vi "Results_file_Plotter.vi"() -> ()   [LabVIEW 2010]
uses:
  Anemometry/Anemometry Sub Vis/Data_plotting_vis/Plot_Slice.ctl
  Anemometry/Anemometry Sub Vis/Data_plotting_vis/Plotter_Mode.ctl
  Anemometry/Anemometry Sub Vis/Data_plotting_vis/Data_File_Type.ctl
  Anemometry/Anemometry Sub Vis/Controls/Global_mode.ctl
  Anemometry/Anemometry Sub Vis/Data_plotting_vis/Results_plotter_Global.vi
  Anemometry/Anemometry Sub Vis/Globals/Constants_global.vi
  Anemometry/Anemometry Sub Vis/Globals/Trav_pos_global.vi
  Instance           1 28Saved   Results_file_Plotter .vi
panel:
  in  "Single Series":i32[](listbox)=[0]
  out "Uadvec":dbl
  in  "Bkgnd Value":dbl
  in  "Update":bool
  in  "Full_Res_Results_Folder":path
  out "Last used Template":path
  out "Cursor index":i32
  in  "Plot Resolution":bool
  out "Choosen Path":path
  out "XY Plot":cluster{dbl[], dbl[]}[](graph)
  in  "VI Refnum Calculation":refnum<vi>
  in  "Save Plot as jpg":bool
  out "Edit Raw Data Header Info":bool
  out "Raw DF in Orig Pos?":bool
  out "Edit Raw DF?":bool
  out "Filetype":string[](array[string])
  out "Mode":T1
  out "Plotted rows only?":bool
  in  "type specifier VI Refnum (for type only) 2":refnum<vi>
  out "Warning!":string
  in  "Edit Template File":bool
  in  "type specifier VI Refnum (for type only)":refnum<vi>
  in  "color and symbol":bool
  out "No Of Rows":i32
  in  "Filter Bins 2":i32[](listbox)=[0]
  in  "Filter 6":u16(ring)
  in  "Filter 5":u16(ring)
  in  "Filter 4":u16(ring) items=["Show All (1216)", "10 (200)", "11 (4)", "13 (4)", "16 (4)", "17 (4)", "20 (12)", "23 (4)", "25 (4)", "28 (4)", "29 (4)", "30 (4)", "31 (4)", "35 (4)", "37 (4)", "38 (4)", "40 (8)", "44 (4)", "45 (8)", "47 (4)", "49 (4)", "50 (192)", "51 (4)", "53 (8)", "54 (4)", "56 (4)", "60 (12)", "63 (4)", "65 (4)", "67 (4)", "71 (8)", "72 (4)", "75 (4)", "78 (4)", "79 (4)", "81 (4)", "82 (4)", "85 (4)", "87 (4)", "90 (12)", "94 (4)", "97 (12)", "99 (4)", "100 (188)", "101 (8)", "103 (4)", "104 (4)", "106 (8)", "110 (4)", "111 (4)", "112 (4)", "115 (4)", "116 (4)", "119 (4)", "121 (8)", "125 (4)", "126 (4)", "128 (8)", "134 (12)", "137 (4)", "139 (4)", "141 (4)", "143 (4)", "144 (4)", "146 (8)", "148 (8)", "149 (4)", "150 (188)", "151 (4)", "153 (8)", "155 (4)", "156 (8)", "160 (4)", "162 (4)", "163 (4)", "164 (4)", "165 (4)", "171 (8)", "172 (4)", "173 (4)", "178 (8)", "181 (4)", "182 (4)", "185 (8)", "191 (8)", "193 (8)", "200 (16)"]
  in  "Filter 3":u16(ring) items=["Show All (1216)", "92 (1216)", "NOT 92 (0)"]
  in  "Filter Array":u16[](array[ring])=[0, 0, 0, 0, 0, 0] items=["Don't Filter", "Filename", "Case", "Roof Height", "Tank Height", "Release Angle", "X", "Y", "Z", "Y (FFID2)", "Z (FFID2)", "Mean Concentration (C)", "Variance in Concentration (C)", "Mean Concentration (C0)", "Variance in Concentration (C0)", "Standard Error in Mean C", "Background Mean Concentration", "Variance in Background Concentration", "CU/Q", "CU/Q err", "x/H", "y/H", "z/H", "Qtrace", "Uref", "Flow Measurement Time", "Seconds since 1st Jan", "Atmos Pressure Used for Corrections", "Current File Number", "Correlation coefficient", "Calib File", "Correlation", "Emission Rate", "Raw Data Filename"]
  in  "Filter Bins 1":i32[](listbox)=[0]
  in  "Tab Control":T2(tab)=enum."Save "
  in  "Reload Files":bool
  in  "Template":path
  in  "Empty":bool
  in  "Result files to read":path[](array[path])
  in  "Add results file":bool
  in  "File Tyoes to Read":T3
  in  "Vector Plot?":bool
  in  "Ordinate Name":string
  out "2nd Add label":string
  out "First Add label":string
  in  "Additional X Values":dbl[](array[numeric]) format="%.2f"
  in  "Additional Y Values":dbl[](array[numeric]) format="%.2f"
  in  "Show Results Space Analysis":bool
  in  "Show Plot Space Analysis":bool
  in  "Multi Ordinate":i32[](listbox)
  in  "Multi Ordinate?":bool
  in  "Ordinate":u16(ring) items=["Filename", "Case", "Roof Height", "Tank Height", "Release Angle", "X", "Y", "Z", "Y (FFID2)", "Z (FFID2)", "Mean Concentration (C)", "Variance in Concentration (C)", "Mean Concentration (C0)", "Variance in Concentration (C0)", "Standard Error in Mean C", "Background Mean Concentration", "Variance in Background Concentration", "CU/Q", "CU/Q err", "x/H", "y/H", "z/H", "Qtrace", "Uref", "Flow Measurement Time", "Seconds since 1st Jan", "Atmos Pressure Used for Corrections", "Current File Number", "Correlation coefficient", "Calib File", "Correlation", "Emission Rate", "Raw Data Filename"]
  in  "Intensity Plot?":bool
  in  "Absisca":u16(ring) items=["Filename", "Case", "Roof Height", "Tank Height", "Release Angle", "X", "Y", "Z", "Y (FFID2)", "Z (FFID2)", "Mean Concentration (C)", "Variance in Concentration (C)", "Mean Concentration (C0)", "Variance in Concentration (C0)", "Standard Error in Mean C", "Background Mean Concentration", "Variance in Background Concentration", "CU/Q", "CU/Q err", "x/H", "y/H", "z/H", "Qtrace", "Uref", "Flow Measurement Time", "Seconds since 1st Jan", "Atmos Pressure Used for Corrections", "Current File Number", "Correlation coefficient", "Calib File", "Correlation", "Emission Rate", "Raw Data Filename"]
  in  "Job Directory":path
  in  "Save Averaged rows":bool
  in  "Create picture Vi Name":string="Intensity plot jpg.vi"
  in  "Save Surface Fit":bool
  in  "Output Filename":path
  in  "Save Data in Rows":bool
  in  "Save Plot data":bool
  in  "Process Point":bool
  in  "Kill Point":bool
  out "Table":string[][](table)
  in  "Post Process Plotted Data":bool
  in  "Calculate Routine":string="Intensity plot jpg.vi"
  in  "Calculate new metadata":bool
  in  "Add /Edit metadata":bool
  in  "Delete Plotted data from file":bool
  in  "Save Setup":bool
  in  "Load Setup":bool
  in  "Point Size":i32(slide) scale=0.0..10.0
  in  "No of Contours":i32=20
  out "Accept Array":bool[][](array[boolean])
  out "Previous slice mode":T4
  out "Slice mode Change?":bool
  in  "Slice mode":T4
  in  "Z Ch Name":u16(ring) items=["Filename", "Case", "Roof Height", "Tank Height", "Release Angle", "X", "Y", "Z", "Y (FFID2)", "Z (FFID2)", "Mean Concentration (C)", "Variance in Concentration (C)", "Mean Concentration (C0)", "Variance in Concentration (C0)", "Standard Error in Mean C", "Background Mean Concentration", "Variance in Background Concentration", "CU/Q", "CU/Q err", "x/H", "y/H", "z/H", "Qtrace", "Uref", "Flow Measurement Time", "Seconds since 1st Jan", "Atmos Pressure Used for Corrections", "Current File Number", "Correlation coefficient", "Calib File", "Correlation", "Emission Rate", "Raw Data Filename"]
  in  "Y Ch Name":u16(ring) items=["Filename", "Case", "Roof Height", "Tank Height", "Release Angle", "X", "Y", "Z", "Y (FFID2)", "Z (FFID2)", "Mean Concentration (C)", "Variance in Concentration (C)", "Mean Concentration (C0)", "Variance in Concentration (C0)", "Standard Error in Mean C", "Background Mean Concentration", "Variance in Background Concentration", "CU/Q", "CU/Q err", "x/H", "y/H", "z/H", "Qtrace", "Uref", "Flow Measurement Time", "Seconds since 1st Jan", "Atmos Pressure Used for Corrections", "Current File Number", "Correlation coefficient", "Calib File", "Correlation", "Emission Rate", "Raw Data Filename"]
  in  "X Ch Name":u16(ring) items=["Filename", "Case", "Roof Height", "Tank Height", "Release Angle", "X", "Y", "Z", "Y (FFID2)", "Z (FFID2)", "Mean Concentration (C)", "Variance in Concentration (C)", "Mean Concentration (C0)", "Variance in Concentration (C0)", "Standard Error in Mean C", "Background Mean Concentration", "Variance in Background Concentration", "CU/Q", "CU/Q err", "x/H", "y/H", "z/H", "Qtrace", "Uref", "Flow Measurement Time", "Seconds since 1st Jan", "Atmos Pressure Used for Corrections", "Current File Number", "Correlation coefficient", "Calib File", "Correlation", "Emission Rate", "Raw Data Filename"]
  out "Filter 2 Strings":string[](array[string])
  out "Filter 1 Strings":string[](array[string])
  out "Ordinate Strings":string[](array[string])
  out "Non-Blank Rows":bool[](array[boolean])
  out "File Index":i32
  in  "Resolution":dbl=1.0 min=0.0 format="%.4f"
  out "Intensity Graph":dbl[][](graph)
  out "Tolerances":dbl[](array[numeric]) format="%.2f"
  in  "Results files choosen":path[](array[path])
  in  "Header":string
  out "Current":string="Graph Scales"
  in  "Transpose":bool
  out "Plotted Series":bool[][](array[boolean])
  in  "Results file":path
  in  "stop":bool
  out "Surface Area":dbl format="%.2f"
  out "Surface Integral":dbl format="%.4f"
  out "Surface Average":dbl format="%#.5f"
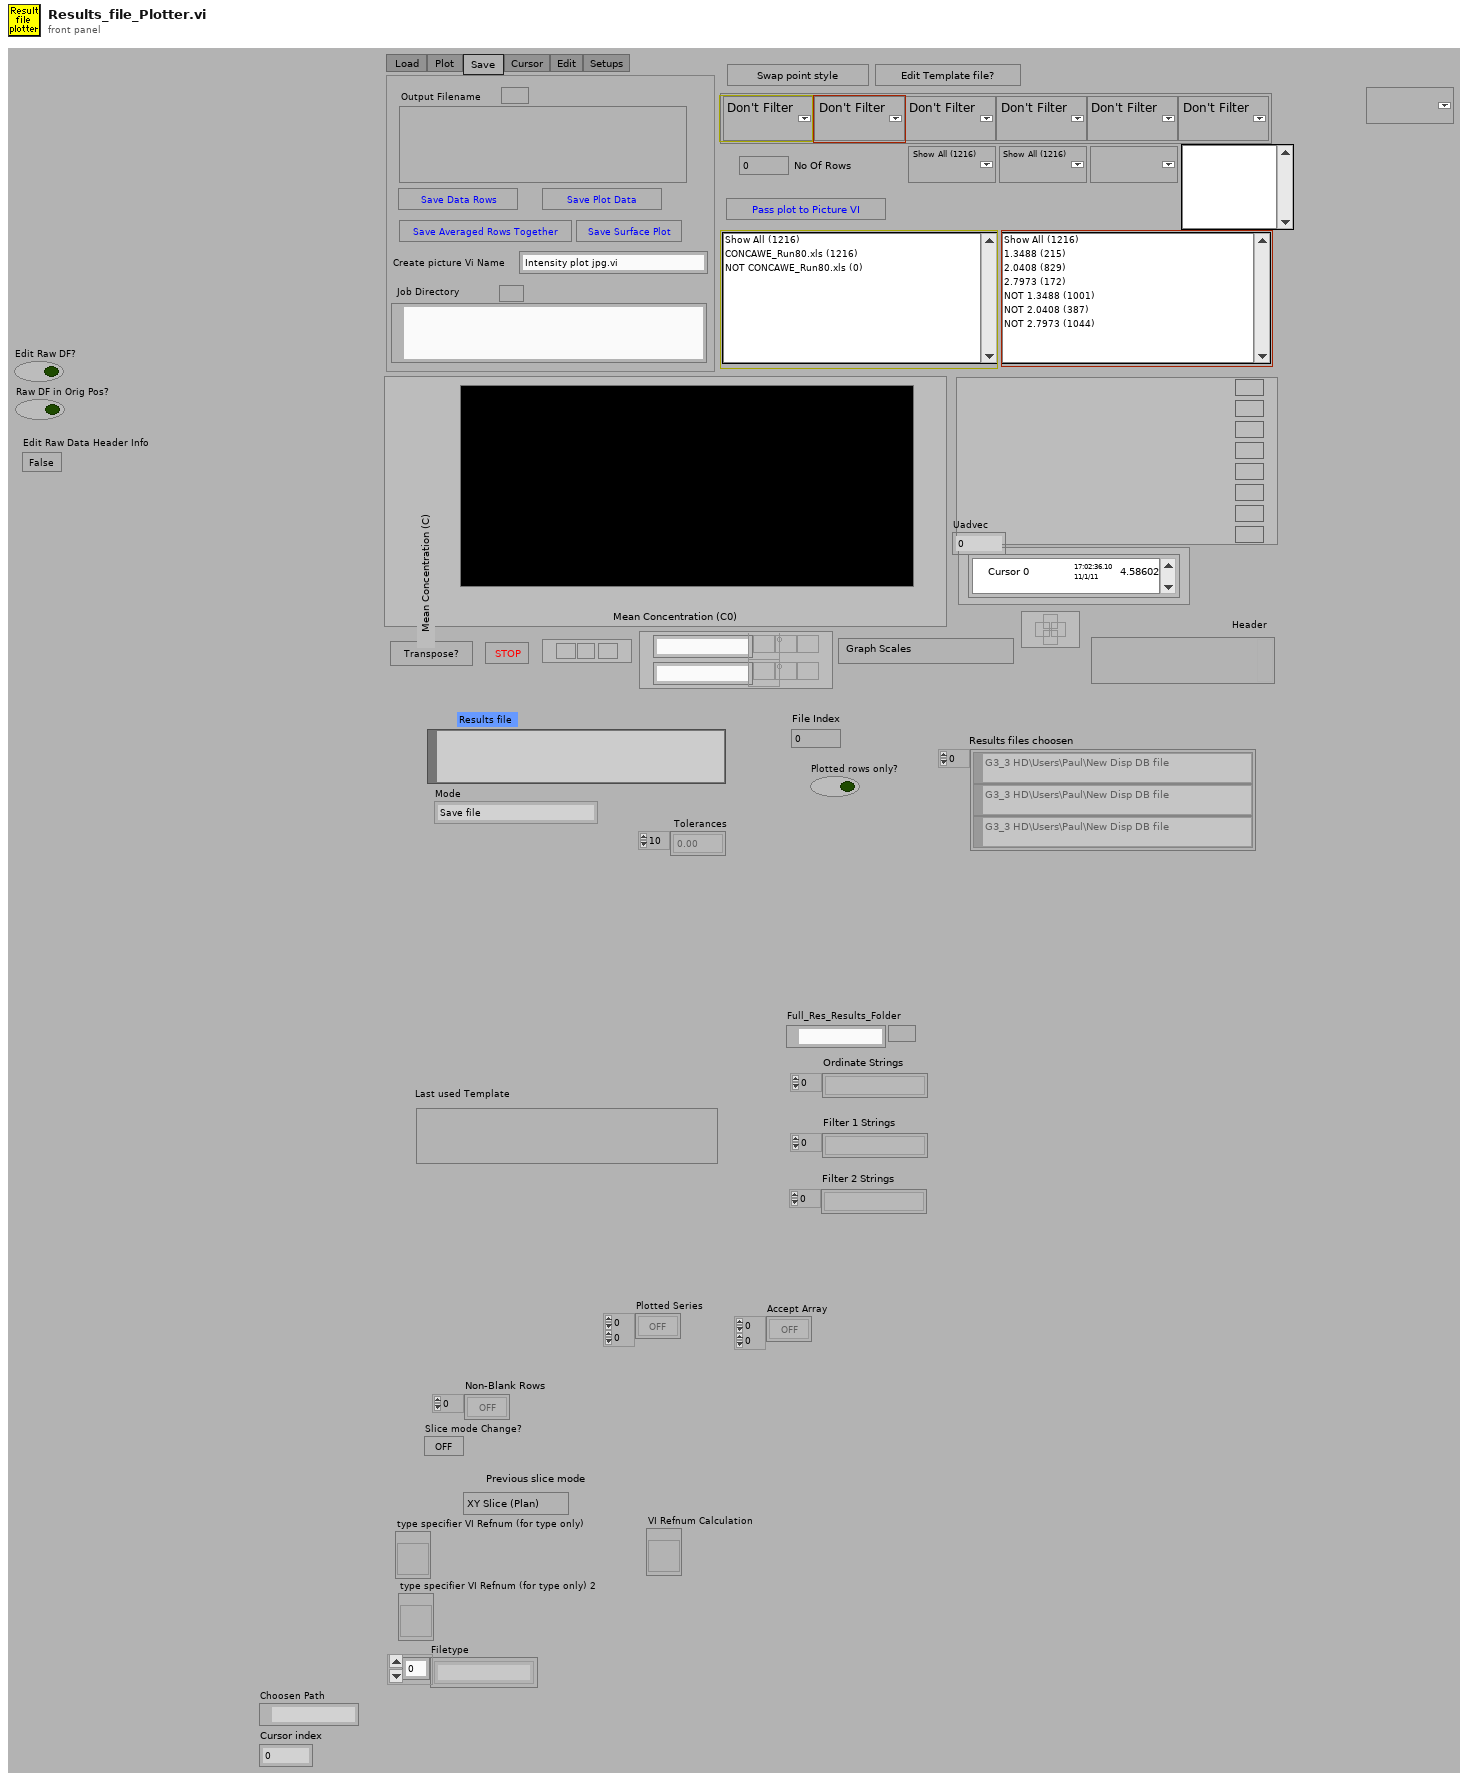
[diagram p1: front panel]
types:
  T1 = typedef "Plotter_Mode.ctl" = enum16{"Save file", "Delete unwanted rows", "Edit Values with constants", "Edit values per row", "Edit Raw Data file header", "Post Process Plotted Rows"}
  T2 = enum32{"Load ", "Plot ", "Save ", "Cursor", "Edit", "Setups"}
  T3 = typedef "Data_File_Type.ctl" = enum16{"Read All File Types", "Results Files Only", "Raw Data Files Only", "Calibration Files Only", "Gas Desk Files Only", "Old Results Files Only", "Tabulated Data Files Only"}
  T4 = typedef "Plot_Slice.ctl" = enum16{"XY Slice (Plan)", "YX Slice (Plan)", "YZ Slice (Cross)", "ZY Slice (Cross)", "XZ Slice (Side)", "ZX Slice (Side)"}
  T5 = enum16{"Zero or one", "One", "Zero or more", "One or more"}
  T6 = typedef "Global_mode.ctl" = enum16{"Read Global", "Load Global From File", "Write Global to File"}
  T7 = enum16{"Edit Existing Template File", "Create New Template File"}
  T8 = enum16{"Show only data summary", "Show data summary", "No data summary"}
  T9 = typedef "All_Setup.ctl" = cluster{"Result files to read":path[], "Template":path, "Transpose":bool, "Additional X Values":dbl[], "Additional Y Values":dbl[], "Ordinate":u16, "Absisca":u16, "Filter Array":u16[], "color and symbol":bool, "Output Filename":path, "Jpg Vi Name":string, "Intensity Plot?":bool, "Multi Ordinate?":bool, "Filter Bins 1":i32[], "Filter Bins 2":i32[], "Multi Ordinate":i32[]}
  T10 = enum16{"Left Button", "Center Button", "Right Button", "Window Close"}
  T11 = enum32{"existing file", "new file", "new or existing file", "existing dir", "new dir", "new or existing dir", "existing file (use LLBs)", "new file (use LLBs)", "new or existing file (use LLBs)", "new or existing file or directory (use LLBs)"}
  T12 = cluster{"Plot Color":u32, "Plot Interpolation":u8, "Point Style":u8, "Line Style":u8, "Fill/Pt. Color":u32, "Line Width":u8, "Bar Plot Style":u8, "Fill To":i16}[]
  T13 = typedef "Group_Binning.ctl" = cluster{"Index":i32, "Tolerance":dbl, "Precision":string}
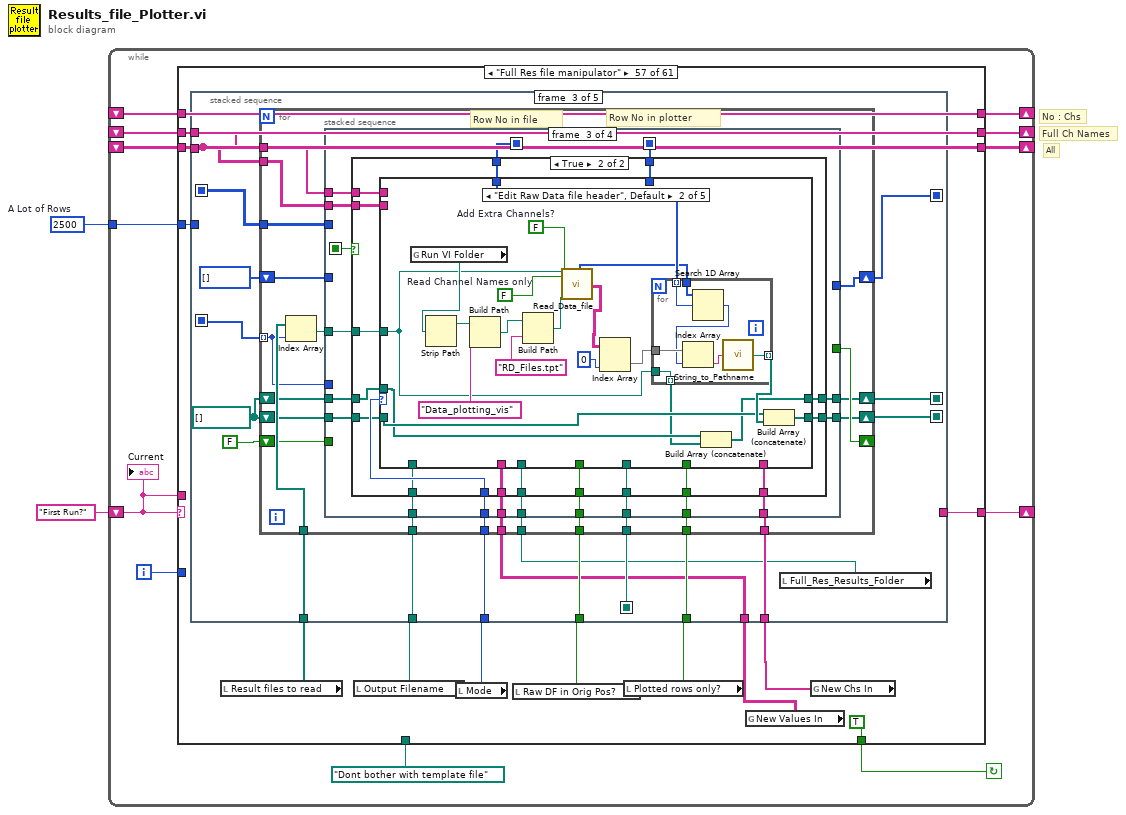
[diagram p0: block diagram]
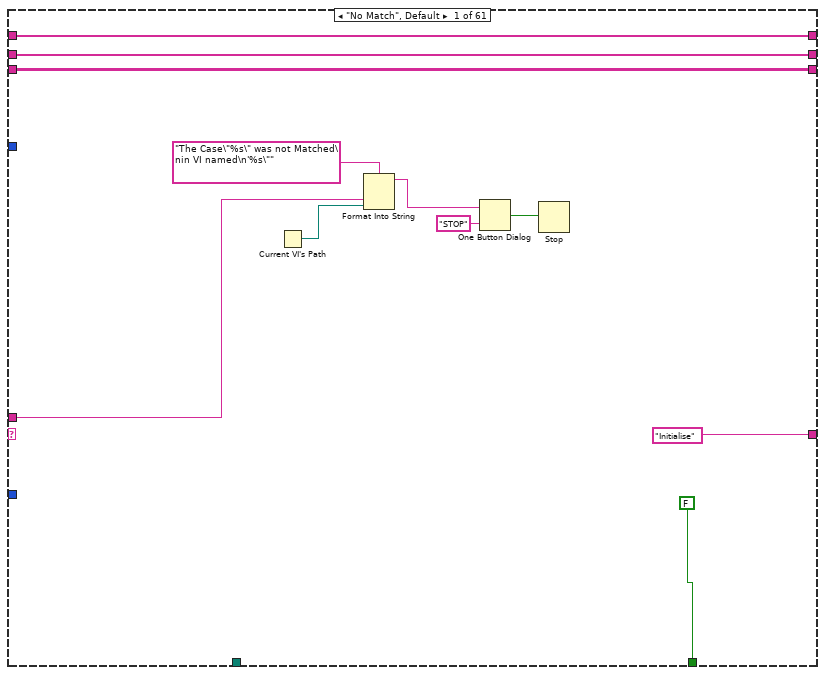
[diagram p2: hidden frame]
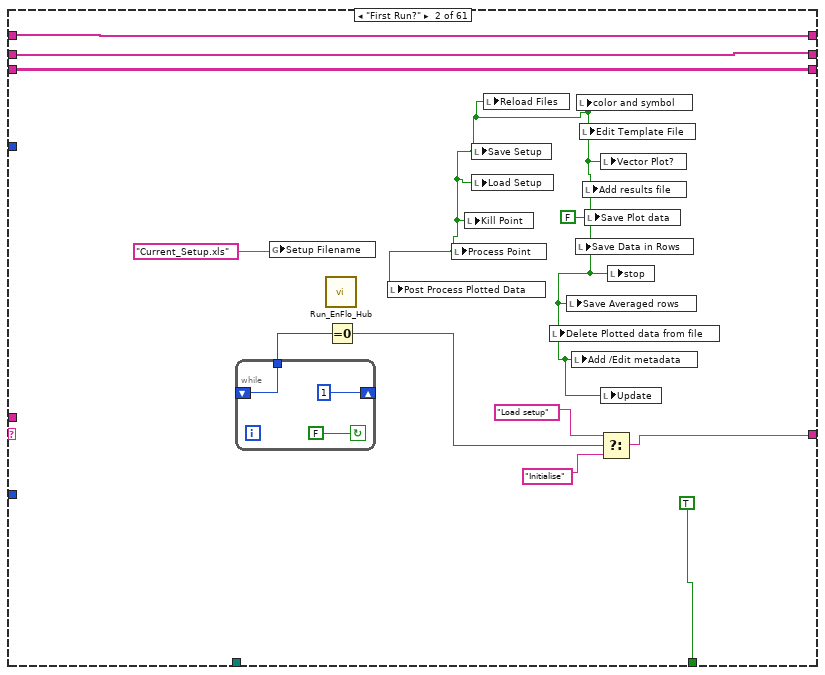
[diagram p3: hidden frame]
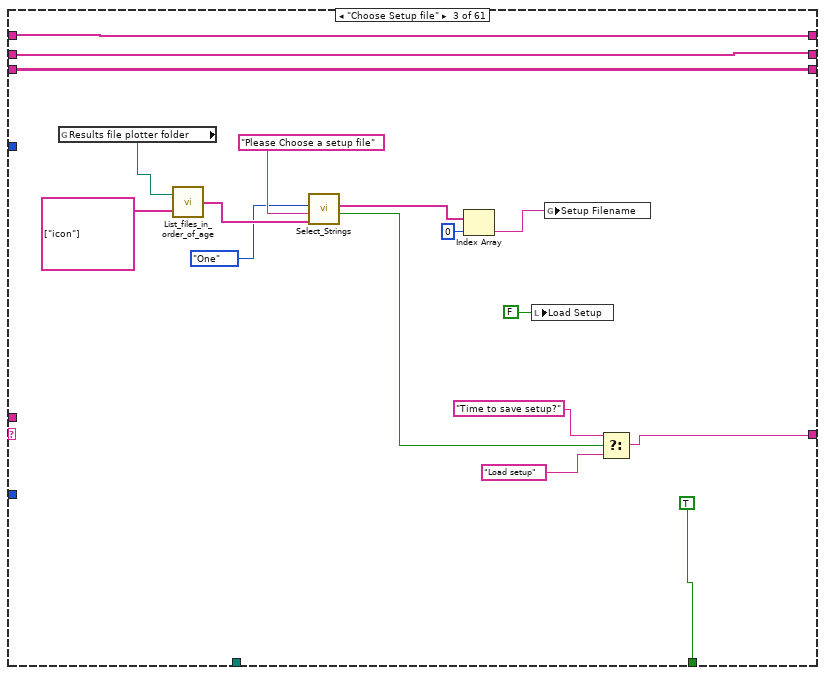
[diagram p4: hidden frame]
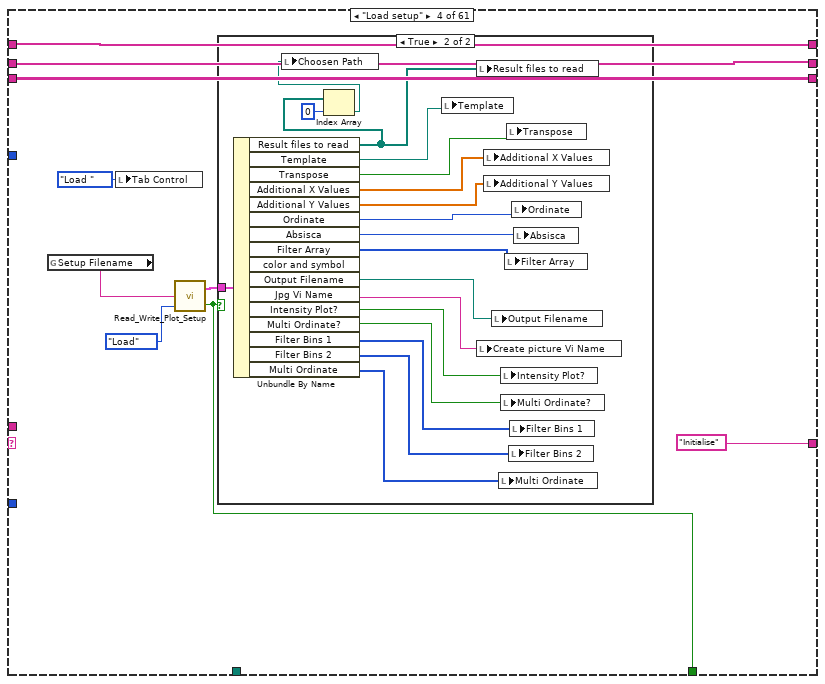
[diagram p5: hidden frame]
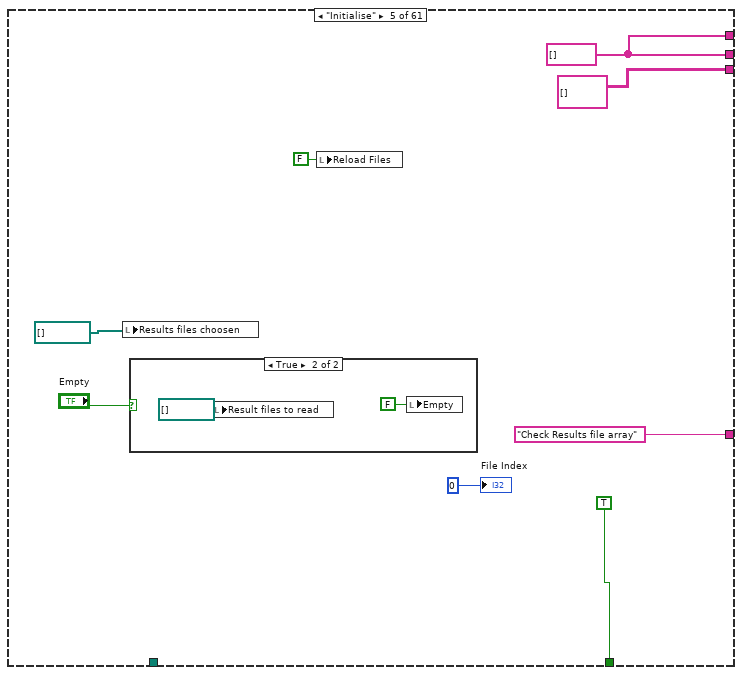
[diagram p7: hidden frame]
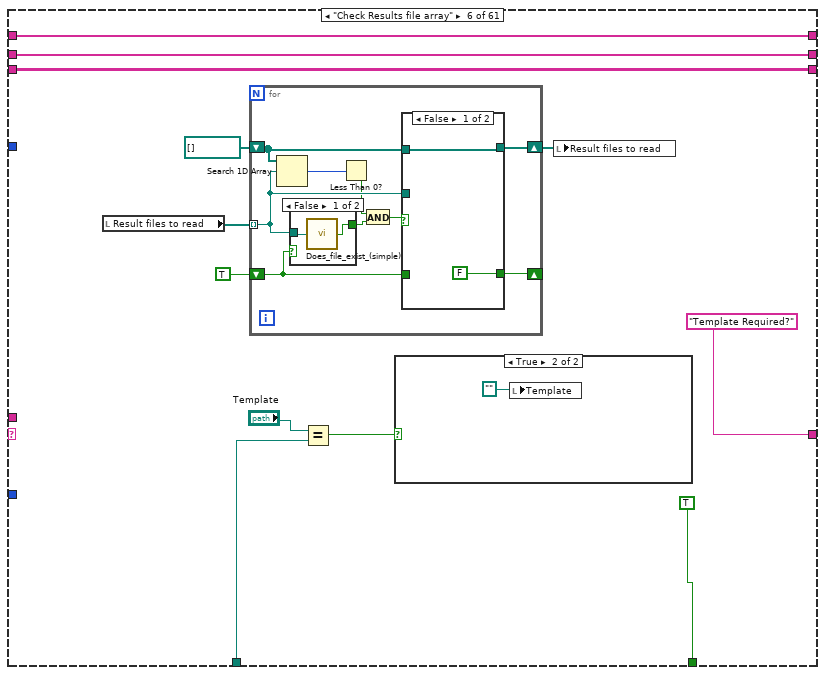
[diagram p9: hidden frame]
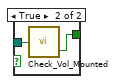
[diagram p11: hidden frame]
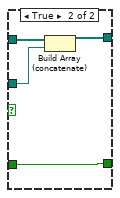
[diagram p12: hidden frame]
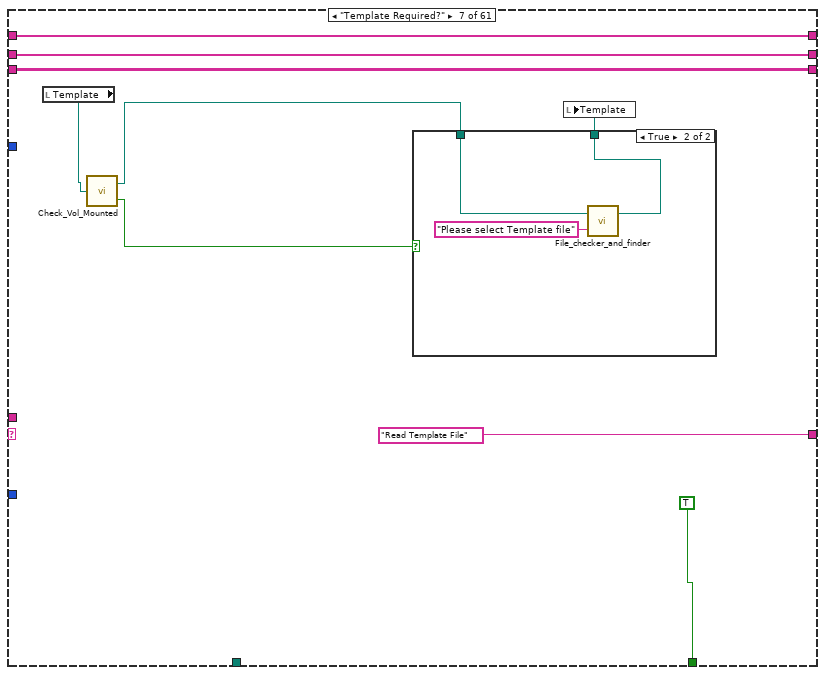
[diagram p13: hidden frame]
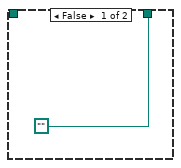
[diagram p14: hidden frame]
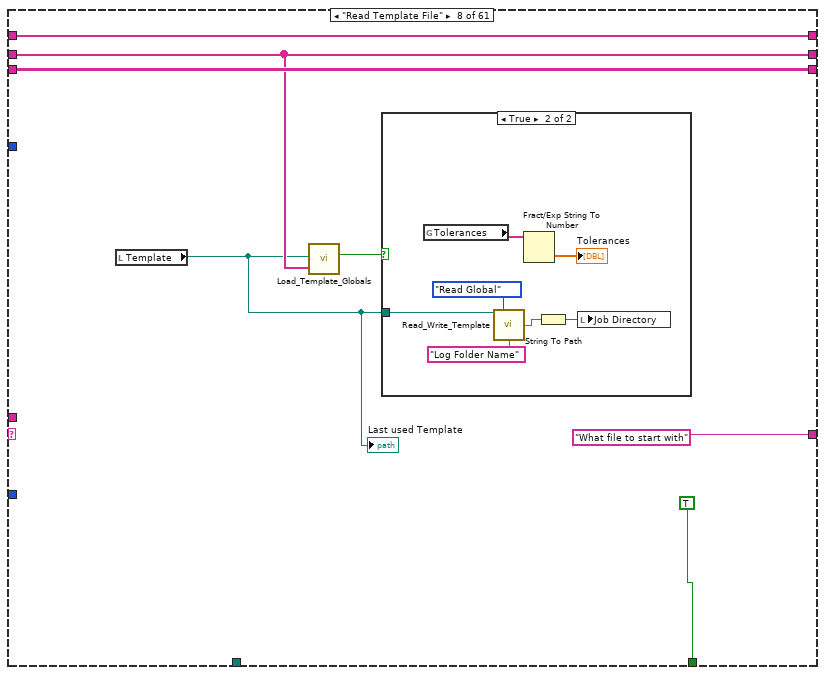
[diagram p15: hidden frame]
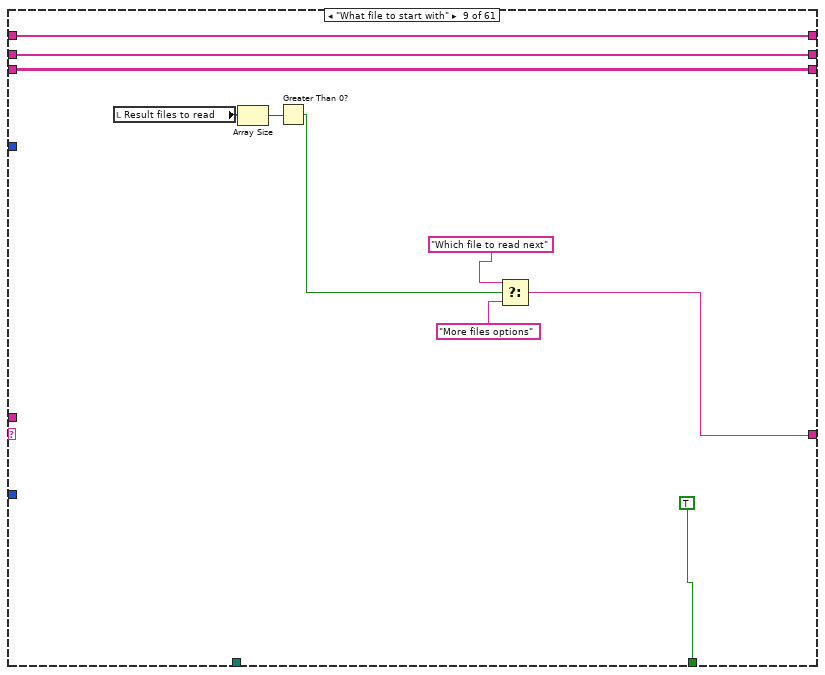
[diagram p17: hidden frame]
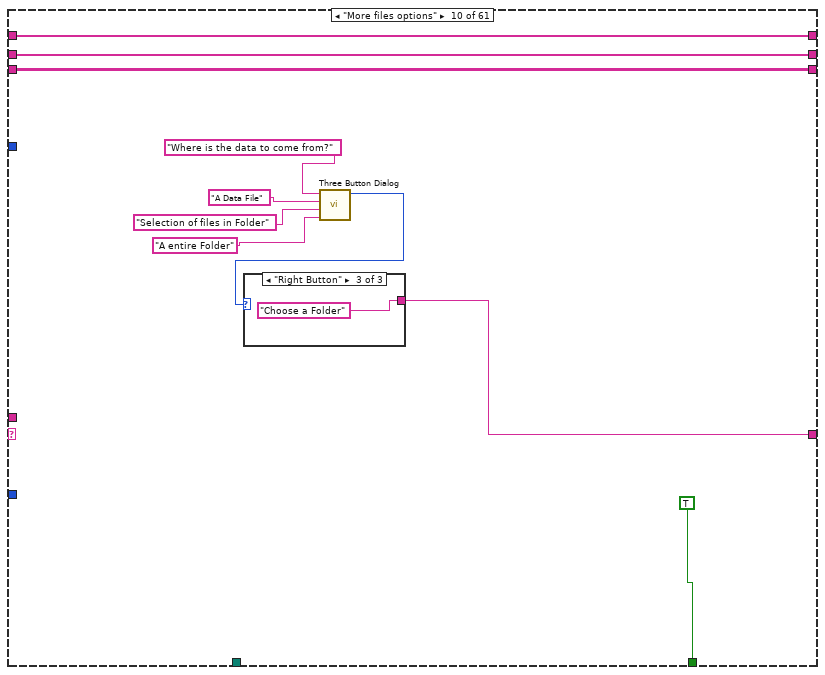
[diagram p18: hidden frame]
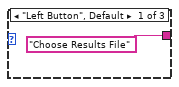
[diagram p19: hidden frame]
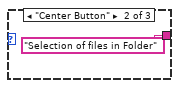
[diagram p20: hidden frame]
diagram:
  w1 = 2500  # A Lot of Rows
  # "No : Chs"
  # "Full Ch Names"
  # "All"
  n1 = while {
    shift-left: _ -> [w7]
    shift-right: [w8] -> _
    shift-left: "First Run?" -> [w11]
    shift-right: [w4] -> _
    shift-left: _ -> [w9]
    shift-right: [w14] -> _
    shift-left: _ -> [w12]
    shift-right: [w5] -> _
    tunnel: w1 -> [w3]
    i -> [w6]
    stop <- w13 continue-if-true
    n2 = case shown="\"Full Res file manipulator\"" w11 {
      tunnel: w9 -> [w25 w35 w55 w63 _ w104 w132 w141 w162 w172 w184 w198 w229 w256 w279 w401 w423 w449 w474 w500 w554 w568 w605 w907 w976 w1031 w1056 w1075 w1161 w1209 w1239 w1528 w1544 w1565 w1594 w1658 w1691 w1763 w1786 w1801 w1865 w1917 w1943 w2152 w2164 w2190 w2316 w2460 w2494 w2509 w2534 w2561 w2604 w2622 w2665 w2768 w2801 w3165 w3180 w3216 w3224]
      tunnel: [w25 w35 w55 w63 w89 w104 w132 w141 w162 w172 w184 w198 w229 w256 w277 w401 w423 w449 w474 w500 w554 w568 w605 w907 w976 w1031 w1056 w1075 w1161 w1209 w1237 w1528 w1544 w1565 w1594 w1658 w1691 w1763 w1786 w1801 w1865 w1917 w1941 w2152 w2164 w2188 w2309 w2460 w2494 w2509 w2534 w2561 w2604 w2622 w2665 w2768 w2801 w3165 w3180 w3216 w3224] -> w14
      tunnel: ["Initialise" w28 w50 "Initialise" ("t") "Check Results file array" ("t") "Template Required?" "Read Template File" "What file to start with" w153 w168 "Which file to read next" "Which file to read next" "Which file to read next" w252 w274 w392 "What is present?" "Ordinate Selector Type" w471 "Which rows are Non-Blank?" w547 "Create Selectors" w594 "Re Plot Data?" w971 "Prepare Filter2 strings" "Plot Data" w1072 "Add Axis names" "Analyse Plot Space" w1240 "What to do next?" "What to do next?" ("t") w1551 w1587 w1636 w1689 w1757 w1782 w1800 w1864 "Initialise" w1944 w2143 "Create Selectors" w2191 w2317 w2458 w2492 w2499 w2518 "Save XY plot as jpg" "Create Selectors" w2619 w2668 w2752 w2807 "Save Setup" ("t") "Initialise" ("t") w3185 "Time to save setup?"] -> w4
      tunnel: [FALSE TRUE TRUE w59 TRUE TRUE TRUE TRUE TRUE TRUE TRUE TRUE TRUE w247 w281 TRUE TRUE TRUE TRUE TRUE TRUE TRUE TRUE TRUE TRUE TRUE TRUE w1073 TRUE TRUE w1241 TRUE TRUE ("OK?") TRUE TRUE ("OK?") TRUE ("OK?") w1687 TRUE TRUE w1799 w1863 TRUE w1945 TRUE ("OK?") TRUE ("OK?") w2192 w2318 TRUE TRUE TRUE TRUE TRUE TRUE TRUE TRUE TRUE TRUE TRUE TRUE w3194 TRUE ("OK?")] -> w13
      tunnel: w12 -> [w24 w34 w54 w62 _ w103 w131 w143 w161 w171 w183 w197 w228 w255 w280 w397 w422 w450 w475 w501 w553 w566 w600 w909 w965 w1033 w1058 w1074 w1163 w1211 w1238 w1527 w1543 w1564 w1605 w1657 w1690 w1762 w1785 w1798 w1862 w1916 w1942 w2151 w2161 w2189 w2315 w2461 w2493 w2508 w2538 w2564 w2603 w2621 w2664 w2767 w2800 w3164 w3179 w3215 w3223]
      tunnel: w11 -> [w16 _ _ _ _ _ _ _ _ _ _ _ _ _ _ _ _ _ _ _ _ _ _ _ _ _ _ _ _ _ _ _ _ _ _ _ _ _ _ _ _ _ _ _ _ _ _ _ _ _ _ _ _ _ _ _ _ _ _ _ _]
      tunnel: path "Dont bother with template file" ("Template File") -> [_ _ _ _ _ w97 _ _ _ _ _ _ _ _ _ _ _ _ _ _ _ _ _ _ _ _ _ _ _ _ _ _ _ _ _ _ _ _ _ _ _ _ _ _ _ _ _ _ _ _ _ _ _ _ _ _ _ w3162 w3174 _ _]
      tunnel: [w15 w33 w53 w64 w89 w102 w130 w142 w159 w169 w181 w195 w226 w254 w276 w385 w421 w451 w473 w499 w545 w567 w598 w906 w967 w1023 w1051 w1071 w1155 w1204 w1233 w1524 w1545 w1563 w1595 w1659 w1692 w1761 w1784 w1797 w1861 w1915 w1935 w2153 w2169 w2179 w2312 w2470 w2495 w2510 w2535 w2562 w2605 w2623 w2669 w2769 w2808 w3166 w3181 w3217 w3225] -> w8
      tunnel: w7 -> [w15 w33 w53 w64 _ w102 w130 w142 w159 w169 w181 w195 w226 w254 w275 w385 w421 w451 w473 w499 w545 w567 w598 w906 w967 w1023 w1051 w1071 w1155 w1204 w1232 w1524 w1545 w1563 w1595 w1659 w1692 w1761 w1784 w1797 w1861 w1915 w1934 w2153 w2169 w2183 w2311 w2470 w2495 w2510 w2535 w2562 w2605 w2623 w2669 w2769 w2808 w3166 w3181 w3217 w3225]
      tunnel: w6 -> [_ _ _ _ _ _ _ _ _ _ _ _ _ _ _ _ _ _ _ _ _ _ _ _ _ _ _ _ _ _ _ _ _ _ _ _ w1688 _ _ _ _ _ _ _ _ _ _ _ _ _ _ _ _ _ _ _ _ _ _ _ _]
      tunnel: [w24 w34 w54 w62 string[][] [] w103 w131 w143 w161 w171 w183 w197 w228 w255 w278 w397 w422 w450 w475 w501 w553 w566 w600 w909 w965 w1033 w1058 w1074 w1163 w1211 w1236 w1527 w1543 w1564 w1605 w1657 w1690 w1762 w1785 w1798 w1862 w1916 w1940 w2151 w2161 w2187 w2308 w2461 w2493 w2508 w2538 w2564 w2603 w2621 w2664 w2767 w2800 w3164 w3179 w3215 w3223] -> w5
      tunnel: w3 -> [_ _ _ _ _ _ _ _ _ _ _ _ _ _ _ _ _ _ _ _ _ _ _ _ _ _ _ _ _ _ _ _ _ _ _ _ _ _ w1780 _ w1860 _ _ _ _ _ _ _ _ _ _ _ _ w2618 w2662 _ w2798 _ _ _ _]
      frame "No Match", Default {
        n3 = Current VI's Path() -> (path=w17:path)
        n4 = Format Into String(format string="The Case\"%s\" was not Matched\nin VI named\n'%s\"" ("Format String"), w16, w17) -> (resulting string=w20:string)  [unwired: 2 in, 1 out]
        n5 = One Button Dialog(message=w20, button name ("OK")="STOP") -> (true=w18:bool)
        n6 = Stop(stop? (T)=w18) -> ()
      }
      frame "First Run?" {
        w26 = FALSE ("Save Plot data")
        n7 = while {
          shift-right: [1] -> _
          shift-left: _ -> [w38]
          tunnel: [w38] -> w30
          stop <- FALSE continue-if-true
        }
        n8 = global write "Results_plotter_Global.vi" "Setup Filename"("Current_Setup.xls" ("Setup filename")) -> ()
        n9 = call "Run_EnFlo_Hub.vi"() -> ()  [unwired: 8 out]
        n10 = Equal To 0?(x=w30) -> (x = 0?=w29:bool)
        n11 = local write "Post Process Plotted Data"(w26) -> ()
        n12 = local write "Process Point"(w26) -> ()
        n13 = local write "Kill Point"(w26) -> ()
        n14 = local write "Save Setup"(w26) -> ()
        n15 = local write "Load Setup"(w26) -> ()
        n16 = local write "Reload Files"(w26) -> ()
        n17 = local write "Delete Plotted data from file"(w26) -> ()
        n18 = local write "Save Averaged rows"(w26) -> ()
        n19 = local write "Add /Edit metadata"(w26) -> ()
        n20 = local write "Save Data in Rows"(w26) -> ()
        n21 = local write "color and symbol"(w26) -> ()
        n22 = local write "Edit Template File"(w26) -> ()
        n23 = local write "Add results file"(w26) -> ()
        n24 = local write "Save Plot data"(w26) -> ()
        n25 = local write "Vector Plot?"(w26) -> ()
        n26 = local write "Update"(w26) -> ()
        n27 = Select(t="Load setup", s=w29, f="Initialise") -> (s? t:f=w28:string)
        n28 = local write "stop"(w26) -> ()
      }
      frame "Choose Setup file" {
        n29 = global read "Constants_global.vi" "Results file plotter folder"() -> (w49:path)
        n30 = call "List_files_in_order_of_age.vi"("Files to Hide"=string[] ["icon"], "Folder"=w49) -> ("file names"=w48:string[])
        n31 = call "Select_Strings.vi"("Available Ch names"=w48, "Message"="Please Choose a setup file", "Selector mode"=T5."One") -> ("Cancel"=w42:bool, "Selected Channel Names"=w45:string[])  [unwired: 1 in, 3 out]
        n32 = Index Array(array=w45, index=0) -> (element=w43:string)
        n33 = local write "Load Setup"(FALSE ("Save Setup")) -> ()
        n34 = global write "Results_plotter_Global.vi" "Setup Filename"(w43) -> ()
        n35 = Select(t="Time to save setup?", s=w42, f="Load setup") -> (s? t:f=w50:string)
      }
      frame "Load setup" {
        n36 = global read "Results_plotter_Global.vi" "Setup Filename"() -> (w58:string)
        n37 = local write "Tab Control"(T2."Load " ("Tab Control")) -> ()
        n38 = call "Read_Write_Plot_Setup.vi"("Mode"=enum16{"Load", "Save"}."Load", "Setup filename"=w58) -> ("OK?"=w59:bool, "Cluster 2"=w60:T9)  [unwired: 1 in]
        n39 = case shown="True" w59 {
          tunnel: w60 -> [_ w83]
          frame False {
          }
          frame True {
            n40 = Unbundle By Name(w83) -> ("Result files to read"=w68:path[], "Template"=w66:path, "Transpose"=w73:bool, "Additional X Values"=w74:dbl[], "Additional Y Values"=w75:dbl[], "Ordinate"=w76:u16, "Absisca"=w77:u16, "Filter Array"=w78:u16[], "Output Filename"=w79:path, "Jpg Vi Name"=w80:string, "Intensity Plot?"=w81:bool, "Multi Ordinate?"=w82:bool, "Filter Bins 1"=w72:i32[], "Filter Bins 2"=w71:i32[], "Multi Ordinate"=w70:i32[])  [unwired: 1 out]
            n41 = Index Array(array=w68, index=0) -> (element=w67:path)
            n42 = local write "Choosen Path"(w67) -> ()
            n43 = local write "Template"(w66) -> ()
            n44 = local write "Result files to read"(w68) -> ()
            n45 = local write "Create picture Vi Name"(w80) -> ()
            n46 = local write "Additional X Values"(w74) -> ()
            n47 = local write "Additional Y Values"(w75) -> ()
            n48 = local write "Output Filename"(w79) -> ()
            n49 = local write "Multi Ordinate"(w70) -> ()
            n50 = local write "Intensity Plot?"(w81) -> ()
            n51 = local write "Multi Ordinate?"(w82) -> ()
            n52 = local write "Filter Array"(w78) -> ()
            n53 = local write "Transpose"(w73) -> ()
            n54 = local write "Filter Bins 2"(w71) -> ()
            n55 = local write "Filter Bins 1"(w72) -> ()
            n56 = local write "Ordinate"(w76) -> ()
            n57 = local write "Absisca"(w77) -> ()
          }
        }
      }
      frame "Initialise" {
        w89 = string[] [] ("Channel names")
        n58 = local write "Results files choosen"(path[] [] ("Results file choosen")) -> ()
        n59 = case shown="True" "Empty" {
          frame False {
          }
          frame True {
            n60 = local write "Result files to read"(path[] [] ("Result files to read")) -> ()
            n61 = local write "Empty"(FALSE ("Empty")) -> ()
          }
        }
        n62 = local write "Reload Files"(FALSE ("Reload Files")) -> ()
        "File Index" <- 0
      }
      frame "Check Results file array" {
        n63 = local read "Result files to read"() -> (w101:path[])
        n64 = for {
          shift-right: [w115] -> w99
          shift-left: path[] [] -> [w114]
          tunnel: w101 -> [w113] mode=indexing
          shift-right: [w108] -> _
          shift-left: TRUE -> [w107]
          n65 = Search 1D Array(1D array=w114, element=w113) -> (index of element=w112:i32)  [unwired: 1 out]
          n66 = case shown="False" w107 {
            tunnel: w113 -> [w117 w119]
            tunnel: [w116 w118] -> w110
            frame False {
              n67 = call "Does_file_exist_(simple).vi"("Pathname"=w117) -> ("exists?"=w116:bool)
            }
            frame True {
              n68 = call "Check_Vol_Mounted.vi"("Filename"=w119) -> ("exists?"=w118:bool)  [unwired: 1 out]
            }
          }
          n69 = Less Than 0?(x=w112) -> (x < 0?=w109:bool)
          n70 = And(x=w109, y=w110) -> (x .and. y?=w111:bool)
          n71 = case shown="False" w111 {
            tunnel: w114 -> [w121 w125]
            tunnel: w113 -> [_ w124]
            tunnel: [w121 w123] -> w115
            tunnel: [FALSE w122] -> w108
            tunnel: w107 -> [_ w122]
            frame False {
            }
            frame True {
              n72 = Build Array (concatenate)(w125, w124) -> (w123:path[])
            }
          }
        }
        n73 = Equal?(x="Template", y=w97) -> (x = y?=w96:bool)
        n74 = case shown="True" w96 {
          frame False {
          }
          frame True {
            n75 = local write "Template"(path "") -> ()
          }
        }
        n76 = local write "Result files to read"(w99) -> ()
      }
      frame "Template Required?" {
        n77 = local read "Template"() -> (w129:path)
        n78 = call "Check_Vol_Mounted.vi"("Filename"=w129) -> ("Filename Out"=w128:path, "exists?"=w127:bool)
        n79 = case shown="True" w127 {
          tunnel: w128 -> [_ w137]
          tunnel: [path "" w136] -> w126
          frame False {
          }
          frame True {
            n80 = call "File_checker_and_finder.vi"("Promp if not found"="Please select Template file", "Filename In"=w137) -> ("Filename Out"=w136:path)  [unwired: 1 out]
          }
        }
        n81 = local write "Template"(w126) -> ()
      }
      frame "Read Template File" {
        n82 = local read "Template"() -> (w139:path)
        "Last used Template" <- w139
        n83 = call "Load_Template_Globals.vi"("Channel Names"=w141, "Template-read"=w139) -> ("Valid Template File?"=w140:bool)
        n84 = case shown="True" w140 {
          tunnel: w139 -> [_ w147]
          frame False {
          }
          frame True {
            n85 = global read "Results_plotter_Global.vi" "Tolerances"() -> (w151:string[])
            n86 = call "Read_Write_Template.vi"("Template File"=w147, "Mode"=Global_mode."Read Global", "Data type"="Log Folder Name" ("Variable name")) -> ("Single Value Out"=w149:string)  [unwired: 5 in, 7 out]
            n87 = Fract/Exp String To Number(string=w151) -> (number=→"Tolerances":dbl[])  [unwired: 4 out]
            n88 = String To Path(string=w149) -> (path=w146:path)
            n89 = local write "Job Directory"(w146) -> ()
          }
        }
      }
      frame "What file to start with" {
        n90 = local read "Result files to read"() -> (w158:path[])
        n91 = Array Size(array=w158) -> (size(s)=w157:i32)
        n92 = Greater Than 0?(x=w157) -> (x > 0?=w154:bool)
        n93 = Select(t="Which file to read next", s=w154, f="More files options") -> (s? t:f=w153:string)
      }
      frame "More files options" {
        n94 = call <vilib>:"Three Button Dialog.vi"("Right Button Text (\"Cancel\")"="A entire Folder" ("F button name (\"Cancel\")"), "Center Button Text (\"No\")"="Selection of files in Folder" ("T button name (\"OK\")"), "Left Button Text (\"Yes\")"="A Data File" ("T button name (\"OK\")"), "message"="Where is the data to come from?") -> ("Which Button?"=w167:T10)  [unwired: 1 in, 6 out]
        n95 = case shown="\"Right Button\"" w167 {
          tunnel: ["Choose Results File" "Selection of files in Folder" "Choose a Folder"] -> w168
          frame "Left Button", Default {
          }
          frame "Center Button" {
          }
          frame "Right Button" {
          }
        }
      }
      frame "Choose Results File" {
        (unwired) T11."existing file" ("select mode (2)")
        n96 = local read "Choosen Path"() -> (w176:path)
        n97 = File Dialog(7:"Please Choose a Results File" ("Promp if not found"), 11:w176) -> (1:w178:bool, 3:w177:path)  [unwired: 1 in, 6 out]
        "Choosen Path" <- w177
        n98 = case shown="False" w178 {
          tunnel: w177 -> [w185 _]
          frame False {
            n99 = local read "Result files to read"() -> (w186:path[])
            n100 = Build Array (concatenate)(w186, w185) -> (w187:path[])
            n101 = local write "Result files to read"(w187) -> ()
          }
          frame True {
          }
        }
      }
      frame "Choose a Folder" {
        n102 = local read "Choosen Path"() -> (w189:path)
        n103 = File Dialog(7:"Please Choose the folder that contains the Results files to be plotted" ("prompt"), 11:w189) -> (3:w188:path)  [unwired: 1 in, 7 out]
        n104 = local write "Choosen Path"(w188) -> ()
        n105 = call "Get_folder_and_filenames.vi"("file path (dialog if empty)"=w188) -> ("Files"=w190:path[])  [unwired: 1 out]
        n106 = for {
          shift-right: [w209] -> w191
          shift-left: "Result files to read" -> [w208]
          tunnel: w190 -> [w206] mode=indexing
          n107 = Search 1D Array(1D array=w208, element=w206) -> (index of element=w207:i32)  [unwired: 1 out]
          n108 = Strip Path(path=w206) -> (name=w205:string)  [unwired: 1 out]
          n109 = Less Than 0?(x=w207) -> (x < 0?=w204:bool)
          n110 = call "Add_filename_suffix.vi"("Filename"=w205) -> ("Original Suffix"=w202:string)  [unwired: 1 in, 3 out]
          n111 = call "Match_Pat_Case_In.vi"("String to match"=".jpg" ("x"), "String"=w202) -> ("offset past match"=w200:i32)  [unwired: 1 in, 3 out]
          n112 = Less Than 0?(x=w200) -> (x < 0?=w199:bool)
          n113 = And(x=w204, y=w199) -> (x .and. y?=w203:bool)
          n114 = case shown="True" w203 {
            tunnel: w208 -> [w210 w213]
            tunnel: w206 -> [_ w212]
            tunnel: [w210 w211] -> w209
            frame False {
            }
            frame True {
              n115 = Build Array (concatenate)(w213, w212) -> (w211:path[])
            }
          }
        }
        n116 = local write "Result files to read"(w191) -> ()
      }
      frame "Selection of files in Folder" {
        n117 = local read "Choosen Path"() -> (w215:path)
        n118 = local read "Result files to read"() -> (w218:path[])
        n119 = File Dialog(7:"Please Choose the folder that contains the Results files to be plotted" ("prompt"), 11:w215) -> (3:w214:path)  [unwired: 1 in, 7 out]
        n120 = local write "Choosen Path"(w214) -> ()
        n121 = call "Get_folder_and_filenames.vi"("file path (dialog if empty)"=w214) -> ("Files"=w220:path[])  [unwired: 1 out]
        n122 = for {
          tunnel: w220 -> [w243] mode=indexing
          tunnel: [w242] -> w223 mode=indexing
          n123 = Strip Path(path=w243) -> (name=w242:string)  [unwired: 1 out]
        }
        n124 = call "Select_Strings.vi"("Available Ch names"=w223, "Message"="Please select the desired data files", "Selector mode"=T5."Zero or more") -> ("Ch Indicies Choosen"=w221:i32[])  [unwired: 1 in, 4 out]
        n125 = for {
          tunnel: w221 -> [w241] mode=indexing
          tunnel: w220 -> [w240]
          tunnel: [w239] -> w216 mode=indexing
          n126 = Index Array(array=w240, index=w241) -> (element=w239:path)
        }
        n127 = for {
          shift-right: [w234] -> w217
          shift-left: w218 -> [w233]
          tunnel: w216 -> [w232] mode=indexing
          n128 = Search 1D Array(1D array=w233, element=w232) -> (index of element=w231:i32)  [unwired: 1 out]
          n129 = Less Than 0?(x=w231) -> (x < 0?=w230:bool)
          n130 = case shown="True" w230 {
            tunnel: w233 -> [w235 w238]
            tunnel: w232 -> [_ w237]
            tunnel: [w235 w236] -> w234
            frame False {
            }
            frame True {
              n131 = Build Array (concatenate)(w238, w237) -> (w236:path[])
            }
          }
        }
        n132 = local write "Result files to read"(w217) -> ()
      }
      frame "Which file to read next" {
        n133 = local read "Result files to read"() -> (w253:path[])
        n134 = local read "File Index"() -> (w250:i32)
        n135 = Array Size(array=w253) -> (size(s)=w251:i32)
        n136 = Equal?(x=w251, y=w250) -> (x = y?=w249:bool)
        n137 = case shown="True" w249 {
          tunnel: w253 -> [w259 _]
          tunnel: [w260 "Load Selectors"] -> w252
          tunnel: w250 -> [w258 w272]
          tunnel: [w257 w272] -> w245
          frame False {
            n138 = Index Array(array=w259, index=w258) -> (element=w261:path)
            n139 = Search 1D Array(1D array="Results files choosen", element=w261) -> (index of element=w263:i32)  [unwired: 1 out]
            n140 = local write "Results file"(w261) -> ()
            n141 = call "Add_filename_suffix.vi"() -> ()  [unwired: 2 in, 4 out]
            n142 = case shown="-1" w263 {
              tunnel: "Results files choosen" -> [_ w271]
              tunnel: w261 -> [w267 w270]
              tunnel: ["Which file to read next" "Load Data"] -> w260
              frame 0, Default {
                n143 = Format Into String(format string="The filename\n \"%s\"\n has already been choosen" ("Format String"), w267) -> (resulting string=w265:string)  [unwired: 2 in, 1 out]
                n144 = One Button Dialog(message=w265) -> ()  [unwired: 2 out]
              }
              frame -1 {
                n145 = Build Array (concatenate)(w271, w270) -> (w269:path[])
                n146 = local write "Results files choosen"(w269) -> ()
              }
            }
            n147 = Increment(x=w258) -> (x+1=w257:i32)
          }
          frame True {
          }
        }
        n148 = Decrement(x=w245) -> (x-1=w244:i32)
        n149 = Build Array(w244) -> (w246:i32[])
        n150 = local read "stop"() -> (w248:bool)
        n151 = local write "File Index"(w245) -> ()
        n152 = property on="Result files to read" class="Arr (strict)"("Index Values"=w246) -> ()  [unwired: 2 in, 2 out]
        n153 = Not(x=w248) -> (.not. x?=w247:bool)
      }
      frame "Load Data" {
        n154 = stacked-sequence {
          seq-local: [w286 _] -> [_ w346]
          seq-local: [w285 _] -> [_ w351]
          seq-local: [w284 _] -> [_ w350]
          seq-local: [w282 _] -> [_ w349]
          tunnel: [TRUE _] -> w281
          tunnel: w280 -> [w300 w352]
          tunnel: w279 -> [w299 _]
          tunnel: [w298 _] -> w278
          tunnel: [w297 _] -> w277
          tunnel: [w296 _] -> w276
          tunnel: w275 -> [w295 _]
          tunnel: ["Which file to read next" _] -> w274
          frame #0 {
            w289 = TRUE  # Add Extra Channels?
            n155 = local read "Template"() -> (w293:path)
            n156 = call "Read_Data_file.vi"("Results file"="Results file", "Add Extra Channels?"=w289, "Template File"=w293, "Desired File Types"="File Tyoes to Read") -> ("Row numbers"=w284:i32[], "Template File Out"=w290:path, "Filetype"=w285:string, "Results file Out"=w286:path, "Ch names Out"=w291:string[], "Channel Values Out"=w287:string[][])  [unwired: 1 in, 9 out]
            n157 = local write "Template"(w290) -> ()
            n158 = Array Size(array=w291) -> (size(s)=w292:i32)
            n159 = Greater Than 0?(x=w292) -> (x > 0?=w282:bool)
            n160 = case shown="True" w282 {
              tunnel: w300 -> [w303 w316]
              tunnel: w299 -> [w304 w308]
              tunnel: w287 -> [_ w306]
              tunnel: [w303 w309] -> w298
              tunnel: [w304 w314] -> w297
              tunnel: [w302 w313] -> w296
              tunnel: w295 -> [w302 _]
              tunnel: w291 -> [_ w307]
              frame False {
              }
              frame True {
                n161 = for {
                  tunnel: w306 -> [w318] mode=indexing
                  tunnel: [w317] -> w305 mode=indexing
                  n162 = for {
                    tunnel: w318 -> [w320] mode=indexing
                    tunnel: [w319] -> w317 mode=indexing
                    n163 = call "Fast_string_Replace.vi"("Replace match with:"="[", "Input String"=w320, "regular expression"="(") -> ("Output String"=w321:string)  [unwired: 2 out]
                    n164 = call "Fast_string_Replace.vi"("Replace match with:"="]", "Input String"=w321, "regular expression"=")") -> ("Output String"=w319:string)  [unwired: 2 out]
                  }
                }
                n165 = call "Merge_channel_names.vi"("Preferred Channel array"=w308, "Channel array"=w307) -> ("Merged Channels"=w314:string[], "Preferred Channels Changed?"=w311:bool, "Channel Array Changed?"=w312:bool)
                n166 = for {
                  tunnel: w314 -> [w343] mode=indexing
                  tunnel: [w340] -> w313 mode=indexing
                  n167 = call "Fast_string_Replace.vi"("Replace match with:"=" ", "Input String"=w343, "regular expression"=":") -> ("Output String"=w339:string)  [unwired: 2 out]
                  n168 = call "Fast_string_Replace.vi"("Replace match with:"=" ", "Input String"=w339, "regular expression"="  ") -> ("Output String"=w338:string)  [unwired: 2 out]
                  n169 = call <vilib>:"Trim Whitespace.vi"("string"=w338) -> ("trimmed string"=w340:string)  [unwired: 1 in]
                }
                n170 = case shown="True" w311 {
                  tunnel: w316 -> [w331 w333]
                  tunnel: w308 -> [_ w335]
                  tunnel: [w331 w332] -> w310
                  tunnel: w314 -> [_ w334]
                  frame False {
                  }
                  frame True {
                    n171 = call "Merge_2D_values.vi"("Values In"=w333, "Present Channels"=w335, "Desired Channels"=w334) -> ("Values Out"=w332:string[][])
                  }
                }
                n172 = case shown="True" w312 {
                  tunnel: [w326 w330] -> w315
                  tunnel: w307 -> [_ w329]
                  tunnel: w305 -> [w326 w328]
                  tunnel: w314 -> [_ w327]
                  frame False {
                  }
                  frame True {
                    n173 = call "Merge_2D_values.vi"("Values In"=w328, "Present Channels"=w329, "Desired Channels"=w327) -> ("Values Out"=w330:string[][])
                  }
                }
                n174 = Build Array (concatenate)(w310, w315) -> (w309:string[][])
              }
            }
          }
          frame #1 {
            n175 = local read "Result files to read"() -> (w345:path[])
            n176 = local read "File Index"() -> (w348:i32)
            n177 = Decrement(x=w348) -> (x-1=w347:i32)
            n178 = case shown="True" w349 {
              tunnel: w352 -> [_ w365]
              tunnel: w351 -> [_ w363]
              tunnel: w350 -> [_ w361]
              tunnel: w347 -> [w353 w359]
              tunnel: w346 -> [_ w358]
              tunnel: w345 -> [w355 w360]
              tunnel: [w354 w357] -> w344
              frame False {
                n179 = Delete From Array(array=w355, length=1, index=w353) -> (array with subset deleted=w354:path[])  [unwired: 1 out]
                n180 = local write "File Index"(w353) -> ()
              }
              frame True {
                n181 = Array Size(array=w365) -> (size(s)=w367:i32[])
                n182 = Index Array(array=w367, index=0 ("Index")) -> (element=w364:i32)
                n183 = for {
                  tunnel: w359 -> [w384]
                  tunnel: [w383] -> w369 mode=indexing
                  tunnel: w364 -> [w380]
                  tunnel: w361 -> [w379] mode=indexing
                  i -> [w381]
                  n184 = Add(x=w381, y=w380) -> (x+y=w382:i32)
                  n185 = Build Array(w384, w379, w382) -> (w383:i32[])
                }
                n186 = case shown="0" w359 {
                  tunnel: w369 -> [w372 w377]
                  tunnel: [w372 w376] -> w368
                  tunnel: w363 -> [w371 w375]
                  tunnel: [w370 w373] -> w362
                  frame 0 {
                    n187 = Build Array(w371) -> (w370:string[])
                  }
                  frame 1, Default {
                    n188 = global read "Results_plotter_Global.vi" "Row Reference"() -> (w378:i32[][])
                    n189 = local read "Filetype"() -> (w374:string[])
                    n190 = Build Array (concatenate)(w374, w375) -> (w373:string[])
                    n191 = Build Array (concatenate)(w378, w377) -> (w376:i32[][])
                  }
                }
                "Filetype" <- w362
                n192 = Replace Array Subset(array=w360, new element=w358, index=w359) -> (w357:path[])
                n193 = global write "Results_plotter_Global.vi" "Row Reference"(w368) -> ()
              }
            }
            n194 = local write "Result files to read"(w344) -> ()
          }
        }
      }
      frame "Load Selectors" {
        n195 = while {
          shift-right: [w405] -> w390
          shift-left: _ -> [w407]
          tunnel: [w407] -> w389
          tunnel: w385 -> [w405]
          stop <- FALSE continue-if-true
        }
        n196 = Array Size(array=w397) -> (size(s)=w396:i32[])
        n197 = local read "Tolerances"() -> (w393:dbl[])
        n198 = Index Array(array=w396, index=0 ("Index")) -> (element=→"No Of Rows":i32)
        n199 = property on="X Ch Name" class="Ring (strict)"("Strings []"=w385) -> ()  [unwired: 2 in, 2 out]
        n200 = property on="Ordinate" class="Ring (strict)"("Strings []"=w385) -> ()  [unwired: 2 in, 2 out]
        n201 = property on="X Axis" class="Ring (strict)"("Strings []"=w385) -> ()  [unwired: 2 in, 2 out]
        n202 = property on="Y Ch Name" class="Ring (strict)"("Strings []"=w385) -> ()  [unwired: 2 in, 2 out]
        n203 = Equal?(x=w390, y=w389) -> (x = y?=w388:bool)
        n204 = Array Size(array=w385) -> (size(s)=w399:i32)
        n205 = Array Size(array=w393) -> (size(s)=w398:i32)
        n206 = property on="Multi Ordinate" class="LstBox (strict)"("Item Names"=w385) -> ()  [unwired: 2 in, 2 out]
        n207 = property on="Z Ch Name" class="Ring (strict)"("Strings []"=w385) -> ()  [unwired: 2 in, 2 out]
        n208 = Not Equal?(x=w399, y=w398) -> (x != y?=w400:bool)
        n209 = case shown="True" w400 {
          tunnel: w399 -> [_ w414]
          tunnel: w398 -> [_ w413]
          tunnel: w393 -> [_ w410]
          frame False {
          }
          frame True {
            n210 = Subtract(x=w414, y=w413) -> (x-y=w412:i32)
            n211 = Initialize Array(1.0 ("Element Data"), w412) -> (w409:dbl[])
            n212 = Build Array (concatenate)(w410, w409) -> (w408:dbl[])
            n213 = local write "Tolerances"(w408) -> ()
          }
        }
        n214 = Build Array (concatenate)("Don't Filter" ("Input Element"), w385) -> (w402:string[])
        n215 = global write "Results_plotter_Global.vi" "First Loop"(TRUE) -> ()
        n216 = property on="Filter on column 1:" class="Ring (strict)"("Strings []"=w402) -> ()  [unwired: 2 in, 2 out]
        n217 = Select(t="What is present?", s=w388, f="Set Axis Channels") -> (s? t:f=w392:string)
      }
      frame "Set Axis Channels" {
        n218 = Array Size(array=w421) -> (size(s)=w420:i32)
        n219 = Build Array("X" ("regular expression"), "Y" ("regular expression"), "Z" ("regular expression")) -> (w415:string[])
        n220 = Decrement(x=w420) -> (x-1=w419:i32)
        n221 = for {
          tunnel: w421 -> [w433]
          tunnel: w419 -> [w432]
          tunnel: w415 -> [w431] mode=indexing
          i -> [w427]
          n222 = while {
            tunnel: w433 -> [w447] mode=indexing
            tunnel: w432 -> [w446]
            tunnel: w431 -> [w444]
            tunnel: [w437] -> w430
            tunnel: [w442] -> w429
            i -> [w442]
            stop <- w445 continue-if-true
            n223 = call "Match_Pat_Case_In.vi"("String to match"=w444, "String"=w447) -> ("offset past match"=w441:i32)  [unwired: 1 in, 3 out]
            n224 = Less?(x=w442, y=w446) -> (x < y?=w443:bool)
            n225 = In Range and Coerce(upper limit=4, x=w441, lower limit=0) -> (In Range?=w438:bool)  [unwired: 1 out]
            n226 = Not(x=w438) -> (.not. x?=w437:bool)
            n227 = And(x=w437, y=w443) -> (x .and. y?=w445:bool)
          }
          n228 = Select(t=0, s=w430, f=w429) -> (s? t:f=w426:i32)
          n229 = case shown="1" w427 {
            tunnel: w426 -> [w434 w435 w436]
            frame 0, Default {
              n230 = local write "X Ch Name"(w434) -> ()
            }
            frame 1 {
              n231 = local write "Y Ch Name"(w435) -> ()
            }
            frame 2 {
              n232 = local write "Z Ch Name"(w436) -> ()
            }
          }
        }
      }
      frame "What is present?" {
        n233 = case shown="True" "Show Results Space Analysis" {
          tunnel: w451 -> [_ w455]
          tunnel: w450 -> [_ w454]
          frame False {
          }
          frame True {
            n234 = stacked-sequence {
              tunnel: w455 -> [w459]
              tunnel: w454 -> [w458]
              frame #0 {
                w456 = FALSE  # Summarise All
                n235 = call "Summarise.vi"("Channel Names"=w459, "Data"=w458, "Summarise All"=w456) -> ("Summary"=w457:string[][])  [unwired: 2 in]
                n236 = call "Results_Space_Analysis.vi"("Table"=w457) -> ()
              }
            }
          }
        }
      }
      frame "Ordinate Selector Type" {
        n237 = while {
          tunnel: [w478] -> w469
          shift-left: _ -> [w478]
          shift-right: ["Slice mode"] -> w470
          stop <- FALSE continue-if-true
          "Previous slice mode" <- w478
        }
        n238 = property on="Multi Ordinate" class="LstBox (strict)"("Visible"="Multi Ordinate?") -> ()  [unwired: 2 in, 2 out]
        n239 = global read "Results_plotter_Global.vi" "First Loop"() -> (w465:bool)
        n240 = Not(x="Multi Ordinate?") -> (.not. x?=w464:bool)
        n241 = local read "Intensity Plot?"() -> (w468:bool)
        n242 = property on="Ordinate Name" class="Str"("Visible"="Multi Ordinate?") -> ()  [unwired: 2 in, 2 out]
        n243 = property on="Ordinate" class="Ring (strict)"("Visible"=w464) -> ()  [unwired: 2 in, 2 out]
        n244 = Not Equal?(x=w470, y=w469) -> (x != y?=w461:bool)
        n245 = Or(x=w461, y="Update") -> (x .or. y?=w462:bool)
        n246 = case shown="False" "Multi Ordinate?" {
          frame False {
            n247 = Build Array("Ordinate") -> (w480:u16[])
            n248 = local write "Multi Ordinate"(w480) -> ()
          }
          frame True {
          }
        }
        n249 = Compound Arithmetic op=AND(invert w465, w462, w468) -> (w467:bool)
        "Slice mode Change?" <- w467
        n250 = property on="First Add label" class="Str"("Visible"=w464) -> ()  [unwired: 2 in, 2 out]
        n251 = property on="Additional Y Values" class="Arr (strict)"("Visible"=w464) -> ()  [unwired: 2 in, 2 out]
        n252 = property on="2nd Add label" class="Str"("Visible"=w464) -> ()  [unwired: 2 in, 2 out]
        n253 = Select(t="Change Slice mode", s=w467, f="Which rows are Non-Blank?") -> (s? t:f=w471:string)
        n254 = property on="Additional X Values" class="Arr (strict)"("Visible"=w464) -> ()  [unwired: 2 in, 2 out]
      }
      frame "Change Slice mode" {
        n255 = local read "Previous slice mode"() -> (w484:T4)
        n256 = local read "Slice mode"() -> (w498:T4)
        n257 = case shown="\"XY Slice (Plan)\"" w498 {
          tunnel: [w510 w515 w522 w527 w534 w540] -> w497
          tunnel: "Y Ch Name" -> [w508 w515 w522 w528 w533 w538]
          tunnel: "X Ch Name" -> [w510 w514 w521 w526 w534 w539]
          tunnel: [w509 w516 w521 w526 w533 w538] -> w488
          tunnel: "Z Ch Name" -> [w509 w516 w520 w527 w532 w540]
          tunnel: [w508 w514 w520 w528 w532 w539] -> w486
          tunnel: w484 -> [w507 w512 w518 w524 w531 w536]
          tunnel: [w505 w511 w517 w523 w530 w535] -> w483
          frame "XY Slice (Plan)" {
            n258 = Equal?(x=Plot_Slice."YX Slice (Plan)" ("Previous slice mode"), y=w507) -> (x = y?=w505:bool)
          }
          frame "YX Slice (Plan)" {
            n259 = Equal?(x=Plot_Slice."XY Slice (Plan)" ("Previous slice mode"), y=w512) -> (x = y?=w511:bool)
          }
          frame "YZ Slice (Cross)" {
            n260 = Equal?(x=Plot_Slice."ZY Slice (Cross)" ("Previous slice mode"), y=w518) -> (x = y?=w517:bool)
          }
          frame "ZY Slice (Cross)" {
            n261 = Equal?(x=Plot_Slice."YZ Slice (Cross)" ("Previous slice mode"), y=w524) -> (x = y?=w523:bool)
          }
          frame "XZ Slice (Side)" {
            n262 = Equal?(x=Plot_Slice."ZX Slice (Side)" ("Previous slice mode"), y=w531) -> (x = y?=w530:bool)
          }
          frame "ZX Slice (Side)" {
            n263 = Equal?(x=Plot_Slice."XZ Slice (Side)" ("Previous slice mode"), y=w536) -> (x = y?=w535:bool)
          }
        }
        n264 = case shown="True" w483 {
          frame False {
          }
          frame True {
            n265 = local read "Transpose"() -> (w504:bool)
            n266 = Not(x=w504) -> (.not. x?=w503:bool)
            n267 = local write "Transpose"(w503) -> ()
          }
        }
        n268 = local write "Update"(FALSE ("Update")) -> ()
        n269 = Increment(x=w488) -> (x+1=w491:u16)
        n270 = Increment(x=w486) -> (x+1=w490:u16)
        n271 = local read "Filter Array"() -> (w495:u16[])
        n272 = Array Subset(array=w495, index=2 ("Array Index")) -> (w493:u16[])  [unwired: 1 in]
        n273 = Build Array (concatenate)(w491, w490, w493) -> (w492:u16[])
        n274 = local write "Filter Array"(w492) -> ()
        n275 = local write "Absisca"(w497) -> ()
      }
      frame "Which rows are Non-Blank?" {
        n276 = while {
          tunnel: [w557] -> w551
          tunnel: [w558] -> w552
          shift-left: _ -> [w559]
          shift-right: [w560] -> w544
          shift-left: _ -> [w562]
          shift-right: [w561] -> _
          stop <- FALSE continue-if-true
          n277 = local read "Multi Ordinate"() -> (w560:i32[])
          n278 = local read "Absisca"() -> (w561:u16)
          n279 = Equal?(x=w561, y=w562) -> (x = y?=w558:bool)
          n280 = Equal?(x=w560, y=w559) -> (x = y?=w557:bool)
        }
        n281 = global read "Results_plotter_Global.vi" "First Loop"() -> (w546:bool)
        n282 = Compound Arithmetic op=AND(invert w546, w552, w551) -> (w550:bool)
        n283 = Array Size(array=w544) -> (size(s)=w543:i32)
        n284 = Greater?(x=w543, y=1) -> (0:w541:bool)
        n285 = global write "Results_plotter_Global.vi" "Multi Ordinate?"(w541) -> ()
        n286 = Select(t="Create Selectors", s=w550, f="Evaluate Blank Rows") -> (s? t:f=w547:string)
      }
      frame "Evaluate Blank Rows" {
        n287 = local read "Multi Ordinate"() -> (w564:i32[])
        n288 = local read "Absisca"() -> (w565:u16)
        n289 = for {
          tunnel: w566 -> [w572] mode=indexing
          tunnel: w565 -> [w575]
          tunnel: w564 -> [w574]
          tunnel: [w571] -> w563 mode=indexing
          n290 = Index Array(array=w572, index=w575) -> (element=w576:string)
          n291 = call "Convert_to_number.vi"("string"=w576) -> ("Number"=w577:dbl)  [unwired: 1 out]
          n292 = Not A Number/Path/Refnum?(number/path/refnum=w577) -> (NaN/Path/Refnum?=w573:bool)
          n293 = case shown="False" w573 {
            tunnel: w574 -> [w581 _]
            tunnel: w572 -> [w580 _]
            tunnel: [w578 FALSE] -> w571
            frame False {
              n294 = for {
                tunnel: w581 -> [w587] mode=indexing
                tunnel: w580 -> [w585]
                tunnel: [w582] -> w579 mode=indexing
                n295 = Index Array(array=w585, index=w587) -> (element=w586:string)
                n296 = call "Convert_to_number.vi"("string"=w586) -> ("Number"=w584:dbl)  [unwired: 1 out]
                n297 = Not A Number/Path/Refnum?(number/path/refnum=w584) -> (NaN/Path/Refnum?=w583:bool)
                n298 = Not(x=w583) -> (.not. x?=w582:bool)
              }
              n299 = Or Array Elements(Boolean array=w579) -> (logical OR=w578:bool)
            }
            frame True {
            }
          }
        }
        "Non-Blank Rows" <- w563
      }
      frame "Create Selectors" {
        n300 = local read "Non-Blank Rows"() -> (w592:bool[])
        n301 = local read "Tolerances"() -> (w590:dbl[])
        n302 = global read "Results_plotter_Global.vi" "Precision"() -> (w589:string[])
        n303 = Array Size(array=w600) -> (size(s)=w599:i32[])
        n304 = Index Array(array=w599, index=0 ("Index")) -> (element=w602:i32)
        n305 = for {
          tunnel: w600 -> [w618]
          tunnel: "Filter Array" -> [w610] mode=indexing
          shift-right: [w617] -> w591
          shift-left: _ -> [w615]
          tunnel: w602 -> [w616]
          tunnel: [w613] -> w597 mode=indexing
          tunnel: w592 -> [w612]
          tunnel: w590 -> [w611]
          tunnel: w589 -> [w608]
          i -> [w614]
          n306 = Decrement(x=w610) -> (x-1=w607:u16)
          n307 = Index Array(array=w608, index=w607) -> (element=w606:string)
          n308 = Index Array(array=w611, index=w607) -> (element=w609:dbl)
          n309 = case shown="5" w614 {
            tunnel: w618 -> [w631 w667 w708 w749 w790 w833 w874]
            tunnel: w610 -> [w630 w666 w707 w748 w789 w832 w873]
            tunnel: w609 -> [w629 w665 w706 w747 w788 w831 w872]
            tunnel: [w628 w664 w705 w746 w787 w830 w871] -> w617
            tunnel: w616 -> [w626 w663 w704 w745 w786 w829 w870]
            tunnel: w615 -> [_ w662 w703 w744 w785 w828 w869]
            tunnel: w614 -> [w625 w661 w700 w741 w782 w827 w866]
            tunnel: [w621 w656 w699 w740 w781 w822 w865] -> w613
            tunnel: w612 -> [w620 w655 w698 w739 w780 w821 w864]
            tunnel: w606 -> [w619 w654 w697 w738 w779 w820 w863]
            frame 0, Default {
              n310 = case shown="1, Default" w630 {
                tunnel: w631 -> [w637 w647]
                tunnel: w630 -> [w638 w646]
                tunnel: w629 -> [_ w653]
                tunnel: [w633 w650] -> w628
                tunnel: "Filter Bins 1" -> [_ w651]
                tunnel: [string[] [] ("Write Attribute") w652] -> w627
                tunnel: w626 -> [w635 _]
                tunnel: w625 -> [w641 w649]
                tunnel: [i32[] [0] ("Filter Bins Out") w648] -> w623
                tunnel: [TRUE ("Unchanged?") w645] -> w621
                tunnel: w620 -> [_ w644]
                tunnel: w619 -> [_ w643]
                frame 0 {
                  n311 = call "Create_filter_points.vi"("Channel to Filter On"=w638, "Index"=w641, "Ch Values In"=w637) -> ()  [unwired: 4 in, 4 out]
                  n312 = Initialize Array(TRUE, w635) -> (w634:bool[])
                  n313 = Build Array(w634) -> (w633:bool[][])
                }
                frame 1, Default {
                  n314 = call "Create_filter_points.vi"("Non-Blank Rows"=w644, "Precision"=w643, "Channel to Filter On"=w646, "Tolerance"=w653, "Index"=w649, "Filter Bins 1"=w651, "Ch Values In"=w647) -> ("Unchanged?"=w645:bool, "Accept array"=w650:bool[][], "Filter Bins Out"=w648:i32[], "Bin Names"=w652:string[])
                }
              }
              n315 = Equal?(x="Filter Bins 1", y=w623) -> (x = y?=w622:bool)
              n316 = case shown="False" w622 {
                tunnel: w623 -> [w632 _]
                frame False {
                  n317 = local write "Filter Bins 1"(w632) -> ()
                }
                frame True {
                }
              }
              n318 = property on="Filter bins 1" class="LstBox (strict)"("Item Names"=w627) -> ()  [unwired: 2 in, 2 out]
            }
            frame 1 {
              n319 = case shown="1, Default" w666 {
                tunnel: w667 -> [_ w679]
                tunnel: w666 -> [w670 w678]
                tunnel: w665 -> [_ w686]
                tunnel: [w674 w682] -> w664
                tunnel: "Filter Bins 2" -> [_ w684]
                tunnel: [string[] [] ("Write Attribute") w688] -> w660
                tunnel: w663 -> [_ _]
                tunnel: w662 -> [w674 w687]
                tunnel: w661 -> [w673 w685]
                tunnel: [i32[] [0] ("Filter Bins Out") w680] -> w659
                tunnel: [TRUE ("Unchanged?") w677] -> w656
                tunnel: w655 -> [_ w676]
                tunnel: w654 -> [_ w675]
                frame 0 {
                  n320 = call "Create_filter_points.vi"("Channel to Filter On"=w670, "Index"=w673) -> ()  [unwired: 5 in, 4 out]
                }
                frame 1, Default {
                  n321 = call "Create_filter_points.vi"("Non-Blank Rows"=w676, "Precision"=w675, "Channel to Filter On"=w678, "Tolerance"=w686, "Index"=w685, "Filter Bins 1"=w684, "Ch Values In"=w679) -> ("Unchanged?"=w677:bool, "Accept array"=w683:bool[][], "Filter Bins Out"=w680:i32[], "Bin Names"=w688:string[])
                  n322 = for {
                    tunnel: w687 -> [w693]
                    tunnel: w683 -> [w692] mode=indexing
                    shift-right: [w689] -> w682
                    shift-left: bool[][] [] -> [w691]
                    n323 = for {
                      tunnel: w692 -> [w696]
                      tunnel: w693 -> [w695] mode=indexing
                      tunnel: [w694] -> _ mode=indexing
                      tunnel: [w694] -> w690 mode=indexing
                      n324 = And(x=w696, y=w695) -> (x .and. y?=w694:bool[])
                    }
                    n325 = Build Array (concatenate)(w691, w690) -> (w689:bool[][])
                  }
                }
              }
              n326 = Equal?(x="Filter Bins 2", y=w659) -> (x = y?=w657:bool)
              n327 = case shown="False" w657 {
                tunnel: w659 -> [w668 _]
                frame False {
                  n328 = local write "Filter Bins 2"(w668) -> ()
                }
                frame True {
                }
              }
              n329 = property on="Filter Bins 2" class="LstBox (strict)"("Item Names"=w660) -> ()  [unwired: 2 in, 2 out]
            }
            frame 2 {
              n330 = case shown="0" w707 {
                tunnel: w708 -> [_ w718]
                tunnel: w707 -> [w711 w719]
                tunnel: w706 -> [_ w730]
                tunnel: [w714 w731] -> w705
                tunnel: "Filter 3" -> [_ w722]
                tunnel: [string[] [] ("Write Attribute") w733] -> w701
                tunnel: w704 -> [_ _]
                tunnel: w703 -> [w714 w732]
                tunnel: w700 -> [w713 w725]
                tunnel: [TRUE ("Unchanged?") w717] -> w699
                tunnel: w698 -> [_ w716]
                tunnel: w697 -> [_ w715]
                frame 0 {
                  n331 = call "Create_filter_points.vi"("Channel to Filter On"=w711, "Index"=w713) -> ()  [unwired: 5 in, 4 out]
                  n332 = local write "Filter 3"(0) -> ()
                }
                frame 1, Default {
                  n333 = Build Array(w722) -> (w729:u16[])
                  n334 = call "Create_filter_points.vi"("Non-Blank Rows"=w716, "Precision"=w715, "Channel to Filter On"=w719, "Tolerance"=w730, "Index"=w725, "Filter Bins 1"=w729, "Ch Values In"=w718) -> ("Unchanged?"=w717:bool, "Accept array"=w727:bool[][], "Filter Bins Out"=w723:i32[], "Bin Names"=w733:string[])
                  n335 = Index Array(array=w723, index=0 ("Index")) -> (element=w720:i32)
                  n336 = Index Array(array=w727, index (row)=0 ("Index")) -> (element=w726:bool[])  [unwired: 1 in]
                  n337 = Equal?(x=w722, y=w720) -> (x = y?=w721:bool)
                  n338 = case shown="True" w721 {
                    tunnel: w720 -> [w734 _]
                    frame False {
                      n339 = local write "Filter 3"(w734) -> ()
                    }
                    frame True {
                    }
                  }
                  n340 = for {
                    tunnel: w726 -> [w737]
                    tunnel: w732 -> [w736] mode=indexing
                    tunnel: [w735] -> w731 mode=indexing
                    n341 = And(x=w737, y=w736) -> (x .and. y?=w735:bool[])
                  }
                }
              }
              n342 = property on="Filter 3" class="Ring (strict)"("Strings []"=w701) -> ()  [unwired: 2 in, 2 out]
            }
            frame 3 {
              n343 = case shown="1, Default" w748 {
                tunnel: w749 -> [_ w760]
                tunnel: w748 -> [w752 w759]
                tunnel: w747 -> [_ w771]
                tunnel: [w755 w772] -> w746
                tunnel: "Filter 4" -> [_ w763]
                tunnel: [string[] [] ("Write Attribute") w774] -> w742
                tunnel: w745 -> [_ _]
                tunnel: w744 -> [w755 w773]
                tunnel: w741 -> [w754 w766]
                tunnel: [TRUE ("Unchanged?") w758] -> w740
                tunnel: w739 -> [_ w757]
                tunnel: w738 -> [_ w756]
                frame 0 {
                  n344 = call "Create_filter_points.vi"("Channel to Filter On"=w752, "Index"=w754) -> ()  [unwired: 5 in, 4 out]
                  n345 = local write "Filter 4"(0) -> ()
                }
                frame 1, Default {
                  n346 = Build Array(w763) -> (w770:u16[])
                  n347 = call "Create_filter_points.vi"("Non-Blank Rows"=w757, "Precision"=w756, "Channel to Filter On"=w759, "Tolerance"=w771, "Index"=w766, "Filter Bins 1"=w770, "Ch Values In"=w760) -> ("Unchanged?"=w758:bool, "Accept array"=w768:bool[][], "Filter Bins Out"=w764:i32[], "Bin Names"=w774:string[])
                  n348 = Index Array(array=w764, index=0 ("Index")) -> (element=w762:i32)
                  n349 = Equal?(x=w763, y=w762) -> (x = y?=w761:bool)
                  n350 = Index Array(array=w768, index (row)=0 ("Index")) -> (element=w767:bool[])  [unwired: 1 in]
                  n351 = case shown="False" w761 {
                    tunnel: w762 -> [w775 _]
                    frame False {
                      n352 = local write "Filter 4"(w775) -> ()
                    }
                    frame True {
                    }
                  }
                  n353 = for {
                    tunnel: w767 -> [w778]
                    tunnel: w773 -> [w777] mode=indexing
                    tunnel: [w776] -> w772 mode=indexing
                    n354 = And(x=w778, y=w777) -> (x .and. y?=w776:bool[])
                  }
                }
              }
              n355 = property on="Filter 4" class="Ring (strict)"("Strings []"=w742) -> ()  [unwired: 2 in, 2 out]
            }
            frame 4 {
              n356 = case shown="1, Default" w789 {
                tunnel: w790 -> [_ w801]
                tunnel: w789 -> [w793 w800]
                tunnel: w788 -> [_ w812]
                tunnel: [w796 w813] -> w787
                tunnel: "Filter 5" -> [_ w803]
                tunnel: [string[] [] ("Write Attribute") w815] -> w783
                tunnel: w786 -> [_ _]
                tunnel: w785 -> [w796 w814]
                tunnel: w782 -> [w795 w807]
                tunnel: [TRUE ("Unchanged?") w799] -> w781
                tunnel: w780 -> [_ w798]
                tunnel: w779 -> [_ w797]
                frame 0 {
                  n357 = call "Create_filter_points.vi"("Channel to Filter On"=w793, "Index"=w795) -> ()  [unwired: 5 in, 4 out]
                  n358 = local write "Filter 5"(0) -> ()
                }
                frame 1, Default {
                  n359 = Build Array(w803) -> (w811:u16[])
                  n360 = call "Create_filter_points.vi"("Non-Blank Rows"=w798, "Precision"=w797, "Channel to Filter On"=w800, "Tolerance"=w812, "Index"=w807, "Filter Bins 1"=w811, "Ch Values In"=w801) -> ("Unchanged?"=w799:bool, "Accept array"=w809:bool[][], "Filter Bins Out"=w805:i32[], "Bin Names"=w815:string[])
                  n361 = Index Array(array=w805, index=0 ("Index")) -> (element=w804:i32)
                  n362 = Equal?(x=w803, y=w804) -> (x = y?=w802:bool)
                  n363 = Index Array(array=w809, index (row)=0 ("Index")) -> (element=w808:bool[])  [unwired: 1 in]
                  n364 = case shown="False" w802 {
                    tunnel: w804 -> [w816 _]
                    frame False {
                      n365 = local write "Filter 5"(w816) -> ()
                    }
                    frame True {
                    }
                  }
                  n366 = for {
                    tunnel: w808 -> [w819]
                    tunnel: w814 -> [w818] mode=indexing
                    tunnel: [w817] -> w813 mode=indexing
                    n367 = And(x=w819, y=w818) -> (x .and. y?=w817:bool[])
                  }
                }
              }
              n368 = property on="Filter 5" class="Ring (strict)"("Strings []"=w783) -> ()  [unwired: 2 in, 2 out]
            }
            frame 5 {
              n369 = case shown="1, Default" w832 {
                tunnel: w833 -> [_ w850]
                tunnel: w832 -> [w836 w849]
                tunnel: w831 -> [_ w854]
                tunnel: [w840 w841] -> w830
                tunnel: "Single Series" -> [_ w852]
                tunnel: [string[] [] ("Write Attribute") w856] -> w826
                tunnel: w829 -> [_ _]
                tunnel: w828 -> [w840 w855]
                tunnel: w827 -> [w839 w853]
                tunnel: [i32[] [0] ("Filter Bins Out") w851] -> w825
                tunnel: [TRUE ("Unchanged?") w848] -> w822
                tunnel: w821 -> [_ w847]
                tunnel: w820 -> [_ w846]
                frame 0 {
                  n370 = call "Create_filter_points.vi"("Channel to Filter On"=w836, "Index"=w839) -> ()  [unwired: 5 in, 4 out]
                }
                frame 1, Default {
                  n371 = call "Create_filter_points.vi"("Non-Blank Rows"=w847, "Precision"=w846, "Channel to Filter On"=w849, "Tolerance"=w854, "Index"=w853, "Filter Bins 1"=w852, "Ch Values In"=w850) -> ("Unchanged?"=w848:bool, "Accept array"=w843:bool[][], "Filter Bins Out"=w851:i32[], "Bin Names"=w856:string[])
                  n372 = Index Array(array=w843, index (row)=0 ("Index")) -> (element=w844:bool[])  [unwired: 1 in]
                  n373 = for {
                    shift-right: [w857] -> w842
                    shift-left: w844 -> [w859]
                    tunnel: w843 -> [w858] mode=indexing
                    n374 = Or(x=w858, y=w859) -> (x .or. y?=w857:bool[])
                  }
                  n375 = for {
                    tunnel: w842 -> [w862]
                    tunnel: w855 -> [w861] mode=indexing
                    tunnel: [w860] -> w841 mode=indexing
                    n376 = And(x=w862, y=w861) -> (x .and. y?=w860:bool[])
                  }
                }
              }
              n377 = Equal?(x="Single Series", y=w825) -> (x = y?=w823:bool)
              n378 = case shown="False" w823 {
                tunnel: w825 -> [w834 _]
                frame False {
                  n379 = local write "Single Series"(w834) -> ()
                }
                frame True {
                }
              }
              n380 = property on="Single Series" class="LstBox (strict)"("Item Names"=w826) -> ()  [unwired: 2 in, 2 out]
            }
            frame 6 {
              n381 = case shown="1, Default" w873 {
                tunnel: w874 -> [_ w885]
                tunnel: w873 -> [w877 w884]
                tunnel: w872 -> [_ w892]
                tunnel: [w880 w897] -> w871
                tunnel: "Filter 6" -> [_ w887]
                tunnel: [string[] [] ("Write Attribute") w899] -> w867
                tunnel: w870 -> [_ _]
                tunnel: w869 -> [w880 w898]
                tunnel: w866 -> [w879 w891]
                tunnel: [TRUE ("Unchanged?") w883] -> w865
                tunnel: w864 -> [_ w882]
                tunnel: w863 -> [_ w881]
                frame 0 {
                  n382 = call "Create_filter_points.vi"("Channel to Filter On"=w877, "Index"=w879) -> ()  [unwired: 5 in, 4 out]
                  n383 = local write "Filter 6"(0) -> ()
                }
                frame 1, Default {
                  n384 = Build Array(w887) -> (w893:u16[])
                  n385 = call "Create_filter_points.vi"("Non-Blank Rows"=w882, "Precision"=w881, "Channel to Filter On"=w884, "Tolerance"=w892, "Index"=w891, "Filter Bins 1"=w893, "Ch Values In"=w885) -> ("Unchanged?"=w883:bool, "Accept array"=w895:bool[][], "Filter Bins Out"=w889:i32[], "Bin Names"=w899:string[])
                  n386 = Index Array(array=w889, index=0 ("Index")) -> (element=w888:i32)
                  n387 = Equal?(x=w887, y=w888) -> (x = y?=w886:bool)
                  n388 = Index Array(array=w895, index (row)=0 ("Index")) -> (element=w894:bool[])  [unwired: 1 in]
                  n389 = case shown="False" w886 {
                    tunnel: w888 -> [w900 _]
                    frame False {
                      n390 = local write "Filter 6"(w900) -> ()
                    }
                    frame True {
                    }
                  }
                  n391 = for {
                    tunnel: w894 -> [w903]
                    tunnel: w898 -> [w902] mode=indexing
                    tunnel: [w901] -> w897 mode=indexing
                    n392 = And(x=w903, y=w902) -> (x .and. y?=w901:bool[])
                  }
                }
              }
              n393 = property on="Filter 6" class="Ring (strict)"("Strings []"=w867) -> ()  [unwired: 2 in, 2 out]
            }
          }
        }
        "Accept Array" <- w591
        n394 = And Array Elements(Boolean array=w597) -> (logical AND=w596:bool)
        n395 = Select(t="Select all for Filter 2", s=w596, f="Create Selectors") -> (s? t:f=w594:string)
      }
      frame "Select all for Filter 2" {
        n396 = local read "Slice mode Change?"() -> (w905:bool)
        n397 = case shown="True" w905 {
          frame False {
          }
          frame True {
            n398 = property on="Filter Bins 2" class="LstBox (strict)"() -> ("Item Names"=w919:string[])  [unwired: 2 in, 2 out]
            n399 = Array Size(array=w919) -> (size(s)=w918:i32)
            n400 = Build Array("Blanks", "Numeric", "Non Numeric", "Non Blanks", "Show All" ("Input Element")) -> (w912:string[])
            n401 = local read "Filter Bins 1"() -> (w921:i32[])
            n402 = while {
              tunnel: w919 -> [w934] mode=indexing
              tunnel: w918 -> [w937]
              shift-right: [w928] -> w910
              shift-left: i32[] [] -> [w929]
              tunnel: w912 -> [w931]
              i -> [w930]
              stop <- w935 stop-if-true
              n403 = String Subset(string=w934, length (rest)=4 ("length (rest)")) -> (substring=w939:string)  [unwired: 1 out]
              n404 = Match Pattern(string=w934, regular expression=" (") -> (before substring=w932:string)  [unwired: 4 out]
              n405 = Search 1D Array(1D array=w931, element=w932) -> (index of element=w927:i32)  [unwired: 1 out]
              n406 = Equal?(x="NOT ", y=w939) -> (x = y?=w926:bool)
              n407 = Equal?(x=w937, y=w930) -> (x = y?=w936:bool)
              n408 = Less Than 0?(x=w927) -> (x < 0?=w925:bool)
              n409 = Or(x=w926, y=w936) -> (x .or. y?=w935:bool)
              n410 = Compound Arithmetic op=AND(w925, invert w926) -> (w924:bool)
              n411 = case shown="False" w924 {
                tunnel: w930 -> [_ w944]
                tunnel: w929 -> [w941 w943]
                tunnel: [w941 w942] -> w928
                frame False {
                }
                frame True {
                  n412 = Build Array (concatenate)(w943, w944) -> (w942:i32[])
                }
              }
            }
            n413 = Array Size(array=w921) -> (size(s)=w923:i32)
            n414 = case shown="1" w923 {
              tunnel: [w945 w948] -> w922
              tunnel: w921 -> [_ w947]
              tunnel: i32[] [1] ("Filter Bins 1") -> [w945 w946]
              frame 0, Default {
              }
              frame 1 {
                n415 = Index Array(array=w947, index=0 ("Index")) -> (element=w950:i32)
                n416 = Greater Than 0?(x=w950) -> (x > 0?=w949:bool)
                n417 = Select(t=w947, s=w949, f=w946) -> (s? t:f=w948:i32[])
              }
            }
            n418 = local write "Filter Bins 1"(w922) -> ()
            n419 = local write "Filter Bins 2"(w910) -> ()
          }
        }
      }
      frame "Re Plot Data?" {
        n420 = while {
          tunnel: [w998] -> w960
          shift-left: _ -> [w1000]
          shift-right: [w999] -> _
          tunnel: [w1003] -> w966
          shift-left: _ -> [w1001]
          shift-right: [w1002] -> _
          tunnel: [w1007] -> w968
          shift-left: _ -> [w1006]
          shift-right: [w1005] -> w952
          tunnel: [w1008] -> w969
          shift-left: _ -> [w1010]
          shift-right: [w1009] -> _
          tunnel: [w1012] -> w970
          shift-left: _ -> [w1011]
          shift-right: [w1004] -> _
          tunnel: [w1013] -> w973
          tunnel: [w1014] -> w974
          shift-left: _ -> [w1015]
          shift-right: [w1016] -> _
          shift-left: _ -> [w1018]
          shift-right: [w1017] -> _
          tunnel: [w1019] -> w953
          shift-left: _ -> [w1020]
          shift-right: [w1021] -> _
          tunnel: [w996] -> w963
          shift-right: [w993] -> _
          shift-left: _ -> [w992]
          tunnel: [w995] -> w962
          shift-right: [w991] -> _
          shift-left: _ -> [w994]
          tunnel: [w988] -> w961
          shift-right: [w989] -> _
          shift-left: _ -> [w990]
          shift-right: [w986] -> _
          shift-left: _ -> [w987]
          tunnel: [w985] -> w955
          stop <- FALSE continue-if-true
          n421 = local read "Ordinate Name"() -> (w986:string)
          n422 = local read "Additional X Values"() -> (w993:dbl[])
          n423 = local read "Additional Y Values"() -> (w991:dbl[])
          n424 = local read "Intensity Plot?"() -> (w1005:bool)
          n425 = local read "color and symbol"() -> (w989:bool)
          n426 = local read "Accept Array"() -> (w1021:bool[][])
          n427 = local read "No of Contours"() -> (w1002:i32)
          n428 = local read "Point Size"() -> (w999:i32)
          n429 = local read "Multi Ordinate"() -> (w1016:i32[])
          n430 = local read "Transpose"() -> (w1004:bool)
          n431 = local read "Resolution"() -> (w1009:dbl)
          n432 = local read "Absisca"() -> (w1017:u16)
          n433 = Equal?(x=w986, y=w987) -> (x = y?=w985:bool)
          n434 = Equal?(x=w1004, y=w1011) -> (x = y?=w1012:bool)
          n435 = Equal?(x=w989, y=w990) -> (x = y?=w988:bool)
          n436 = Equal?(x=w1002, y=w1001) -> (x = y?=w1003:bool)
          n437 = Equal?(x=w999, y=w1000) -> (x = y?=w998:bool)
          n438 = Equal?(x=w1009, y=w1010) -> (x = y?=w1008:bool)
          n439 = Equal?(x=w993, y=w992) -> (x = y?=w996:bool)
          n440 = Equal?(x=w991, y=w994) -> (x = y?=w995:bool)
          n441 = Equal?(x=w1017, y=w1018) -> (x = y?=w1014:bool)
          n442 = Equal?(x=w1021, y=w1020) -> (x = y?=w1019:bool)
          n443 = Equal?(x=w1005, y=w1006) -> (x = y?=w1007:bool)
          n444 = Equal?(x=w1016, y=w1015) -> (x = y?=w1013:bool)
        }
        n445 = global read "Results_plotter_Global.vi" "First Loop"() -> (w964:bool)
        n446 = while {
          shift-right: [w984] -> _
          shift-left: _ -> [w983]
          shift-right: [w981] -> _
          shift-left: _ -> [w982]
          tunnel: [w980] -> w959
          tunnel: [w979] -> w958
          stop <- FALSE continue-if-true
          n447 = local read "Filter Bins 1"() -> (w981:i32[])
          n448 = local read "Filter Bins 2"() -> (w984:i32[])
          n449 = Equal?(x=w981, y=w982) -> (x = y?=w979:bool)
          n450 = Equal?(x=w984, y=w983) -> (x = y?=w980:bool)
        }
        n451 = Not(x=w952) -> (.not. x?=w956:bool)
        n452 = property on="XY Plot" class="XYGraph (strict)"("Visible"=w956) -> ()  [unwired: 2 in, 2 out]
        n453 = property on="Intensity Graph" class="IntGraph (strict)"("Visible"=w952) -> ()  [unwired: 2 in, 2 out]
        n454 = property on="Resolution" class="DigNum (strict)"("Visible"=w952) -> ()  [unwired: 2 in, 2 out]
        n455 = property on="Bkgnd Value" class="DigNum (strict)"("Visible"=w952) -> ()  [unwired: 2 in, 2 out]
        n456 = Compound Arithmetic op=AND(w959, w958) -> (w957:bool)
        n457 = Compound Arithmetic op=AND(w955, w957, w960, w961, w966, w969, w970, w974, w973, w953, w968, w963, w962, invert w964) -> (w972:bool)
        n458 = Select(t="What to do next?", s=w972, f="Prepare for Plotting") -> (s? t:f=w971:string)
      }
      frame "Prepare for Plotting" {
        n459 = local read "Filter Array"() -> (w1030:u16[])
        n460 = local read "Multi Ordinate"() -> (w1024:i32[])
        n461 = Index Array(array=w1030, index=0 ("Index")) -> (element=w1027:u16)
        n462 = Equal To 0?(x=w1027) -> (x = 0?=w1028:bool)
        n463 = for {
          tunnel: w1024 -> [w1036] mode=indexing
          tunnel: [w1035] -> w1022 mode=indexing
          tunnel: w1023 -> [w1034]
          n464 = Index Array(array=w1034, index=w1036) -> (element=w1035:string)
        }
        "Ordinate Strings" <- w1022
        n465 = case shown="False" w1028 {
          tunnel: w1027 -> [w1042 _]
          tunnel: w1023 -> [w1040 _]
          tunnel: [w1037 string[] []] -> w1026
          frame False {
            n466 = Decrement(x=w1042) -> (x-1=w1041:u16)
            n467 = local read "Filter Bins 1"() -> (w1044:i32[])
            n468 = property on="Filter bins 1" class="LstBox (strict)"() -> ("Item Names"=w1043:string[])  [unwired: 2 in, 2 out]
            n469 = Index Array(array=w1040, index=w1041) -> (element=w1038:string)
            n470 = for {
              tunnel: w1044 -> [w1047] mode=indexing
              tunnel: w1043 -> [w1046]
              tunnel: [w1045] -> w1039 mode=indexing
              n471 = Index Array(array=w1046, index=w1047) -> (element=w1045:string)
            }
            n472 = Build Array (concatenate)(w1038, w1039) -> (w1037:string[])
          }
          frame True {
          }
        }
        "Filter 1 Strings" <- w1026
      }
      frame "Prepare Filter2 strings" {
        n473 = local read "Filter Array"() -> (w1055:u16[])
        n474 = Index Array(array=w1055, index=1 ("Index")) -> (element=w1052:u16)
        n475 = Equal To 0?(x=w1052) -> (x = 0?=w1053:bool)
        n476 = case shown="False" w1053 {
          tunnel: w1052 -> [w1064 _]
          tunnel: w1051 -> [w1062 _]
          tunnel: [w1059 string[] []] -> w1049
          frame False {
            n477 = Decrement(x=w1064) -> (x-1=w1063:u16)
            n478 = local read "Filter Bins 2"() -> (w1066:i32[])
            n479 = property on="Filter Bins 2" class="LstBox (strict)"() -> ("Item Names"=w1065:string[])  [unwired: 2 in, 2 out]
            n480 = Index Array(array=w1062, index=w1063) -> (element=w1060:string)
            n481 = for {
              tunnel: w1066 -> [w1069] mode=indexing
              tunnel: w1065 -> [w1068]
              tunnel: [w1067] -> w1061 mode=indexing
              n482 = Index Array(array=w1068, index=w1069) -> (element=w1067:string)
            }
            n483 = Build Array (concatenate)(w1060, w1061) -> (w1059:string[])
          }
          frame True {
          }
        }
        "Filter 2 Strings" <- w1049
      }
      frame "Plot Data" {
        n484 = stacked-sequence {
          seq-local: [w1077 _ _] -> [_ w1110 _]
          seq-local: [w1076 _ _] -> [_ w1109 _]
          tunnel: w1074 -> [_ w1119 _]
          tunnel: [_ TRUE _] -> w1073
          tunnel: [_ _ w1139] -> w1072
          tunnel: w1071 -> [w1078 _ _]
          frame #0 {
            n485 = local read "Ordinate Strings"() -> (w1077:string[])
            n486 = for {
              tunnel: w1077 -> [w1080] mode=indexing
              tunnel: w1078 -> [w1083]
              tunnel: [w1081] -> w1076 mode=indexing
              n487 = String Length(string=w1080) -> (length=w1079:i32)
              n488 = for {
                tunnel: w1080 -> [w1087]
                tunnel: w1083 -> [w1084] mode=indexing
                shift-right: [w1091] -> w1081
                shift-left: -1 -> [w1089]
                tunnel: w1079 -> [w1085]
                i -> [w1090]
                n489 = String Subset(string=w1084, length (rest)=w1085) -> (substring=w1086:string)  [unwired: 1 out]
                n490 = Equal?(x=w1086, y=w1087) -> (x = y?=w1088:bool)
                n491 = case shown="True" w1088 {
                  tunnel: [w1103 w1106] -> w1091
                  tunnel: w1090 -> [w1102 _]
                  tunnel: w1089 -> [w1101 w1106]
                  tunnel: w1085 -> [w1100 _]
                  tunnel: w1084 -> [w1099 _]
                  frame True {
                    n492 = String Subset(string=w1099, offset (0)=w1100) -> (substring=w1093:string)  [unwired: 1 out]
                    n493 = call <vilib>:"Trim Whitespace.vi"("string"=w1093) -> ("trimmed string"=w1092:string)  [unwired: 1 in]
                    n494 = Equal?(x=w1092, y="Err") -> (x = y?=w1095:bool)
                    n495 = Equal?(x=w1092, y="err") -> (x = y?=w1096:bool)
                    n496 = Or(x=w1095, y=w1096) -> (x .or. y?=w1094:bool)
                    n497 = case shown="True" w1094 {
                      tunnel: [w1104 w1105] -> w1103
                      tunnel: w1102 -> [w1104 _]
                      tunnel: w1101 -> [_ w1105]
                      frame True {
                      }
                      frame False {
                      }
                    }
                  }
                  frame False {
                  }
                }
              }
            }
          }
          frame #1 {
            n498 = local read "Accept Array"() -> (w1121:bool[][])
            n499 = local read "Filter 1 Strings"() -> (w1123:string[])
            n500 = local read "Filter 2 Strings"() -> (w1122:string[])
            n501 = local read "Multi Ordinate?"() -> (w1115:bool)
            n502 = Select(t=5, s=w1115, f=2 ("y")) -> (s? t:f=w1113:i32)
            n503 = global write "Results_plotter_Global.vi" "Ordinate"("Multi Ordinate") -> ()
            n504 = global write "Results_plotter_Global.vi" "Absisca"("Absisca") -> ()
            n505 = global write "Results_plotter_Global.vi" "Transpose"("Transpose") -> ()
            n506 = while {
              shift-right: [w1126] -> w1118
              shift-left: _ -> [w1127]
              tunnel: "color and symbol" -> [w1128]
              tunnel: w1113 -> [w1124]
              stop <- FALSE continue-if-true
              n507 = case shown="True" w1128 {
                tunnel: w1127 -> [w1135 w1137]
                tunnel: [w1134 w1137] -> w1126
                tunnel: w1124 -> [w1129 _]
                frame True {
                  n508 = Add(x=w1135, y=1) -> (x+y=w1132:i32)
                  n509 = local write "color and symbol"(FALSE ("color and symbol")) -> ()
                  n510 = Greater?(x=w1132, y=w1129) -> (0:w1133:bool)
                  n511 = Select(t=0, s=w1133, f=w1132) -> (s? t:f=w1134:i32)
                }
                frame False {
                }
              }
            }
            n512 = call "Plot_XY_data.vi"("Channel Values"=w1119, "Ordinate Strings"=w1110, "Swap color and symbol"=w1118, "Error Bar Chs"=w1109, "Accept Array"=w1121, "Filter 1 Strings"=w1123, "Filter 2 Strings"=w1122, "Ordinate"="Multi Ordinate", "Absisca"="Absisca", "Transpose"="Transpose") -> ("Accept Array Out"=→"Plotted Series":bool[][])  [unwired: 5 out]
          }
          frame #2 {
            n513 = Select(t="Intensity plot", s="Intensity Plot?", f="Add Legend and scales") -> (s? t:f=w1139:string)
            n514 = property on="Surface Area" class="DigNum (strict)"("Visible"="Intensity Plot?") -> ()  [unwired: 2 in, 2 out]
            n515 = property on="Surface Integral" class="DigNum (strict)"("Visible"="Intensity Plot?") -> ()  [unwired: 2 in, 2 out]
            n516 = property on="Surface Average" class="DigNum (strict)"("Visible"="Intensity Plot?") -> ()  [unwired: 2 in, 2 out]
            n517 = property on="X Ch Name" class="Ring (strict)"("Visible"="Intensity Plot?") -> ()  [unwired: 2 in, 2 out]
            n518 = property on="Y Ch Name" class="Ring (strict)"("Visible"="Intensity Plot?") -> ()  [unwired: 2 in, 2 out]
            n519 = property on="Z Ch Name" class="Ring (strict)"("Visible"="Intensity Plot?") -> ()  [unwired: 2 in, 2 out]
            n520 = property on="Point Size" class="Slide (strict)"("Visible"="Intensity Plot?") -> ()  [unwired: 2 in, 2 out]
            n521 = property on="No of Contours" class="DigNum (strict)"("Visible"="Intensity Plot?") -> ()  [unwired: 2 in, 2 out]
            n522 = property on="Slice mode" class="Enum (strict)"("Visible"="Intensity Plot?") -> ()  [unwired: 2 in, 2 out]
            n523 = property on="Plot Resolution" class="Bool (strict)"("Visible"="Intensity Plot?") -> ()  [unwired: 2 in, 2 out]
            n524 = property on="Update" class="Bool (strict)"("Visible"="Intensity Plot?") -> ()  [unwired: 2 in, 2 out]
          }
        }
      }
      frame "Add Legend and scales" {
        n525 = local read "Transpose"() -> (w1145:bool)
        n526 = global read "Results_plotter_Global.vi" "Plot Index values"() -> (w1148:dbl[][])
        n527 = global read "Results_plotter_Global.vi" "XY Graph Cluster"() -> (→"XY Plot":cluster{dbl[], dbl[]}[])
        n528 = Select(t=1 ("index (row)"), s=w1145, f=0 ("index (row)")) -> (s? t:f=w1142:i32)
        n529 = Index Array(array=w1148, index (row)=w1142) -> (element=w1147:dbl[])  [unwired: 1 in]
        n530 = Array Max & Min(array=w1147) -> (max value=w1146:dbl)  [unwired: 3 out]
        n531 = global read "Results_plotter_Global.vi" "Point info"() -> (w1153:T12)
        n532 = global read "Results_plotter_Global.vi" "Legend"() -> (w1154:string[])
        n533 = Greater?(x=w1146, y=2680560000.0) -> (0:w1150:bool)
        n534 = case shown="False" w1150 {
          tunnel: [w1165 u8 7 ("X Scale.Format & Precision:Precision")] -> w1149
          tunnel: w1146 -> [w1171 _]
          frame False {
            n535 = Absolute Value(x=w1171) -> (abs(x)=w1164:dbl)
            n536 = In Range and Coerce(upper limit=100000.0 ("y"), x=w1164, lower limit=0.0001) -> (In Range?=w1168:bool)  [unwired: 1 out]
            n537 = Select(t=u8 0 ("f"), s=w1168, f=u8 1) -> (s? t:f=w1165:u8)
          }
          frame True {
          }
        }
        n538 = local write "Warning!"("") -> ()
        n539 = for {
          tunnel: w1154 -> [w1188] mode=indexing
          tunnel: w1153 -> [w1185] mode=indexing
          tunnel: [w1186] -> w1158
          i -> [w1186]
          n540 = call "Abbreviate_string.vi"("Input String"=w1188, "Max String Length"=50) -> ("Output String"=w1179:string)
          n541 = Unbundle By Name(w1185) -> ("Point Style"=w1184:u8, "Fill/Pt. Color"=w1183:u32)
          n542 = String Length(string=w1179) -> (length=w1182:i32)
          n543 = Subtract(x=w1182, y=2) -> (x-y=w1180:i32)
          n544 = String Subset(string=w1179, length (rest)=w1180) -> (substring=w1178:string)  [unwired: 1 out]
          n545 = property on="XY Plot" class="XYGraph (strict)"("Active Plot"=w1186, "Plot.Plot Name"=w1178, "Plot.Point Style"=w1184, "Plot.Fill/Point Color"=w1183, "Plot.Plot Color"=w1183) -> ()  [unwired: 2 in, 2 out]
        }
        n546 = Increment(x=w1158) -> (x+1=w1157:i32)
        n547 = property on="XY Plot" class="XYGraph (strict)"("X Scale.Format & Precision:Format"=w1149) -> ()  [unwired: 2 in, 2 out]
        n548 = for {
          N: 10 -> [_]
          tunnel: w1157 -> [w1176]
          i -> [w1177]
          w1173 = u32 0
          n549 = Add(x=w1176, y=w1177) -> (x+y=w1175:i32)
          n550 = property on="XY Plot" class="XYGraph (strict)"("Active Plot"=w1175, "Plot.Plot Name"="" ("Write Attribute"), "Plot.Plot Color"=w1173, "Plot.Fill/Point Color"=w1173) -> ()  [unwired: 2 in, 2 out]
        }
      }
      frame "Add Axis names" {
        n551 = local read "Multi Ordinate"() -> (w1203:i32[])
        n552 = for {
          tunnel: w1203 -> [w1220] mode=indexing
          shift-right: [w1217] -> w1196
          shift-left: "" -> [w1216]
          tunnel: w1204 -> [w1219]
          tunnel: [w1212] -> w1195
          i -> [w1212]
          n553 = Index Array(array=w1219, index=w1220) -> (element=w1218:string)
          n554 = String Length(string=w1216) -> (length=w1215:i32)
          n555 = Less?(x=w1215, y=30) -> (x < y?=w1213:bool)
          n556 = case shown="True" w1213 {
            tunnel: w1218 -> [_ w1225]
            tunnel: [w1221 w1224] -> w1217
            tunnel: w1216 -> [w1221 w1222]
            frame False {
            }
            frame True {
              n557 = Concatenate Strings(w1222, w1225, "   ") -> (w1224:string)
            }
          }
        }
        n558 = Greater Than 0?(x=w1195) -> (x > 0?=w1193:bool)
        n559 = local read "Transpose"() -> (w1206:bool)
        n560 = local read "Absisca"() -> (w1207:u16)
        n561 = Index Array(array=w1204, index=w1207) -> (element=w1205:string)
        n562 = String Length(string=w1196) -> (length=w1199:i32)
        n563 = Empty String/Path?(string/path="Ordinate Name") -> (empty?=w1194:bool)
        n564 = Subtract(x=w1199, y=3) -> (x-y=w1197:i32)
        n565 = Compound Arithmetic op=AND(invert w1194, w1193) -> (w1192:bool)
        n566 = String Subset(string=w1196, length (rest)=w1197) -> (substring=w1191:string)  [unwired: 1 out]
        n567 = Select(t="Ordinate Name", s=w1192, f=w1191) -> (s? t:f=w1189:string)
        n568 = case shown="False" w1206 {
          tunnel: [w1226 w1229] -> w1202
          tunnel: w1189 -> [w1227 w1229]
          tunnel: [w1227 w1228] -> w1201
          tunnel: w1205 -> [w1226 w1228]
          frame False {
          }
          frame True {
          }
        }
        n569 = global write "Results_plotter_Global.vi" "X Axis Name"(w1202) -> ()
        n570 = global write "Results_plotter_Global.vi" "Y Axis Name"(w1201) -> ()
        n571 = global write "Results_plotter_Global.vi" "Value plotted Name"(w1189) -> ()
        n572 = property on="XY Plot" class="XYGraph (strict)"("X Scale.Name Label.Text"=w1202, "Y Scale.Name Label.Text"=w1201) -> ()  [unwired: 2 in, 2 out]
      }
      frame "Intensity plot" {
        # "Max"
        # "Min"
        n573 = global read "Results_plotter_Global.vi" "XY Graph Cluster"() -> (w1230:cluster{dbl[], dbl[]}[])
        n574 = local read "Tolerances"() -> (w1235:dbl[])
        n575 = local read "Absisca"() -> (w1234:u16)
        n576 = local read "Transpose"() -> (w1231:bool)
        n577 = stacked-sequence {
          seq-local: [w1248 _ _ _ _ _ _ _ _ _ _ _ _] -> [_ _ _ w1313 w1320 _ w1345 _ _ _ _ _ _]
          seq-local: [_ w1264 _ _ _ _ _ _ _ _ _ _ _] -> [_ _ _ _ w1319 _ w1344 _ _ _ _ _ _]
          seq-local: [_ _ w1296 _ _ _ _ _ _ _ _ _ _] -> [_ _ _ _ _ _ w1353 _ _ _ _ _ _]
          seq-local: [_ _ _ _ _ _ w1355 _ _ _ _ _ _] -> [_ _ _ _ _ _ _ _ w1379 _ _ _ _]
          seq-local: [_ _ _ _ _ _ w1354 _ _ _ _ _ _] -> [_ _ _ _ _ _ _ _ w1380 _ _ _ _]
          seq-local: [_ w1260 _ _ _ _ _ _ _ _ _ _ _] -> [_ _ _ _ _ _ _ _ _ w1444 _ _ _]
          seq-local: [_ _ _ w1311 _ _ _ _ _ _ _ _ _] -> [_ _ _ _ w1318 _ w1349 _ _ _ _ _ _]
          seq-local: [_ _ _ _ _ _ _ _ _ _ _ w1470 _] -> [_ _ _ _ _ _ _ _ _ _ _ _ w1520]
          seq-local: [_ _ _ _ _ _ _ _ _ _ _ w1469 _] -> [_ _ _ _ _ _ _ _ _ _ _ _ w1521]
          seq-local: [_ _ _ w1310 _ _ _ _ _ _ _ _ _] -> [_ _ _ _ _ w1333 _ _ _ _ _ _ _]
          seq-local: [_ _ _ _ _ _ _ _ _ _ _ w1467 _] -> [_ _ _ _ _ _ _ _ _ _ _ _ w1513]
          tunnel: [_ _ _ TRUE _ _ _ _ _ _ _ _ _] -> w1241
          tunnel: [_ _ _ _ _ _ _ _ _ _ _ _ "Analyse Plot Space"] -> w1240
          tunnel: w1238 -> [w1245 _ _ _ _ _ _ _ _ _ _ _ _]
          tunnel: w1239 -> [w1246 _ w1297 _ _ _ _ _ _ w1425 _ _ _]
          tunnel: [w1246 _ _ _ _ _ _ _ _ _ _ _ _] -> w1237
          tunnel: [w1245 _ _ _ _ _ _ _ _ _ _ _ _] -> w1236
          tunnel: w1235 -> [w1250 _ _ _ _ _ _ _ _ _ _ _ _]
          tunnel: w1230 -> [w1249 _ _ w1315 _ _ _ _ _ _ _ _ _]
          tunnel: w1234 -> [w1247 _ _ _ _ _ _ _ _ w1441 _ _ _]
          tunnel: w1231 -> [w1244 _ _ w1312 _ _ w1357 _ _ w1439 _ _ _]
          tunnel: [_ w1265 _ _ _ _ _ _ _ _ _ _ _] -> w1233
          tunnel: w1232 -> [_ w1265 _ _ _ _ _ _ _ w1426 _ _ _]
          frame #0 {
            n578 = Not(x=w1244) -> (.not. x?=w1243:bool)
            n579 = for {
              tunnel: w1249 -> [w1259] mode=indexing
              tunnel: w1243 -> [w1256]
              shift-right: [w1254] -> w1251
              shift-left: dbl[] [] -> [w1255]
              n580 = Unbundle(w1259) -> (w1258:dbl[], w1257:dbl[])
              n581 = Select(t=w1258, s=w1256, f=w1257) -> (s? t:f=w1253:dbl[])
              n582 = Build Array (concatenate)(w1255, w1253) -> (w1254:dbl[])
            }
            n583 = Index Array(array=w1250, index=w1247) -> (element=w1242:dbl)
            n584 = call "Numeric_bins.vi"("Values"=w1251, "Tolerance"=w1242) -> ("Bin Centres"=w1248:dbl[])  [unwired: 2 out]
          }
          frame #1 {
            n585 = local read "Filter Bins 2"() -> (w1266:i32[])
            n586 = local read "Filter Bins 1"() -> (w1268:i32[])
            n587 = Array Size(array=w1266) -> (size(s)=w1270:i32)
            n588 = Array Size(array=w1268) -> (size(s)=w1271:i32)
            n589 = Greater?(x=w1271, y=w1270) -> (0:w1269:bool)
            n590 = case shown="True" w1269 {
              tunnel: w1268 -> [_ w1293]
              tunnel: [w1289 w1293] -> w1267
              tunnel: [w1290 w1292] -> w1262
              tunnel: w1266 -> [w1289 _]
              tunnel: [1 0] -> w1260
              frame False {
                n591 = property on="Filter Bins 2" class="LstBox (strict)"() -> ("Item Names"=w1290:string[])  [unwired: 2 in, 2 out]
              }
              frame True {
                n592 = property on="Filter Bins 1" class="LstBox (strict)"() -> ("Item Names"=w1292:string[])  [unwired: 2 in, 2 out]
              }
            }
            n593 = Array Size(array=w1262) -> (size(s)=w1261:i32)
            n594 = for {
              tunnel: w1267 -> [w1276] mode=indexing
              tunnel: w1262 -> [w1282]
              shift-right: [w1279] -> w1264
              shift-left: dbl[] [] -> [w1280]
              tunnel: w1261 -> [w1275]
              n595 = Index Array(array=w1282, index=w1276) -> (element=w1278:string)
              n596 = Less?(x=w1276, y=w1275) -> (x < y?=w1274:bool)
              n597 = Match Pattern(string=w1278, regular expression=" (0)") -> (offset past match=w1277:i32)  [unwired: 4 out]
              n598 = Less Than 0?(x=w1277) -> (x < 0?=w1273:bool)
              n599 = And(x=w1273, y=w1274) -> (x .and. y?=w1272:bool)
              n600 = case shown="True" w1272 {
                tunnel: w1280 -> [w1283 w1287]
                tunnel: [w1283 w1286] -> w1279
                tunnel: w1278 -> [_ w1285]
                frame False {
                }
                frame True {
                  n601 = Fract/Exp String To Number(string=w1285) -> (number=w1284:dbl)  [unwired: 4 out]
                  n602 = Build Array (concatenate)(w1287, w1284) -> (w1286:dbl[])
                }
              }
            }
          }
          frame #2 {
            n603 = local read "Template"() -> (w1295:path)
            n604 = call "Valid_Path.vi"("Filename"=w1295) -> ("Valid Path?"=w1294:bool)
            n605 = case shown="True" w1294 {
              tunnel: w1295 -> [_ w1307]
              tunnel: w1297 -> [_ w1306]
              tunnel: [nan w1303] -> w1296
              frame False {
              }
              frame True {
                n606 = local read "Multi Ordinate"() -> (w1302:i32[])
                n607 = call "Read_Write_Template.vi"("Template File"=w1307, "Mode"=Global_mode."Read Global", "Channel names In"=w1306, "Data type"="Minimum Value") -> ("1D Info Out"=w1305:string[])  [unwired: 4 in, 7 out]
                n608 = Index Array(array=w1302, index=0 ("Index")) -> (element=w1301:i32)
                n609 = Index Array(array=w1305, index=w1301) -> (element=w1304:string)
                n610 = Fract/Exp String To Number(string=w1304, default (0 dbl)=nan) -> (number=w1303:dbl)  [unwired: 3 out]
              }
            }
          }
          frame #3 {
            n611 = call "Grid_Data.vi"("Transpose"=w1312, "XY Graph"=w1315, "Bin Centres"=w1313) -> ("No of Duplicates"=w1310:i32, "Grided data"=w1311:dbl[][])
          }
          frame #4 {
            n612 = for {
              tunnel: w1320 -> [w1325]
              tunnel: w1319 -> [w1324] mode=indexing
              tunnel: w1318 -> [w1323] mode=indexing
              shift-right: [w1321] -> w1316
              shift-left: dbl[][] [] -> [w1322]
              n613 = for {
                tunnel: w1325 -> [w1331] mode=indexing
                tunnel: w1324 -> [w1326]
                tunnel: w1323 -> [w1330] mode=indexing
                shift-right: [w1327] -> w1321
                shift-left: w1322 -> [w1329]
                n614 = Build Array(w1331, w1326, w1330) -> (w1328:dbl[])
                n615 = Build Array (concatenate)(w1329, w1328) -> (w1327:dbl[][])
              }
            }
            n616 = global write "Results_plotter_Global.vi" "Intensity Plot data in rows"(w1316) -> ()
          }
          frame #5 {
            n617 = case shown="1, Default" w1333 {
              tunnel: w1333 -> [_ w1337]
              tunnel: ["" w1335] -> w1332
              frame 0 {
              }
              frame 1, Default {
                n618 = Format Into String(format string="The Intensity Plot has %d duplicate points which have been averged together.", w1337) -> (resulting string=w1335:string)  [unwired: 2 in, 1 out]
              }
            }
            "Warning!" <- w1332
          }
          frame #6 {
            n619 = call "Insert_extra_rows_and_col.vi"("Row Values In"=w1344, "Additional Row Values"="Additional X Values", "Column Values In"=w1345, "Data In"=w1349, "Additional Column Values"="Additional Y Values") -> ("Row Values Out"=w1346:dbl[], "Column Values Out"=w1347:dbl[], "Data Out"=w1348:dbl[][])  [unwired: 2 out]
            n620 = Select(t="Resolution", s="Plot Resolution", f=0.0) -> (s? t:f=w1339:dbl)
            n621 = call "2D_interpolation.vi"("X Axis Current"=w1347, "Min Z Value In"=w1353, "Y axis Current"=w1346, "Bkgnd Value"="Bkgnd Value", "Plot In"=w1348, "Increment Value"=w1339, "Transpose"=w1357, "Point Size"="Point Size") -> ("min Z value"=w1355:dbl, "max Z value"=w1354:dbl, "Increment Value Out"=w1343:dbl, "Plot Out"=→"Intensity Graph":dbl[][])  [unwired: 4 out]
            n622 = local write "Resolution"(w1343) -> ()
          }
          frame #7 {
            n623 = global read "Results_plotter_Global.vi" "X Scale"() -> (w1365:cluster{"Xo":dbl, "delta X":dbl})
            n624 = global read "Results_plotter_Global.vi" "Y Scale"() -> (w1361:cluster{"Xo":dbl, "delta X":dbl})
            n625 = global read "Results_plotter_Global.vi" "Y Max"() -> (w1362:dbl)
            n626 = global read "Results_plotter_Global.vi" "X Max"() -> (w1363:dbl)
            n627 = Unbundle By Name(w1361) -> ("Xo"=w1360:dbl)
            n628 = Unbundle By Name(w1365) -> ("Xo"=w1364:dbl)
            n629 = Subtract(x=w1362, y=w1360) -> (x-y=w1366:dbl)
            n630 = Subtract(x=w1363, y=w1364) -> (x-y=w1375:dbl)
            n631 = Greater?(x=w1375, y=5.0) -> (0:w1373:bool)
            n632 = Greater?(x=w1366, y=5.0) -> (0:w1368:bool)
            n633 = Select(t=u8 0 ("Write Attribute"), s=w1373, f=u8 3) -> (s? t:f=w1359:u8)
            n634 = Select(t=u8 0 ("Write Attribute"), s=w1368, f=u8 3) -> (s? t:f=w1358:u8)
            n635 = property on="Intensity Graph" class="IntGraph (strict)"("X Scale.Offset and Multiplier"=w1365, "X Scale.Range:Maximum"=w1363, "Y Scale.Offset and Multiplier"=w1361, "Y Scale.Range:Maximum"=w1362, "X Scale.Format & Precision:Precision"=w1359, "Y Scale.Format & Precision:Precision"=w1358) -> ()  [unwired: 2 in, 2 out]
          }
          frame #8 {
            n636 = Greater Than 0?(x=w1380) -> (x > 0?=w1377:bool)
            n637 = Less Than 0?(x=w1379) -> (x < 0?=w1378:bool)
            n638 = And(x=w1377, y=w1378) -> (x .and. y?=w1376:bool)
            n639 = case shown="True" w1376 {
              tunnel: w1380 -> [w1409 w1423]
              tunnel: [w1417 w1421] -> w1382
              tunnel: w1379 -> [w1405 w1418]
              frame True {
                (unwired) u32 3743
                (unwired) u32 16721152
                n640 = Absolute Value(x=w1405) -> (abs(x)=w1404:dbl)
                n641 = Absolute Value(x=w1409) -> (abs(x)=w1411:dbl)
                n642 = Absolute Value(x=w1405) -> (abs(x)=w1412:dbl)
                n643 = Max & Min(x=w1411, y=w1412) -> (max(x,y)=w1407:dbl)  [unwired: 1 out]
                n644 = Divide(x=w1404, y=w1407) -> (x/y=w1398:dbl)
                n645 = Subtract(x=1.0, y=w1398) -> (x-y=w1397:dbl)
                n646 = Multiply(x=w1397, y=u32 255) -> (x*y=w1403:dbl)
                n647 = To Unsigned Long Integer(number=w1403) -> (unsigned 32bit integer=w1387:u32)
                n648 = Multiply(x=w1387, y=u32 256) -> (x*y=w1389:u32)
                n649 = Multiply(x=w1387, y=u32 65536) -> (x*y=w1386:u32)
                n650 = Compound Arithmetic op=ADD(w1386, w1389, u32 255) -> (w1385:u32)
                n651 = Bundle("min Z value"=w1405, w1385) -> (w1414:cluster{"min Z value":dbl, u32})  [unwired: 1 out]
                n652 = Divide(x=w1409, y=w1407) -> (x/y=w1402:dbl)
                n653 = Bundle("max Z value"=0.0, u32 16777215) -> (w1413:cluster{"max Z value":dbl, u32})  [unwired: 1 out]
                n654 = Subtract(x=1.0, y=w1402) -> (x-y=w1400:dbl)
                n655 = Multiply(x=w1400, y=u32 255) -> (x*y=w1396:dbl)
                n656 = To Unsigned Long Integer(number=w1396) -> (unsigned 32bit integer=w1383:u32)
                n657 = Multiply(x=w1383, y=u32 256) -> (x*y=w1393:u32)
                n658 = Compound Arithmetic op=ADD(w1383, w1393, u32 16711680) -> (w1384:u32)
                n659 = Bundle("max Z value"=w1409, w1384) -> (w1416:cluster{"max Z value":dbl, u32})  [unwired: 1 out]
                n660 = Build Array(w1416, w1414) -> (w1415:cluster{"min Z value":dbl, u32}[])
                n661 = Build Array (concatenate)(w1415, w1413) -> (w1417:cluster{"max Z value":dbl, u32}[])
              }
              frame False {
                n662 = Bundle("max Z value"=w1423, u32 16721152) -> (w1420:cluster{"max Z value":dbl, u32})  [unwired: 1 out]
                n663 = Bundle("min Z value"=w1418, u32 3743) -> (w1419:cluster{"min Z value":dbl, u32})  [unwired: 1 out]
                n664 = Build Array(w1420, w1419) -> (w1421:cluster{"min Z value":dbl, u32}[])
              }
            }
            n665 = property on="Intensity Graph" class="IntGraph (strict)"("Ignore Array"=FALSE ("Write Attribute"), "Z Scale.Marker Values[]"=w1382) -> ()  [unwired: 2 in, 2 out]
          }
          frame #9 {
            n666 = local read "Filter Array"() -> (w1443:u16[])
            n667 = Index Array(array=w1443, index=w1444) -> (element=w1442:u16)
            n668 = Decrement(x=w1442) -> (x-1=w1440:u16)
            n669 = local read "Multi Ordinate"() -> (w1430:i32[])
            n670 = Index Array(array=w1426, index=w1440) -> (element=w1434:string)
            n671 = Index Array(array=w1426, index=w1441) -> (element=w1433:string)
            n672 = case shown="False" w1439 {
              tunnel: [w1446 w1448] -> w1432
              tunnel: w1434 -> [w1446 w1447]
              tunnel: w1433 -> [w1445 w1448]
              tunnel: [w1445 w1447] -> w1431
              frame False {
              }
              frame True {
              }
            }
            n673 = Index Array(array=w1430, index=0) -> (element=w1428:i32)
            n674 = Index Array(array=w1425, index=w1428) -> (element=w1427:string)
            n675 = global write "Results_plotter_Global.vi" "Value plotted Name"(w1427) -> ()
            n676 = property on="Intensity Graph" class="IntGraph (strict)"("X Scale.Name Label.Text"=w1431, "Y Scale.Name Label.Text"=w1432) -> ()  [unwired: 2 in, 2 out]
            n677 = global write "Results_plotter_Global.vi" "Y Axis Name"(w1431) -> ()
            n678 = global write "Results_plotter_Global.vi" "X Axis Name"(w1432) -> ()
            n679 = Format Into String(format string="Add %s values", w1434) -> (resulting string=→"First Add label":string)  [unwired: 2 in, 1 out]
            n680 = Format Into String(format string="Add %s values", w1433) -> (resulting string=→"2nd Add label":string)  [unwired: 2 in, 1 out]
          }
          frame #10 {
            n681 = property on="Intensity Graph" class="IntGraph (strict)"() -> ("Color Table"=w1450:u32[])  [unwired: 2 in, 2 out]
            n682 = Increment(x="No of Contours") -> (x+1=w1451:i32)
            n683 = Divide(x=255, y=w1451) -> (x/y=w1455:dbl)
            n684 = To Long Integer(number=w1455) -> (32bit integer=w1454:i32)
            n685 = for {
              tunnel: w1454 -> [w1463]
              tunnel: [w1460] -> w1449 mode=indexing
              tunnel: w1450 -> [w1459] mode=indexing
              tunnel: u32 0 -> [w1458]
              i -> [w1464]
              n686 = Increment(x=w1464) -> (x+1=w1461:i32)
              n687 = Quotient & Remainder(x=w1461, y=w1463) -> (x-y*floor(x/y)=w1462:i32)  [unwired: 1 out]
              n688 = case shown="0" w1462 {
                tunnel: [w1465 w1466] -> w1460
                tunnel: w1459 -> [_ w1466]
                tunnel: w1458 -> [w1465 _]
                frame 0 {
                }
                frame 1, Default {
                }
              }
            }
            n689 = property on="Intensity Graph" class="IntGraph (strict)"("Ignore Array"=TRUE ("Write Attribute"), "Color Table"=w1449) -> ()  [unwired: 2 in, 2 out]
          }
          frame #11 {
            n690 = global read "Results_plotter_Global.vi" "Raw Interpolation"() -> (w1468:dbl[][])
            n691 = Add Array Elements(numeric array=w1468) -> (sum=w1467:dbl)
            n692 = Array Size(array=w1468) -> (size(s)=w1478:i32[])
            n693 = Decrement(x=w1478) -> (x-1=w1476:i32[])
            n694 = Index Array(array=w1476, index=0) -> (element=w1477:i32)
            n695 = Index Array(array=w1476, index=1) -> (element=w1473:i32)
            n696 = for {
              N: w1477 -> [_]
              tunnel: w1468 -> [w1486]
              tunnel: w1473 -> [w1485]
              shift-right: [w1481] -> w1470
              shift-left: 0.0 -> [w1482]
              shift-right: [w1480] -> w1469
              shift-left: 0 -> [w1479]
              i -> [w1484]
              n697 = Increment(x=w1484) -> (x+1=w1483:i32)
              n698 = for {
                N: w1485 -> [_]
                tunnel: w1486 -> [w1495]
                tunnel: w1484 -> [w1500]
                tunnel: w1483 -> [w1498]
                shift-right: [w1491] -> w1481
                shift-left: w1482 -> [w1490]
                shift-right: [w1487] -> w1480
                shift-left: w1479 -> [w1488]
                i -> [w1499]
                n699 = Increment(x=w1499) -> (x+1=w1497:i32)
                n700 = Index Array(array=w1495, index (row)=w1500, index (col)=w1497) -> (element=w1496:dbl)
                n701 = Index Array(array=w1495, index (row)=w1498, index (col)=w1497) -> (element=w1493:dbl)
                n702 = Index Array(array=w1495, index (row)=w1500, index (col)=w1499) -> (element=w1501:dbl)
                n703 = Index Array(array=w1495, index (row)=w1498, index (col)=w1499) -> (element=w1494:dbl)
                n704 = Compound Arithmetic op=ADD(w1501, w1496, w1494, w1493) -> (w1489:dbl)
                n705 = Not A Number/Path/Refnum?(number/path/refnum=w1489) -> (NaN/Path/Refnum?=w1492:bool)
                n706 = case shown="False" w1492 {
                  tunnel: [w1505 w1509] -> w1491
                  tunnel: w1490 -> [w1507 w1509]
                  tunnel: w1489 -> [w1506 _]
                  tunnel: [w1504 w1508] -> w1487
                  tunnel: w1488 -> [w1503 w1508]
                  frame False {
                    n707 = Add(x=w1506, y=w1507) -> (x+y=w1505:dbl)
                    n708 = Add(x=1, y=w1503) -> (x+y=w1504:i32)
                  }
                  frame True {
                  }
                }
              }
            }
          }
          frame #12 {
            n709 = local read "Resolution"() -> (w1522:dbl)
            n710 = Divide(x=w1520, y=4.0) -> (x/y=w1518:dbl)
            n711 = Multiply(x=w1522, y=w1522) -> (x*y=w1514:dbl)
            n712 = Multiply(x=w1514, y=w1513) -> ()  [unwired: 1 out]
            n713 = Multiply(x=w1514, y=w1521) -> (x*y=w1515:dbl)
            "Surface Area" <- w1515
            n714 = Multiply(x=w1514, y=w1518) -> (x*y=w1511:dbl)
            "Surface Integral" <- w1511
            n715 = global write "Results_plotter_Global.vi" "Surface Area"(w1515) -> ()
            n716 = global write "Results_plotter_Global.vi" "Surface Integral"(w1511) -> ()
            n717 = Divide(x=16666667, y=w1511) -> (x/y=→"Uadvec":dbl)
            n718 = Divide(x=w1511, y=w1515) -> (x/y=→"Surface Average":dbl)
          }
        }
      }
      frame "Analyse Plot Space" {
        n719 = case shown="True" "Show Plot Space Analysis" {
          tunnel: w1527 -> [_ w1537]
          tunnel: w1524 -> [_ w1536]
          frame False {
          }
          frame True {
            w1533 = TRUE  # Summarise All
            n720 = global read "Results_plotter_Global.vi" "Plot Index values"() -> (w1531:dbl[][])
            n721 = Index Array(array=w1531, index (row)=2) -> (element=w1530:dbl[])  [unwired: 1 in]
            n722 = To Long Integer(number=w1530) -> (32bit integer=w1529:i32[])
            n723 = for {
              tunnel: w1529 -> [w1540] mode=indexing
              tunnel: w1537 -> [w1539]
              tunnel: [w1538] -> w1534 mode=indexing
              n724 = Index Array(array=w1539, index (row)=w1540) -> (element=w1538:string[])  [unwired: 1 in]
            }
            n725 = call "Summarise.vi"("Channel Names"=w1536, "Data"=w1534, "Summarise All"=w1533) -> ("Summary"=w1535:string[][])  [unwired: 2 in]
            n726 = call "Plot_Space_Analysis.vi"("Table"=w1535) -> ()
          }
        }
      }
      frame "Vector Plot" {
        n727 = flat-sequence {
          tunnel: w1545 -> [w1547]
          tunnel: w1543 -> [w1546]
          frame #0 {
            n728 = local read "Template"() -> (w1548:path)
            n729 = call "Vector_Plotting.vi"("Template Filename"=w1548, "Data"=w1546, "Channel Names"=w1547) -> ()  [unwired: 1 out]
          }
          frame #1 {
            n730 = local write "Vector Plot?"(FALSE ("Vector Plot?")) -> ()
          }
        }
      }
      frame "What to do next?" {
        n731 = local read "Warning!"() -> (w1558:string)
        n732 = Empty String/Path?(string/path=w1558) -> (empty?=w1557:bool)
        n733 = Not(x=w1557) -> (.not. x?=w1556:bool)
        n734 = property on="Warning!" class="Str" props=["Visible", "Blinking", "Caption"]("Visible"=w1556, "Blinking"=w1556) -> ()  [unwired: 2 in, 3 out]
        n735 = case shown="False" "Add results file" {
          tunnel: [w1580 "More files options"] -> w1561
          tunnel: "Add results file" -> [_ _]
          tunnel: "Edit Template File" -> [w1571 _]
          frame False {
            n736 = Select(t="Edit template file", s=w1571, f="What to do next 2nd?") -> (s? t:f=w1569:string)
            n737 = Or(x="Save Plot data", y="Save Surface Fit") -> (x .or. y?=w1573:bool)
            n738 = Select(t="Save Plot Data", s=w1573, f=w1569) -> (s? t:f=w1576:string)
            n739 = Select(t="Create Plot summary", s="Save Plot as jpg", f=w1576) -> (s? t:f=w1567:string)
            n740 = Select(t="Save Data in Rows", s="Save Data in Rows", f=w1567) -> (s? t:f=w1580:string)
          }
          frame True {
            n741 = local write "Add results file"(FALSE) -> ()
          }
        }
        n742 = Select(t="End", s="stop", f=w1561) -> (s? t:f=w1552:string)
        n743 = Select(t="Vector Plot", s="Vector Plot?", f=w1552) -> (s? t:f=w1551:string)
      }
      frame "What to do next 2nd?" {
        n744 = local read "Empty"() -> (w1603:bool)
        n745 = local read "Last used Template"() -> (w1591:path)
        n746 = local read "Template"() -> (w1583:path)
        n747 = Select(t="Empty Results file array", s=w1603, f="What to do next 3rd?") -> (s? t:f=w1586:string)
        n748 = global write "Results_plotter_Global.vi" "Template"(w1583) -> ()
        n749 = Not Equal?(x=w1591, y=w1583) -> (x != y?=w1590:bool)
        n750 = Select(t="What type of row averaging?", s="Save Averaged rows", f=w1586) -> (s? t:f=w1598:string)
        n751 = case shown="True" "Delete Plotted data from file" {
          tunnel: [w1631 "Full Res file manipulator" ("t")] -> w1596
          tunnel: w1598 -> [w1631 _]
          frame False {
          }
          frame True {
            n752 = local write "Plotted rows only?"(TRUE ("Save Plotted rows only?")) -> ()
            n753 = local write "Mode"(Plotter_Mode."Delete unwanted rows" ("Mode")) -> ()
          }
        }
        n754 = case shown="True" "Add /Edit metadata" {
          tunnel: [w1608 w1623] -> w1588
          tunnel: w1596 -> [w1609 w1624]
          tunnel: w1594 -> [_ w1622]
          tunnel: "Reload Files" -> [w1610 _]
          tunnel: [string[] [] ("New Chs Out") w1616] -> w1585
          tunnel: [string[][] [] w1615] -> w1584
          frame False {
            n755 = Select(t="Initialise", s=w1610, f=w1609) -> (s? t:f=w1608:string)
          }
          frame True {
            n756 = local read "Result files to read"() -> (w1617:path[])
            n757 = call "Edit_Channel_Panel.vi"("All Channel names"=w1622, "Result files to read"=w1617) -> ("New Values Out"=w1630:string[], "New Chs Out"=w1616:string[], "Cancel Out"=w1619:bool, "Edit Raw Data Header Info Out"=w1613:bool, "Plotted rows only?"=w1629:bool, "Edit Raw data files?"=→"Edit Raw DF?":bool, "Raw data files in Orig Positions?"=→"Raw DF in Orig Pos?":bool, "Mode"=w1627:T1)  [unwired: 6 out]
            "Edit Raw Data Header Info" <- w1613
            n758 = Array Size(array=w1616) -> (size(s)=w1626:i32)
            n759 = Build Array(w1630) -> (w1615:string[][])
            n760 = local write "Add /Edit metadata"(FALSE ("Add /Edit metadata")) -> ()
            n761 = Greater Than 0?(x=w1626) -> (x > 0?=w1614:bool)
            n762 = local write "Plotted rows only?"(w1629) -> ()
            n763 = Or(x=w1613, y=w1614) -> (x .or. y?=w1612:bool)
            n764 = local write "Mode"(w1627) -> ()
            n765 = Compound Arithmetic op=AND(invert w1619, w1612) -> (w1618:bool)
            n766 = Select(t="Full Res file manipulator", s=w1618, f=w1624) -> (s? t:f=w1623:string)
          }
        }
        n767 = global write "Results_plotter_Global.vi" "New Chs In"(w1585) -> ()
        n768 = global write "Results_plotter_Global.vi" "New Values In"(w1584) -> ()
        n769 = Select(t="Initialise", s=w1590, f=w1588) -> (s? t:f=w1587:string)
      }
      frame "What to do next 3rd?" {
        n770 = local read "Show Results Space Analysis"() -> (w1646:bool)
        n771 = local read "Show Plot Space Analysis"() -> (w1645:bool)
        n772 = while {
          shift-right: [w1669] -> _
          shift-left: _ -> [w1668]
          shift-left: _ -> [w1667]
          shift-left: _ -> [w1666]
          tunnel: w1646 -> [w1669]
          shift-right: [w1674] -> _
          shift-left: _ -> [w1673]
          shift-left: _ -> [w1672]
          shift-left: _ -> [w1671]
          tunnel: w1645 -> [w1674]
          tunnel: [w1670] -> w1644
          tunnel: [w1665] -> w1643
          stop <- TRUE stop-if-true
          n773 = Compound Arithmetic op=AND(w1669, w1668, w1667, w1666) -> (w1665:bool)
          n774 = Compound Arithmetic op=AND(w1674, w1673, w1672, w1671) -> (w1670:bool)
        }
        n775 = Select(t="Run Calculation Routine", s="Calculate new metadata", f="Time to save setup?") -> (s? t:f=w1652:string)
        n776 = case shown="True" w1644 {
          frame False {
          }
          frame True {
            n777 = Open VI Reference(vi path="Plot_Space_Analysis.vi" ("VI path")) -> (vi reference=w1686:refnum<vi>, error out=w1685:errorcluster)  [unwired: 1 in, 4 out]
            n778 = property class="VI"(reference=w1686, error in=w1685) -> (reference out=w1684:refnum<vi>, error out=w1683:errorcluster, "Front Panel Window:Open"=w1681:bool)
            n779 = local write "Show Plot Space Analysis"(w1681) -> ()
            n780 = Close Reference(reference=w1684, error in (no error)=w1683) -> ()  [unwired: 1 out]
          }
        }
        n781 = case shown="True" w1643 {
          frame False {
          }
          frame True {
            n782 = Open VI Reference(vi path="Results_Space_Analysis.vi" ("VI path")) -> (vi reference=w1680:refnum<vi>, error out=w1679:errorcluster)  [unwired: 1 in, 4 out]
            n783 = property class="VI"(reference=w1680, error in=w1679) -> (reference out=w1678:refnum<vi>, error out=w1677:errorcluster, "Front Panel Window:Open"=w1675:bool)
            n784 = local write "Show Results Space Analysis"(w1675) -> ()
            n785 = Close Reference(reference=w1678, error in (no error)=w1677) -> ()  [unwired: 1 out]
          }
        }
        n786 = Select(t="Save Setup", s="Save Setup", f=w1652) -> (s? t:f=w1649:string)
        n787 = Select(t="Choose Setup file", s="Load Setup", f=w1649) -> (s? t:f=w1642:string)
        n788 = Or(x="Kill Point", y="Process Point") -> (x .or. y?=w1639:bool)
        n789 = Select(t="Process cursor point", s=w1639, f=w1642) -> (s? t:f=w1635:string)
        n790 = case shown="True" "Post Process Plotted Data" {
          tunnel: [w1660 "Full Res file manipulator" ("t")] -> w1636
          tunnel: w1635 -> [w1660 _]
          frame False {
          }
          frame True {
            n791 = local write "Plotted rows only?"(TRUE ("Plotted rows only?")) -> ()
            n792 = local write "Mode"(Plotter_Mode."Post Process Plotted Rows" ("Mode")) -> ()
          }
        }
      }
      frame "Time to save setup?" {
        n793 = stacked-sequence {
          seq-local: [w1696 _] -> [_ w1737]
          seq-local: [w1695 _] -> [_ w1736]
          tunnel: [w1704 _] -> w1689
          tunnel: w1688 -> [w1694 _]
          tunnel: [w1693 _] -> w1687
          frame #0 {
            n794 = while {
              shift-right: [w1726] -> _
              shift-left: _ -> [w1724]
              shift-right: [w1713] -> _
              shift-left: _ -> [w1721]
              tunnel: [w1713] -> w1703
              tunnel: [w1712] -> w1702
              shift-right: [w1714] -> _
              shift-left: _ -> [w1720]
              tunnel: [w1718] -> w1697
              tunnel: [w1715] -> w1698
              tunnel: [w1714] -> w1699
              tunnel: [w1711] -> w1695
              tunnel: w1694 -> [w1706]
              tunnel: [w1705] -> w1693
              stop <- FALSE continue-if-true
              n795 = Get Date/Time In Seconds() -> (seconds since 1Jan1904=w1722:timestamp)
              n796 = To Double Precision Float(number=w1722) -> (double precision float=w1725:dbl)
              n797 = local read "Show Plot Space Analysis"() -> (w1714:bool)
              n798 = Subtract(x=w1725, y=w1724) -> (x-y=w1728:dbl)
              n799 = local read "Show Results Space Analysis"() -> (w1713:bool)
              n800 = Greater?(x=w1728, y=200.0) -> (0:w1709:bool)
              n801 = Greater?(x=w1706, y=300) -> (0:w1708:bool)
              n802 = And(x=w1709, y=w1708) -> (x .and. y?=w1707:bool)
              n803 = case shown="True" w1707 {
                tunnel: [w1731 w1735] -> w1726
                tunnel: w1725 -> [_ w1735]
                tunnel: w1724 -> [w1731 _]
                tunnel: ["Check modification dates?" "Save Setup"] -> w1717
                tunnel: [TRUE w1732] -> w1705
                frame False {
                }
                frame True {
                  n804 = global read "Trav_pos_global.vi" "Estimated Completion time"() -> (w1734:string)
                  n805 = Empty String/Path?(string/path=w1734) -> (empty?=w1732:bool)
                }
              }
              n806 = Not Equal?(x=w1714, y=w1720) -> (x != y?=w1715:bool)
              n807 = Not Equal?(x=w1713, y=w1721) -> (x != y?=w1712:bool)
              n808 = Compound Arithmetic op=AND(invert w1713, w1712) -> (w1711:bool)
              n809 = And(x=w1714, y=w1715) -> (x .and. y?=w1719:bool)
              n810 = Select(t="Analyse Plot Space", s=w1719, f=w1717) -> (s? t:f=w1718:string)
            }
            n811 = Compound Arithmetic op=AND(invert w1699, w1698) -> (w1696:bool)
            n812 = And(x=w1703, y=w1702) -> (x .and. y?=w1701:bool)
            n813 = Select(t="What is present?", s=w1701, f=w1697) -> (s? t:f=w1704:string)
          }
          frame #1 {
            n814 = case shown="True" w1736 {
              frame False {
              }
              frame True {
                n815 = Open VI Reference(vi path="Results_Space_Analysis.vi" ("VI path")) -> (vi reference=w1743:refnum<vi>, error out=w1742:errorcluster)  [unwired: 1 in, 4 out]
                n816 = property class="VI"(reference=w1743, error in=w1742, "Front Panel Window:Open"=FALSE) -> (reference out=w1741:refnum<vi>, error out=w1740:errorcluster)
                n817 = Close Reference(reference=w1741, error in (no error)=w1740) -> ()  [unwired: 1 out]
              }
            }
            n818 = case shown="True" w1737 {
              frame False {
              }
              frame True {
                n819 = Open VI Reference(vi path="Plot_Space_Analysis.vi" ("VI path")) -> (vi reference=w1749:refnum<vi>, error out=w1748:errorcluster)  [unwired: 1 in, 4 out]
                n820 = property class="VI"(reference=w1749, error in=w1748, "Front Panel Window:Open"=FALSE) -> (reference out=w1747:refnum<vi>, error out=w1746:errorcluster)
                n821 = Close Reference(reference=w1747, error in (no error)=w1746) -> ()  [unwired: 1 out]
              }
            }
          }
        }
      }
      frame "Check modification dates?" {
        n822 = while {
          shift-right: [w1769] -> _
          shift-left: _ -> [w1767]
          tunnel: [w1766] -> w1758
          stop <- FALSE continue-if-true
          n823 = Get Date/Time In Seconds() -> (seconds since 1Jan1904=w1764:timestamp)
          n824 = To Double Precision Float(number=w1764) -> (double precision float=w1768:dbl)
          n825 = Subtract(x=w1768, y=w1767) -> (x-y=w1772:dbl)
          n826 = Greater?(x=w1772, y=200.0) -> (0:w1770:bool)
          n827 = case shown="True" w1770 {
            tunnel: [w1774 w1777] -> w1769
            tunnel: w1768 -> [_ w1777]
            tunnel: w1767 -> [w1774 _]
            tunnel: [FALSE w1775] -> w1766
            frame False {
            }
            frame True {
              n828 = global read "Results_plotter_Global.vi" "First Loop"() -> (w1776:bool)
              n829 = Not(x=w1776) -> (.not. x?=w1775:bool)
            }
          }
        }
        n830 = Equal?(x="Tab Control", y=enum32{"Load ", "Plot ", "Save ", "Cursor"}."Cursor" ("Tab Control")) -> (x = y?=w1754:bool)
        n831 = global write "Results_plotter_Global.vi" "First Loop"(FALSE) -> ()
        n832 = Select(t="Read Cursor", s=w1754, f="Ordinate Selector Type") -> (s? t:f=w1752:string)
        n833 = Select(t="Files Modified?", s=w1758, f=w1752) -> (s? t:f=w1757:string)
      }
      frame "Files Modified?" {
        n834 = local read "No Of Rows"() -> (w1781:i32)
        n835 = Less?(x=w1781, y=w1780) -> (x < y?=w1778:bool)
        n836 = case shown="False" w1778 {
          tunnel: [w1787 w1793] -> w1782
          tunnel: "Ordinate Selector Type" -> [w1787 w1788]
          frame False {
          }
          frame True {
            n837 = local read "Result files to read"() -> (w1792:path[])
            n838 = for {
              tunnel: w1792 -> [w1796] mode=indexing
              tunnel: [w1794] -> w1791 mode=indexing
              n839 = call "File_Modified_Since_Check.vi"("Pathname"=w1796, "Just Modified?"=TRUE) -> ("Modified?"=w1794:bool)
            }
            n840 = Or Array Elements(Boolean array=w1791) -> (logical OR=w1790:bool)
            n841 = Select(t="Initialise", s=w1790, f=w1788) -> (s? t:f=w1793:string)
          }
        }
      }
      frame "Read Cursor" {
        n842 = stacked-sequence {
          seq-local: [w1802 _] -> [_ w1837]
          tunnel: ["Ordinate Selector Type" _] -> w1800
          tunnel: [TRUE _] -> w1799
          tunnel: w1798 -> [_ w1836]
          tunnel: w1797 -> [_ w1835]
          frame #0 {
            n843 = property on="XY Plot" class="XYGraph (strict)"() -> ("Cursor.Cursor Position:Cursor X"=w1804:dbl, "Cursor.Cursor Position:Cursor Y"=w1803:dbl)  [unwired: 2 in, 2 out]
            n844 = local read "Transpose"() -> (w1817:bool)
            n845 = global read "Results_plotter_Global.vi" "Plot Index values"() -> (w1810:dbl[][])
            n846 = Index Array(array=w1810, index (row)=1) -> (element=w1808:dbl[])  [unwired: 1 in]
            n847 = Index Array(array=w1810, index (row)=2) -> (element=w1807:dbl[])  [unwired: 1 in]
            n848 = Index Array(array=w1810, index (row)=0) -> (element=w1809:dbl[])  [unwired: 1 in]
            n849 = case shown="True" w1817 {
              tunnel: [w1821 w1823] -> w1816
              tunnel: w1804 -> [w1821 w1822]
              tunnel: [w1820 w1822] -> w1815
              tunnel: w1803 -> [w1820 w1823]
              frame False {
              }
              frame True {
              }
            }
            n850 = for {
              tunnel: w1816 -> [w1832]
              tunnel: w1815 -> [w1831]
              tunnel: [w1826] -> w1814 mode=indexing
              tunnel: w1809 -> [w1825] mode=indexing
              tunnel: w1808 -> [w1824] mode=indexing
              n851 = Subtract(x=w1832, y=w1825) -> (x-y=w1830:dbl)
              n852 = Subtract(x=w1831, y=w1824) -> (x-y=w1829:dbl)
              n853 = Multiply(x=w1830, y=w1830) -> (x*y=w1827:dbl)
              n854 = Multiply(x=w1829, y=w1829) -> (x*y=w1828:dbl)
              n855 = Add(x=w1827, y=w1828) -> (x+y=w1826:dbl)
            }
            n856 = Array Max & Min(array=w1814) -> (min index (indices)=w1806:i32)  [unwired: 3 out]
            n857 = Index Array(array=w1807, index=w1806) -> (element=w1805:dbl)
            n858 = To Long Integer(number=w1805) -> (32bit integer=w1802:i32)
            "Cursor index" <- w1802
          }
          frame #1 {
            n859 = Index Array(array=w1836, index (row)=w1837) -> (element=w1834:string[])  [unwired: 1 in]
            n860 = for {
              tunnel: w1835 -> [w1845] mode=indexing
              tunnel: w1834 -> [w1838] mode=indexing
              tunnel: [w1844] -> w1833 mode=indexing
              n861 = while {
                shift-right: [w1857] -> _
                shift-left: w1838 -> [w1858]
                tunnel: [w1854] -> w1842
                tunnel: [w1853] -> w1840 mode=indexing
                i -> [w1854]
                stop <- w1855 continue-if-true
                n862 = Match Pattern(string=w1858, regular expression=":") -> (before substring=w1853:string, after substring=w1857:string, offset past match=w1856:i32)  [unwired: 2 out]
                n863 = Greater Than 0?(x=w1856) -> (x > 0?=w1855:bool)
              }
              n864 = Greater?(x=w1842, y=2) -> (0:w1841:bool)
              n865 = Reverse 1D Array(array=w1840) -> (reversed array=w1839:string[])
              n866 = case shown="True" w1841 {
                tunnel: w1845 -> [w1848 w1852]
                tunnel: [w1846 w1851] -> w1844
                tunnel: w1839 -> [_ w1850]
                tunnel: w1838 -> [w1847 w1849]
                frame False {
                  n867 = Build Array(w1848, w1847) -> (w1846:string[])
                }
                frame True {
                  n868 = Build Array (concatenate)(w1852, w1850, w1849) -> (w1851:string[])
                }
              }
            }
            "Table" <- w1833
          }
        }
      }
      frame "Process Cursor Point" {
        n869 = stacked-sequence {
          tunnel: [w1881] -> w1864
          tunnel: [TRUE] -> w1863
          tunnel: w1862 -> [_]
          tunnel: w1861 -> [_]
          tunnel: w1860 -> [w1882]
          frame #0 {
            w1873 = FALSE  # Add Extra Channels?
            w1874 = FALSE  # Read Channel Names only
            n870 = local read "Kill Point"() -> (w1883:bool)
            n871 = local read "Cursor index"() -> (w1889:i32)
            n872 = global read "Results_plotter_Global.vi" "Row Reference"() -> (w1890:i32[][])
            n873 = Index Array(array=w1890, index (row)=w1889) -> (element=w1884:i32[])  [unwired: 1 in]
            n874 = local read "Result files to read"() -> (w1888:path[])
            n875 = Index Array(array=w1884, index=0) -> (element=w1887:i32)
            n876 = Index Array(array=w1884, index=1) -> (element=w1868:i32)
            n877 = Index Array(array=w1888, index=w1887) -> (element=w1872:path)
            n878 = global read "Constants_global.vi" "Run VI Folder"() -> (w1877:path)
            n879 = Strip Path(path=w1877) -> (stripped path=w1878:path)  [unwired: 1 out]
            n880 = Build Path(base path=w1878, name or relative path="Data_plotting_vis") -> (appended path=w1879:path)
            n881 = Build Path(base path=w1879, name or relative path="RD_Files.tpt") -> (appended path=w1875:path)
            n882 = call "Read_Data_file.vi"("Results file"=w1872, "Read Channel Names only"=w1874, "Add Extra Channels?"=w1873, "Template File"=w1875) -> ("Channel Values Out"=w1869:string[][])  [unwired: 1 in, 14 out]
            n883 = Index Array(array=w1869, index (col)=0 ("index (row)")) -> (element=w1871:string[])  [unwired: 1 in]
            n884 = Index Array(array=w1871, index=w1868) -> (element=w1867:string)
            n885 = call "String_to_Pathname.vi"("Input String"=w1867) -> ("path"=w1866:path)
            n886 = case shown="False" w1883 {
              tunnel: w1872 -> [_ w1902]
              tunnel: w1868 -> [_ w1898]
              tunnel: w1882 -> [_ w1905]
              tunnel: ["What to do next?" ("t") w1904] -> w1881
              tunnel: w1866 -> [w1892 w1896]
              frame False {
                n887 = call "Post_Process_Measurement.vi"("Raw data file"=w1892) -> ()  [unwired: 1 out]
                n888 = local write "Process Point"(FALSE ("Kill Point")) -> ()
              }
              frame True {
                n889 = Strip Path(path=w1902) -> (name=w1897:string)  [unwired: 1 out]
                n890 = Strip Path(path=w1896) -> (name=w1895:string)  [unwired: 1 out]
                n891 = local read "No Of Rows"() -> (w1907:i32)
                n892 = Format Into String(format string="Are you sure you want to remove the row in the results file \"%s\" generated from the raw data filename \"%s\"?", w1897, w1895) -> (resulting string=w1900:string)  [unwired: 2 in, 1 out]
                n893 = Less?(x=w1907, y=w1905) -> (x < y?=w1906:bool)
                n894 = Two Button Dialog(message=w1900) -> (T button?=w1899:bool)  [unwired: 2 out]
                n895 = case shown="False" w1906 {
                  tunnel: ["Create Selectors" "Initialise" ("t")] -> w1904
                  frame False {
                  }
                  frame True {
                  }
                }
                n896 = case shown="True" w1899 {
                  tunnel: w1902 -> [_ w1909]
                  tunnel: w1898 -> [_ w1908]
                  frame False {
                  }
                  frame True {
                    n897 = Build Array(w1908) -> (w1910:i32[])
                    n898 = call "Delete_unwanted_rows.vi"("Selected Rows"=w1910, "Filename"=w1909) -> ()  [unwired: 1 out]
                  }
                }
                n899 = local write "Kill Point"(FALSE ("Kill Point")) -> ()
              }
            }
          }
        }
      }
      frame "Edit template file" {
        n900 = stacked-sequence {
          frame #0 {
            n901 = local read "Template"() -> (w1919:path)
            n902 = call "Valid_Path.vi"("Filename"=w1919) -> ("Valid Path?"=w1918:bool)
            n903 = case shown="False" w1918 {
              tunnel: [T7."Edit Existing Template File" ("Mode") T7."Create New Template File" ("Mode")] -> w1922
              frame True {
              }
              frame False {
              }
            }
            n904 = local read "Results file"() -> (w1921:path)
            n905 = call "Edit_Template_File.vi"("Mode"=w1922, "Template Filename"=w1919, "Data Filename"=w1921) -> ("Template Filename Out"=w1920:path)  [unwired: 12 out]
            n906 = local write "Template"(w1920) -> ()
          }
          frame #1 {
            n907 = local read "Job Directory"() -> (w1925:path)
            n908 = Path To String(path=w1925) -> (string=w1928:string)
            n909 = call "Read_Write_Template.vi"("Mode"=Global_mode."Write Global to File", "Single Value In"=w1928, "Data type"="Log Folder Name" ("Variable name")) -> ()  [unwired: 5 in, 8 out]
            n910 = local write "Edit Template File"(FALSE ("Edit Template File")) -> ()
            n911 = Current VI's Path() -> (path=w1931:path)
            n912 = call "Open_Close_Front_Panel.ph.vi"("Front Panel Window:Open"=TRUE, "VI path"=w1931) -> ()  [unwired: 2 out]
          }
        }
      }
      frame "Save Plot Data" {
        n913 = global read "Results_plotter_Global.vi" "XY Graph Cluster"() -> (w1932:cluster{dbl[], dbl[]}[])
        n914 = local read "Tolerances"() -> (w1939:dbl[])
        n915 = local read "Absisca"() -> (w1938:u16)
        n916 = local read "Transpose"() -> (w1937:bool)
        n917 = local read "Multi Ordinate"() -> (w1936:i32[])
        n918 = global read "Results_plotter_Global.vi" "Precision"() -> (w1933:string[])
        n919 = stacked-sequence {
          seq-local: [w1950 _ _ _ _ _ _ _ _] -> [_ w1975 _ w2013 _ _ _ _ _]
          seq-local: [_ w1971 _ _ _ _ _ _ _] -> [_ _ _ _ _ _ _ w2135 _]
          seq-local: [_ _ _ _ _ w2065 _ _ _] -> [_ _ _ _ _ _ _ w2134 _]
          seq-local: [_ _ _ _ _ w2067 _ _ _] -> [_ _ _ _ _ _ w2103 _ _]
          seq-local: [_ _ _ w2011 _ _ _ _ _] -> [_ _ _ _ _ _ w2104 _ _]
          seq-local: [_ _ _ _ w2034 _ _ _ _] -> [_ _ _ _ _ w2060 _ _ _]
          seq-local: [w1947 _ _ _ _ _ _ _ _] -> [_ _ _ _ _ _ _ _ w2140]
          seq-local: [w1946 _ _ _ _ _ _ _ _] -> [_ w1963 _ _ _ _ _ _ _]
          seq-local: [_ _ w1992 _ _ _ _ _ _] -> [_ _ _ w2012 _ _ w2105 _ _]
          seq-local: [_ _ _ _ _ _ w2101 _ _] -> [_ _ _ _ _ _ _ w2132 _]
          tunnel: [_ _ _ _ _ _ _ _ TRUE] -> w1945
          tunnel: [_ _ _ _ _ _ _ _ w2138] -> w1944
          tunnel: w1942 -> [_ _ _ _ _ w2063 _ _ _]
          tunnel: w1943 -> [_ w1968 _ _ _ w2066 _ _ _]
          tunnel: [_ _ _ _ _ w2066 _ _ _] -> w1941
          tunnel: [_ _ _ _ _ w2063 _ _ _] -> w1940
          tunnel: w1939 -> [w1952 _ _ _ w2039 w2064 _ _ _]
          tunnel: w1932 -> [w1951 _ _ w2015 _ _ _ _ _]
          tunnel: w1938 -> [w1949 w1985 _ _ w2041 _ _ _ _]
          tunnel: w1937 -> [w1948 _ _ w2014 _ _ _ _ _]
          tunnel: w1936 -> [_ _ _ _ w2038 _ _ _ _]
          tunnel: [_ _ _ w2009 _ _ _ _ _] -> w1935
          tunnel: w1934 -> [_ _ w1995 w2009 _ _ _ _ _]
          tunnel: w1933 -> [_ _ _ w2008 _ w2059 _ _ _]
          frame #0 {
            n920 = local read "Save Surface Fit"() -> (w1947:bool)
            n921 = Not(x=w1948) -> (.not. x?=w1955:bool)
            n922 = for {
              tunnel: w1951 -> [w1962] mode=indexing
              tunnel: w1955 -> [w1959]
              shift-right: [w1957] -> w1953
              shift-left: dbl[] [] -> [w1958]
              n923 = Unbundle(w1962) -> (w1961:dbl[], w1960:dbl[])
              n924 = Select(t=w1961, s=w1959, f=w1960) -> (s? t:f=w1956:dbl[])
              n925 = Build Array (concatenate)(w1958, w1956) -> (w1957:dbl[])
            }
            n926 = Index Array(array=w1952, index=w1949) -> (element=w1946:dbl)
            n927 = call "Numeric_bins.vi"("Values"=w1953, "Tolerance"=w1946) -> ("Bin Centres"=w1950:dbl[])  [unwired: 2 out]
          }
          frame #1 {
            n928 = Index Array(array=w1968, index=w1985) -> (element=w1988:string)
            n929 = Match Pattern(string=w1988, regular expression=":") -> (before substring=w1987:string, after substring=w1986:string)  [unwired: 3 out]
            n930 = Concatenate Strings(w1987, " ", w1986, " =:" ("regular expression")) -> (w1970:string)
            n931 = Greater?(x=w1963, y=0.4) -> (0:w1983:bool)
            n932 = Greater?(x=w1963, y=0.09) -> (0:w1978:bool)
            n933 = call <vilib>:"Trim Whitespace.vi"("string"=w1970) -> ("trimmed string"=w1969:string)  [unwired: 1 in]
            n934 = Select(t=i16 0 ("precision (6)"), s=w1983, f=i16 2 ("precision (6)")) -> (s? t:f=w1979:i16)
            n935 = Select(t=w1979, s=w1978, f=i16 3) -> (s? t:f=w1976:i16)
            n936 = Number To Fractional String(number=w1975, precision (6)=w1976) -> (F-format string=w1974:string[])  [unwired: 2 out]
            n937 = for {
              tunnel: w1969 -> [w1991]
              tunnel: w1974 -> [w1989] mode=indexing
              tunnel: [w1990] -> w1973 mode=indexing
              n938 = Concatenate Strings(w1991, w1989) -> (w1990:string)
            }
            n939 = Build Array (concatenate)("Plot:Legend:" ("Input Element"), w1973, "End of:Plot Series:" ("Input Element")) -> (w1971:string[])
          }
          frame #2 {
            n940 = local read "Multi Ordinate?"() -> (w1994:bool)
            n941 = global read "Results_plotter_Global.vi" "Legend"() -> (w1993:string[])
            n942 = case shown="False" w1994 {
              tunnel: w1995 -> [w1999 _]
              tunnel: [w1996 w2007] -> w1992
              tunnel: w1993 -> [w1998 w2007]
              frame False {
                n943 = local read "Multi Ordinate"() -> (w2002:i32[])
                n944 = Index Array(array=w2002, index=0 ("Index")) -> (element=w2000:i32)
                n945 = Index Array(array=w1999, index=w2000) -> (element=w1997:string)
                n946 = for {
                  tunnel: w1998 -> [w2006] mode=indexing
                  tunnel: w1997 -> [w2005]
                  tunnel: [w2003] -> w1996 mode=indexing
                  n947 = Format Into String(format string="; %s", initial string=w2005, w2006) -> (resulting string=w2003:string)  [unwired: 1 in, 1 out]
                }
              }
              frame True {
              }
            }
          }
          frame #3 {
            n948 = call "Grid_Data.vi"("Transpose"=w2014, "XY Graph"=w2015, "Bin Centres"=w2013) -> ("Grided data"=w2010:dbl[][])  [unwired: 1 out]
            n949 = for {
              tunnel: w2012 -> [w2022] mode=indexing
              tunnel: [w2024] -> w2011 mode=indexing
              tunnel: w2010 -> [w2023] mode=indexing
              tunnel: w2009 -> [w2018]
              tunnel: w2008 -> [w2017]
              n950 = Match Pattern(string=w2022, regular expression=";") -> (before substring=w2019:string)  [unwired: 4 out]
              n951 = Search 1D Array(1D array=w2018, element=w2019) -> (index of element=w2020:i32)  [unwired: 1 out]
              n952 = Index Array(array=w2017, index=w2020) -> (element=w2016:string)
              n953 = for {
                tunnel: w2016 -> [w2029]
                tunnel: [w2028] -> w2025 mode=indexing
                tunnel: w2023 -> [w2026] mode=indexing
                n954 = Not A Number/Path/Refnum?(number/path/refnum=w2026) -> (NaN/Path/Refnum?=w2027:bool)
                n955 = case shown="True" w2027 {
                  tunnel: w2029 -> [w2032 _]
                  tunnel: [w2031 ""] -> w2028
                  tunnel: w2026 -> [w2030 _]
                  frame False {
                    n956 = call "Number_2_string.vi"("precision"=w2032, "number"=w2030) -> ("String"=w2031:string)
                  }
                  frame True {
                  }
                }
              }
              n957 = Build Array (concatenate)(w2022, w2025) -> (w2024:string[])
            }
          }
          frame #4 {
            n958 = Index Array(array=w2038, index=0 ("Index")) -> (element=w2036:i32)
            n959 = global read "Results_plotter_Global.vi" "Summarise"() -> (w2035:string[])
            n960 = for {
              shift-right: [w2048] -> w2034
              shift-left: i32[] [] -> [w2049]
              tunnel: w2041 -> [w2054]
              tunnel: w2036 -> [w2053]
              tunnel: w2039 -> [w2046] mode=indexing
              tunnel: w2035 -> [w2044] mode=indexing
              i -> [w2047]
              n961 = Equal?(x=w2053, y=w2047) -> (x = y?=w2052:bool)
              n962 = Not A Number/Path/Refnum?(number/path/refnum=w2046) -> (NaN/Path/Refnum?=w2045:bool)
              n963 = Equal?(x=w2054, y=w2047) -> (x = y?=w2051:bool)
              n964 = Equal?(x="FALSE", y=w2044) -> (x = y?=w2042:bool)
              n965 = Compound Arithmetic op=OR(w2051, w2052, w2045, w2042) -> (w2050:bool)
              n966 = case shown="False" w2050 {
                tunnel: w2049 -> [w2057 w2058]
                tunnel: [w2056 w2058] -> w2048
                tunnel: w2047 -> [w2055 _]
                frame False {
                  n967 = Build Array (concatenate)(w2057, w2055) -> (w2056:i32[])
                }
                frame True {
                }
              }
            }
          }
          frame #5 {
            n968 = local read "Plotted Series"() -> (w2062:bool[][])
            n969 = for {
              tunnel: w2064 -> [w2078]
              tunnel: [w2077] -> w2067 mode=indexing
              tunnel: w2060 -> [w2076]
              tunnel: w2063 -> [w2075]
              tunnel: w2062 -> [w2074] mode=indexing
              tunnel: i32[] [] -> [w2072]
              tunnel: w2059 -> [w2071]
              n970 = for {
                shift-right: [w2080] -> w2073
                shift-left: w2072 -> [w2081]
                tunnel: w2074 -> [w2079] mode=indexing
                i -> [w2082]
                n971 = case shown="True" w2079 {
                  tunnel: w2082 -> [_ w2086]
                  tunnel: w2081 -> [w2083 w2085]
                  tunnel: [w2083 w2084] -> w2080
                  frame False {
                  }
                  frame True {
                    n972 = Build Array (concatenate)(w2085, w2086) -> (w2084:i32[])
                  }
                }
              }
              n973 = for {
                tunnel: w2078 -> [w2094]
                tunnel: [w2095] -> w2077 mode=indexing
                tunnel: w2076 -> [w2089] mode=indexing
                tunnel: w2075 -> [w2092]
                tunnel: w2073 -> [w2091]
                tunnel: w2071 -> [w2088]
                n974 = for {
                  tunnel: w2091 -> [w2100] mode=indexing
                  tunnel: [w2099] -> w2096 mode=indexing
                  tunnel: w2089 -> [w2098]
                  tunnel: w2092 -> [w2097]
                  n975 = Index Array(array=w2097, index (row)=w2100, index (col)=w2098) -> (element=w2099:string)
                }
                n976 = Index Array(array=w2088, index=w2089) -> (element=w2090:string)
                n977 = Index Array(array=w2094, index=w2089) -> (element=w2093:dbl)
                n978 = call "Value_Occurence_Analysis.vi"("Average Numeric Values?"=FALSE, "Tolerance"=w2093, "Precision (3)"=w2090, "String Array"=w2096) -> ("Output String"=w2095:string)  [unwired: 2 out]
              }
            }
            n979 = for {
              tunnel: w2060 -> [w2070] mode=indexing
              tunnel: w2066 -> [w2069]
              tunnel: [w2068] -> w2065 mode=indexing
              n980 = Index Array(array=w2069, index=w2070) -> (element=w2068:string)
            }
          }
          frame #6 {
            n981 = for {
              shift-right: [w2118] -> w2101
              shift-left: string[][] [] -> [w2119]
              shift-right: [w2114] -> _
              shift-left: _ -> [w2115]
              tunnel: w2105 -> [w2116] mode=indexing
              tunnel: w2104 -> [w2108] mode=indexing
              tunnel: w2103 -> [w2107] mode=indexing
              i -> [w2113]
              n982 = Greater Than 0?(x=w2113) -> (x > 0?=w2112:bool)
              n983 = Match Pattern(string=w2116, regular expression="; ") -> (before substring=w2114:string)  [unwired: 4 out]
              n984 = Equal?(x=w2115, y=w2114) -> (x = y?=w2111:bool)
              n985 = Build Array (concatenate)(w2108, "", w2107) -> (w2106:string[])
              n986 = Compound Arithmetic op=AND(w2112, invert w2111) -> (w2110:bool)
              n987 = case shown="True" w2110 {
                tunnel: w2119 -> [w2123 w2126]
                tunnel: [w2122 w2125] -> w2118
                tunnel: w2106 -> [w2121 w2124]
                frame True {
                  n988 = Build Array (concatenate)(w2123, string[] [] ("array"), w2121) -> (w2122:string[][])
                }
                frame False {
                  n989 = Build Array (concatenate)(w2126, w2124) -> (w2125:string[][])
                }
              }
            }
          }
          frame #7 {
            w2131 = TRUE  # Simple Save?
            n990 = Build Array (concatenate)(w2135, w2134) -> (w2133:string[])
            n991 = local read "Header"() -> (w2128:string)
            n992 = call "Write_output_file.vi"("Output filename"="Output Filename", "Header"=w2128, "Channel Names"=w2133, "Data"=w2132, "Simple Save?"=w2131, "Summarise mode"=T8."No data summary") -> ("Output filename Out"=w2129:path)  [unwired: 6 in, 3 out]
            n993 = local write "Output Filename"(w2129) -> ()
          }
          frame #8 {
            n994 = local write "Save Plot data"(FALSE ("Save Plot data")) -> ()
            n995 = local write "Header"("") -> ()
            n996 = Select(t="Save Surface Fit data", s=w2140, f="Create Selectors") -> (s? t:f=w2138:string)
          }
        }
      }
      frame "What type of row averaging?" {
        n997 = Two Button Dialog(message="Do you want to Combine rows with identical positions together?", 1:"Just average series" ("F button name (\"Cancel\")"), 2:"Combine rows" ("T button name (\"OK\")")) -> (T button?=w2146:bool)
        n998 = Select(t="Combine rows" ("T button name (\"OK\")"), s=w2146, f="Average Rows together") -> (s? t:f=w2143:string)
      }
      frame "Combine rows" {
        w2156 = TRUE  # Show panel ?
        n999 = local read "Output Filename"() -> (w2155:path)
        n1000 = call "Combined_file_Panel.vi"("Show panel ?"=w2156, "Output filename"=w2155) -> ("Only Plotted data?"=w2157:bool, "Include Empty Rows? Out"=w2158:bool, "Give Audit Channels Out"=w2159:bool, "Output filename Out"=w2154:path)  [unwired: 5 out]
        n1001 = case shown="False" w2157 {
          tunnel: w2161 -> [w2170 w2173]
          tunnel: [w2170 w2171] -> w2160
          frame False {
          }
          frame True {
            n1002 = global read "Results_plotter_Global.vi" "Plot Index values"() -> (w2175:dbl[][])
            n1003 = Index Array(array=w2175, index (row)=2) -> (element=w2172:dbl[])  [unwired: 1 in]
            n1004 = for {
              tunnel: w2173 -> [w2178]
              tunnel: w2172 -> [w2177] mode=indexing
              tunnel: [w2176] -> w2171 mode=indexing
              n1005 = Index Array(array=w2178, index (row)=w2177) -> (element=w2176:string[])  [unwired: 1 in]
            }
          }
        }
        n1006 = local write "Save Averaged rows"(FALSE ("Save Plot data")) -> ()
        n1007 = local read "X Ch Name"() -> (w2165:u16)
        n1008 = local read "Y Ch Name"() -> (w2166:u16)
        n1009 = local read "Z Ch Name"() -> (w2167:u16)
        n1010 = call "Find_Rows_to_Combine.vi"("Include Empty Rows?"=w2158, "file path (dialog if empty)"=w2154, "Give Audit Channels"=w2159, "Full Channel Names"=w2164, "Data"=w2160, "Z Column Index"=w2167, "Y Column Index"=w2166, "X Column Index"=w2165) -> ()  [unwired: 4 out]
        n1011 = local write "Output Filename"(w2154) -> ()
      }
      frame "Average Rows together" {
        n1012 = global read "Results_plotter_Global.vi" "XY Graph Cluster"() -> (w2180:cluster{dbl[], dbl[]}[])
        n1013 = local read "Tolerances"() -> (w2186:dbl[])
        n1014 = local read "Absisca"() -> (w2185:u16)
        n1015 = local read "Transpose"() -> (w2184:bool)
        n1016 = global read "Results_plotter_Global.vi" "Precision"() -> (w2182:string[])
        n1017 = global read "Results_plotter_Global.vi" "Summarise"() -> (w2181:string[])
        n1018 = stacked-sequence {
          seq-local: [w2198 _ _ _ _] -> [_ w2215 _ _ _]
          seq-local: [_ w2218 _ _ _] -> [_ _ _ w2300 _]
          seq-local: [w2194 _ _ _ _] -> [_ w2216 _ _ _]
          seq-local: [_ _ w2278 _ _] -> [_ _ _ w2294 _]
          tunnel: [_ _ _ _ TRUE] -> w2192
          tunnel: [_ _ _ _ "Create Selectors"] -> w2191
          tunnel: w2189 -> [_ w2221 _ _ w2303]
          tunnel: w2190 -> [_ _ w2279 _ w2302]
          tunnel: [_ _ _ _ w2302] -> w2188
          tunnel: [_ _ _ _ w2303] -> w2187
          tunnel: w2186 -> [w2200 w2219 _ _ _]
          tunnel: w2180 -> [w2199 _ _ _ _]
          tunnel: w2185 -> [w2197 _ _ _ _]
          tunnel: w2184 -> [w2196 _ _ _ _]
          tunnel: w2183 -> [w2193 _ _ _ _]
          tunnel: w2182 -> [_ w2220 _ _ _]
          tunnel: w2181 -> [_ w2217 w2280 _ _]
          tunnel: [w2193 _ _ _ _] -> w2179
          frame #0 {
            n1019 = Not(x=w2196) -> (.not. x?=w2203:bool)
            n1020 = for {
              tunnel: w2199 -> [w2210] mode=indexing
              tunnel: w2203 -> [w2207]
              shift-right: [w2205] -> w2201
              shift-left: dbl[] [] -> [w2206]
              n1021 = Unbundle(w2210) -> (w2209:dbl[], w2208:dbl[])
              n1022 = Select(t=w2209, s=w2207, f=w2208) -> (s? t:f=w2204:dbl[])
              n1023 = Build Array (concatenate)(w2206, w2204) -> (w2205:dbl[])
            }
            n1024 = Index Array(array=w2200, index=w2197) -> (element=w2195:dbl)
            n1025 = call "Numeric_bins.vi"("Values"=w2201, "Tolerance"=w2195) -> ("Bin Centres"=w2198:dbl[], "Bin Index"=w2194:i32[])  [unwired: 1 out]
          }
          frame #1 {
            n1026 = Array Size(array=w2215) -> (size(s)=w2214:i32)
            n1027 = global read "Results_plotter_Global.vi" "Plot Index values"() -> (w2212:dbl[][])
            n1028 = Index Array(array=w2212, index (row)=2) -> (element=w2211:dbl[])  [unwired: 1 in]
            n1029 = for {
              N: w2214 -> [_]
              tunnel: w2221 -> [w2231]
              tunnel: w2220 -> [w2230]
              tunnel: w2219 -> [w2229]
              tunnel: [w2222] -> w2218 mode=indexing
              tunnel: w2217 -> [w2228]
              tunnel: w2216 -> [w2226]
              tunnel: w2211 -> [w2225]
              i -> [w2227]
              n1030 = stacked-sequence {
                seq-local: [w2235 _] -> [_ w2254]
                tunnel: w2231 -> [_ w2255]
                tunnel: w2230 -> [_ w2253]
                tunnel: w2229 -> [_ w2252]
                tunnel: w2228 -> [_ w2251]
                tunnel: w2227 -> [w2234 _]
                tunnel: w2226 -> [w2233 _]
                tunnel: w2225 -> [w2232 _]
                tunnel: [_ w2249] -> w2224
                tunnel: [_ w2248] -> w2223
                frame #0 {
                  n1031 = for {
                    shift-right: [w2241] -> w2235
                    shift-left: i32[] [] -> [w2242]
                    tunnel: w2234 -> [w2240]
                    tunnel: w2233 -> [w2239] mode=indexing
                    tunnel: w2232 -> [w2237] mode=indexing
                    n1032 = Equal?(x=w2239, y=w2240) -> (x = y?=w2238:bool)
                    n1033 = case shown="False" w2238 {
                      tunnel: w2242 -> [w2243 w2246]
                      tunnel: [w2243 w2247] -> w2241
                      tunnel: w2237 -> [_ w2244]
                      frame False {
                      }
                      frame True {
                        n1034 = To Long Integer(number=w2244) -> (32bit integer=w2245:i32)
                        n1035 = Build Array (concatenate)(w2246, w2245) -> (w2247:i32[])
                      }
                    }
                  }
                }
                frame #1 {
                  n1036 = for {
                    tunnel: w2255 -> [w2269]
                    tunnel: w2254 -> [w2268]
                    tunnel: w2253 -> [w2266] mode=indexing
                    tunnel: w2252 -> [w2265] mode=indexing
                    tunnel: [w2264] -> w2249 mode=indexing
                    tunnel: w2251 -> [w2261] mode=indexing
                    shift-right: [w2256] -> w2248
                    shift-left: string[] [] -> [w2257]
                    i -> [w2263]
                    n1037 = for {
                      tunnel: w2269 -> [w2277]
                      tunnel: w2268 -> [w2276] mode=indexing
                      tunnel: [w2275] -> w2267 mode=indexing
                      tunnel: w2263 -> [w2274]
                      n1038 = Index Array(array=w2277, index (row)=w2276, index (col)=w2274) -> (element=w2275:string)
                    }
                    n1039 = Equal?(x="TRUE", y=w2261) -> (x = y?=w2260:bool)
                    n1040 = Not(x=w2260) -> (.not. x?=w2259:bool)
                    n1041 = call "Value_Occurence_Analysis.vi"("Average Numeric Values?"=w2259, "Tolerance"=w2265, "Precision (3)"=w2266, "String Array"=w2267) -> ("St Dev"=w2258:string, "Output String"=w2264:string)  [unwired: 1 out]
                    n1042 = case shown="False" w2259 {
                      tunnel: w2258 -> [_ w2273]
                      tunnel: w2257 -> [w2270 w2272]
                      tunnel: [w2270 w2271] -> w2256
                      frame False {
                      }
                      frame True {
                        n1043 = Build Array (concatenate)(w2272, w2273) -> (w2271:string[])
                      }
                    }
                  }
                }
              }
              n1044 = Build Array (concatenate)(w2224, w2223) -> (w2222:string[])
            }
          }
          frame #2 {
            n1045 = for {
              tunnel: w2280 -> [w2285] mode=indexing
              shift-right: [w2281] -> w2278
              shift-left: w2279 -> [w2282]
              tunnel: w2279 -> [w2283] mode=indexing
              n1046 = Equal?(x="TRUE", y=w2285) -> (x = y?=w2284:bool)
              n1047 = case shown="False" w2284 {
                tunnel: w2283 -> [w2291 _]
                tunnel: w2282 -> [w2288 w2292]
                tunnel: [w2287 w2292] -> w2281
                frame False {
                  n1048 = Concatenate Strings(w2291, "St Dev") -> (w2289:string)
                  n1049 = Build Array (concatenate)(w2288, w2289) -> (w2287:string[])
                }
                frame True {
                }
              }
            }
          }
          frame #3 {
            w2297 = FALSE  # Save Plotted rows only?
            w2299 = TRUE  # Simple Save?
            n1050 = local read "Output Filename"() -> (w2295:path)
            n1051 = local read "Header"() -> (w2296:string)
            n1052 = local read "Template"() -> (w2298:path)
            n1053 = call "Write_output_file.vi"("Output filename"=w2295, "Header"=w2296, "Template Filename"=w2298, "Channel Names"=w2294, "Data"=w2300, "Simple Save?"=w2299, "Save Plotted rows only?"=w2297, "Summarise mode"=T8."No data summary") -> ("Output filename Out"=w2301:path)  [unwired: 4 in, 3 out]
            n1054 = local write "Output Filename"(w2301) -> ()
          }
          frame #4 {
            n1055 = local write "Save Averaged rows"(FALSE ("Save Plot data")) -> ()
          }
        }
      }
      frame "Save Surface Fit data" {
        n1056 = local read "Transpose"() -> (w2307:bool)
        n1057 = local read "Tolerances"() -> (w2314:dbl[])
        n1058 = local read "Absisca"() -> (w2313:u16)
        n1059 = global read "Results_plotter_Global.vi" "Precision"() -> (w2310:string[])
        n1060 = stacked-sequence {
          seq-local: [w2321 _ _ _ _ _] -> [_ w2340 _ _ _ _]
          seq-local: [_ w2337 _ _ _ _] -> [_ _ _ _ w2424 _]
          seq-local: [_ _ w2363 _ _ _] -> [_ _ _ _ w2443 _]
          seq-local: [w2322 _ _ _ _ _] -> [_ _ w2364 _ _ _]
          seq-local: [_ _ w2359 _ _ _] -> [_ _ _ _ w2427 _]
          seq-local: [_ _ w2358 _ _ _] -> [_ _ _ w2394 _ _]
          seq-local: [_ _ _ w2389 _ _] -> [_ _ _ _ w2425 _]
          tunnel: [_ _ _ _ _ TRUE] -> w2318
          tunnel: [_ _ _ _ _ "Create Selectors"] -> w2317
          tunnel: w2315 -> [_ _ _ _ _ w2449]
          tunnel: w2316 -> [_ w2325 _ _ _ w2450]
          tunnel: w2314 -> [_ w2351 _ _ _ _]
          tunnel: w2313 -> [_ w2352 _ _ _ _]
          tunnel: [_ _ w2369 _ _ _] -> w2312
          tunnel: w2311 -> [_ w2328 w2369 _ _ _]
          tunnel: w2310 -> [_ _ w2365 _ _ _]
          tunnel: [_ _ _ _ _ w2450] -> w2309
          tunnel: [_ _ _ _ _ w2449] -> w2308
          tunnel: w2307 -> [_ _ _ w2388 _ _]
          frame #0 {
            n1061 = global read "Results_plotter_Global.vi" "Raw Interpolation"() -> (w2319:dbl[][])
            n1062 = global read "Results_plotter_Global.vi" "X Values"() -> (w2321:dbl[])
            n1063 = global read "Results_plotter_Global.vi" "Y Values"() -> (w2320:dbl[])
            n1064 = Insert Into Array(array=w2319, index (col)=0 ("disabled index (col)"), new element=w2320) -> (w2322:dbl[][])  [unwired: 1 in]
          }
          frame #1 {
            n1065 = global read "Results_plotter_Global.vi" "Y Axis Name"() -> (w2327:string)
            n1066 = Search 1D Array(1D array=w2328, element=w2327) -> (index of element=w2326:i32)  [unwired: 1 out]
            n1067 = Index Array(array=w2325, index=w2326) -> (element=w2324:string)
            n1068 = Match Pattern(string=w2324, regular expression=":") -> (before substring=w2354:string, after substring=w2353:string)  [unwired: 3 out]
            n1069 = Index Array(array=w2351, index=w2352) -> (element=w2342:dbl)
            n1070 = Concatenate Strings(w2354, " ", w2353, " =:" ("regular expression")) -> (w2336:string)
            n1071 = Greater?(x=w2342, y=0.9) -> (0:w2349:bool)
            n1072 = Greater?(x=w2342, y=0.09) -> (0:w2344:bool)
            n1073 = call <vilib>:"Trim Whitespace.vi"("string"=w2336) -> ("trimmed string"=w2335:string)  [unwired: 1 in]
            n1074 = Select(t=i16 0 ("precision (6)"), s=w2349, f=i16 2 ("precision (6)")) -> (s? t:f=w2345:i16)
            n1075 = Select(t=w2345, s=w2344, f=i16 3) -> (s? t:f=w2341:i16)
            n1076 = Number To Fractional String(number=w2340, precision (6)=w2341) -> (F-format string=w2339:string[])  [unwired: 2 out]
            n1077 = for {
              tunnel: w2335 -> [w2357]
              tunnel: w2339 -> [w2355] mode=indexing
              tunnel: [w2356] -> w2330 mode=indexing
              n1078 = Concatenate Strings(w2357, w2355) -> (w2356:string)
            }
            n1079 = Build Array (concatenate)("Channel:Values:Plotted" ("Input Element"), "Axis:Name:" ("Input Element"), "Axis:Values:" ("Input Element"), w2330) -> (w2337:string[])
          }
          frame #2 {
            n1080 = global read "Results_plotter_Global.vi" "X Axis Name"() -> (w2362:string)
            n1081 = Concatenate Strings(w2362, " =" ("string")) -> (w2360:string)
            n1082 = local read "Multi Ordinate"() -> (w2368:i32[])
            n1083 = Index Array(array=w2368, index=0 ("Index")) -> (element=w2366:i32)
            n1084 = Index Array(array=w2365, index=w2366) -> (element=w2358:string)
            n1085 = Index Array(array=w2369, index=w2366) -> (element=w2359:string)
            n1086 = for {
              tunnel: w2359 -> [w2371]
              tunnel: [w2374] -> w2363 mode=indexing
              tunnel: w2358 -> [w2373]
              tunnel: w2364 -> [w2372] mode=indexing
              tunnel: w2360 -> [w2370]
              n1087 = for {
                tunnel: w2372 -> [w2377] mode=indexing
                tunnel: [w2376] -> w2375 mode=indexing
                tunnel: w2373 -> [w2379]
                n1088 = Not A Number/Path/Refnum?(number/path/refnum=w2377) -> (NaN/Path/Refnum?=w2378:bool)
                n1089 = case shown="False" w2378 {
                  tunnel: w2379 -> [w2382 _]
                  tunnel: w2377 -> [w2381 _]
                  tunnel: [w2380 ""] -> w2376
                  frame False {
                    n1090 = call "Number_2_string.vi"("precision"=w2382, "number"=w2381) -> ("String"=w2380:string)
                  }
                  frame True {
                  }
                }
              }
              n1091 = Build Array (concatenate)(w2371, w2370, w2375) -> (w2374:string[])
            }
          }
          frame #3 {
            w2393 = "\t"
            n1092 = global read "Results_plotter_Global.vi" "Intensity Plot data in rows"() -> (w2395:dbl[][])
            n1093 = global read "Results_plotter_Global.vi" "Value plotted Name"() -> (w2392:string)
            n1094 = global read "Results_plotter_Global.vi" "X Axis Name"() -> (w2386:string)
            n1095 = global read "Results_plotter_Global.vi" "Y Axis Name"() -> (w2385:string)
            n1096 = case shown="False" w2388 {
              tunnel: [w2396 w2399] -> w2387
              tunnel: w2386 -> [w2397 w2399]
              tunnel: w2385 -> [w2396 w2398]
              tunnel: [w2397 w2398] -> w2384
              frame False {
              }
              frame True {
              }
            }
            n1097 = Concatenate Strings(w2387, w2393, w2384, w2393, w2392, "\r") -> (w2390:string)
            n1098 = for {
              tunnel: w2395 -> [w2405] mode=indexing
              tunnel: w2394 -> [w2410]
              shift-right: [w2404] -> w2389
              shift-left: w2390 -> [w2409]
              n1099 = Index Array(array=w2405, index=0) -> (element=w2401:dbl)
              n1100 = Index Array(array=w2405, index=1) -> (element=w2400:dbl)
              n1101 = Index Array(array=w2405, index=2) -> (element=w2403:dbl)
              n1102 = Not A Number/Path/Refnum?(number/path/refnum=w2403) -> (NaN/Path/Refnum?=w2402:bool)
              n1103 = case shown="False" w2402 {
                tunnel: w2410 -> [w2421 _]
                tunnel: w2409 -> [w2420 w2422]
                tunnel: w2403 -> [w2419 _]
                tunnel: [w2418 w2422] -> w2404
                tunnel: w2401 -> [w2417 _]
                tunnel: w2400 -> [w2416 _]
                frame False {
                  w2412 = "\t"
                  n1104 = call "Number_2_string.vi"("number"=w2417) -> ("String"=w2415:string)  [unwired: 1 in]
                  n1105 = call "Number_2_string.vi"("number"=w2416) -> ("String"=w2414:string)  [unwired: 1 in]
                  n1106 = call "Number_2_string.vi"("precision"=w2421, "number"=w2419) -> ("String"=w2413:string)
                  n1107 = Concatenate Strings(w2420, w2415, w2412, w2414, w2412, w2413, "\r") -> (w2418:string)
                }
                frame True {
                }
              }
            }
          }
          frame #4 {
            w2439 = TRUE  # append to file? (new file:F)
            n1108 = global read "Results_plotter_Global.vi" "Surface Integral"() -> (w2438:dbl)
            n1109 = global read "Results_plotter_Global.vi" "Surface Area"() -> (w2437:dbl)
            n1110 = Initialize Array("", 10 ("Dimension Size")) -> (w2448:string[])
            n1111 = Divide(x=w2438, y=w2437) -> (x/y=w2436:dbl)
            n1112 = call "Asterisk_header.vi"("Channel names"=w2448) -> ("Header string"=w2426:string)
            n1113 = call "Value_to_string.vi"("Value"=w2438, "Label for value"="Surface Integral") -> ("Output string"=w2433:string)  [unwired: 1 in]
            n1114 = call "Value_to_string.vi"("Value"=w2437, "Label for value"="Surface Area") -> ("Output string"=w2434:string)  [unwired: 1 in]
            n1115 = call "Value_to_string.vi"("Value"=w2436, "Label for value"="Surface Average") -> ("Output string"=w2432:string)  [unwired: 1 in]
            n1116 = Concatenate Strings(w2434, w2433, w2432) -> (w2429:string)
            n1117 = call "Ch_names_to_rows.vi"("Channel Names"=w2424) -> ("3 Row names"=w2423:string[][])
            n1118 = local read "Output Filename"() -> (w2440:path)
            n1119 = Build Array (concatenate)(w2423, w2443) -> (w2441:string[][])
            n1120 = Array To Spreadsheet String(array=w2441, 3:"%s" ("format string")) -> (spreadsheet string=w2428:string)  [unwired: 1 out]
            n1121 = Format Into String(format string="\n%s\n\n%s\n%s\n\n\nInterpolated Surface of %s\n%s\n%s\n%s\n\n\n%s", w2426, w2425, w2426, w2427, w2426, w2428, w2426, w2429) -> (resulting string=w2431:string)  [unwired: 2 in, 1 out]
            n1122 = call "Write_Characters_To_File.vi"("file path (dialog if empty)"=w2440, "character string"=w2431, "append to file? (new file:F)"=w2439) -> ()  [unwired: 2 in, 4 out]
          }
          frame #5 {
            n1123 = local write "Save Surface Fit"(FALSE ("Save Plot data")) -> ()
          }
        }
      }
      frame "Save Data in Rows" {
        w2465 = TRUE  # Show panel ?
        n1124 = local read "Output Filename"() -> (w2462:path)
        n1125 = local write "Save Data in Rows"(FALSE ("Save All data")) -> ()
        n1126 = call "Output_file_Panel.vi"("Show panel ?"=w2465, "Channel Names"=w2460, "Header"="Header", "Output filename"=w2462) -> ("Save Full Res Data?"=w2457:bool, "Desired Columns"=w2466:i32[], "Header Out"=w2464:string, "Output filename Out"=w2468:path, "Channels to Tabulate in header Out"=w2454:i32[], "Save Plotted rows only?"=w2455:bool, "Summarise mode"=w2463:T8, "Grouping info"=w2456:T13[])
        "Plotted rows only?" <- w2455
        n1127 = case shown="False" w2457 {
          tunnel: w2468 -> [w2484 w2486]
          tunnel: w2466 -> [w2483 _]
          tunnel: w2464 -> [w2482 _]
          tunnel: w2455 -> [w2481 _]
          tunnel: w2463 -> [w2480 _]
          tunnel: w2461 -> [w2479 _]
          tunnel: w2460 -> [w2478 _]
          tunnel: [w2477 w2486] -> w2459
          tunnel: ["Create Selectors" "Is Filename Empty?"] -> w2458
          tunnel: w2456 -> [w2473 _]
          tunnel: w2454 -> [w2472 _]
          frame False {
            w2475 = FALSE  # Simple Save?
            n1128 = local read "Template"() -> (w2476:path)
            n1129 = call "Write_output_file.vi"("Output filename"=w2484, "Header"=w2482, "Template Filename"=w2476, "Channel Names"=w2478, "Data"=w2479, "Desired Columns"=w2483, "Simple Save?"=w2475, "Save Plotted rows only?"=w2481, "Summarise mode"=w2480, "Grouping info"=w2473, "Channels to Tabulate in header"=w2472) -> ("Output filename Out"=w2477:path)  [unwired: 1 in, 3 out]
          }
          frame True {
            "Mode" <- Plotter_Mode."Save file" ("Mode")
          }
        }
        n1130 = local write "Output Filename"(w2459) -> ()
      }
      frame "Is Filename Empty?" {
        n1131 = call "File Dialog"("start path"="Full_Res_Results_Folder", "prompt"="Please select a new or existing folder to save the results files in") -> ("selected path"=w2490:path, "cancelled"=w2488:bool)  [unwired: 5 in, 7 out]
        n1132 = local write "Full_Res_Results_Folder"(w2490) -> ()
        n1133 = case shown="False" w2488 {
          tunnel: ["Full Res file manipulator" ("f") "Create Selectors" ("t")] -> w2492
          frame False {
          }
          frame True {
          }
        }
      }
      frame "Check for overwrite or append" {
        n1134 = local read "Output Filename"() -> (w2506:path)
        n1135 = Format Into String(format string="Do you want to append to the result file\n\"%s\"" ("message"), w2506) -> (resulting string=w2501:string)  [unwired: 2 in, 1 out]
        n1136 = call <vilib>:"Three Button Dialog.vi"("Window Title (\"\")"="Output File Dialog" ("Window Title (\"\")"), "Right Button Text (\"Cancel\")"="Cancel" ("Button 3 Name"), "Center Button Text (\"No\")"="Overwrite" ("F button name (\"Cancel\")"), "Left Button Text (\"Yes\")"="Append" ("T button name (\"OK\")"), "message"=w2501) -> ("Which Button?"=w2500:T10)  [unwired: 6 out]
        n1137 = case shown="\"Center Button\"" w2500 {
          tunnel: w2506 -> [_ w2513 _]
          tunnel: ["Full Res file manipulator" "Full Res file manipulator" "Create Selectors" ("t")] -> w2499
          frame "Left Button" {
          }
          frame "Center Button" {
            n1138 = call "Delete_with_Check.vi"("FilePath"=w2513) -> ()  [unwired: 1 out]
          }
          frame "Right Button", Default {
          }
        }
      }
      frame "Create Plot summary" {
        w2528 = TRUE  # Summarise All
        n1139 = global read "Results_plotter_Global.vi" "Plot Index values"() -> (w2531:dbl[][])
        n1140 = local read "Intensity Plot?"() -> (w2527:bool)
        n1141 = global read "Results_plotter_Global.vi" "Row Reference"() -> (w2523:i32[][])
        n1142 = Index Array(array=w2523, index (col)=0 ("disabled index (col)")) -> (element=w2522:i32[])  [unwired: 1 in]
        n1143 = Index Array(array=w2531, index (row)=2) -> (element=w2533:dbl[])  [unwired: 1 in]
        n1144 = Select(t="Save Intensity plot as jpg", s=w2527, f="Create summary per series") -> (s? t:f=w2518:string)
        n1145 = To Long Integer(number=w2533) -> (32bit integer=w2530:i32[])
        n1146 = for {
          tunnel: w2538 -> [w2551]
          tunnel: [w2550] -> w2529 mode=indexing
          tunnel: w2530 -> [w2548] mode=indexing
          tunnel: w2522 -> [w2549]
          shift-right: [w2545] -> w2520
          shift-left: i32[] [] -> [w2546]
          n1147 = Index Array(array=w2549, index=w2548) -> (element=w2544:i32)
          n1148 = Search 1D Array(1D array=w2546, element=w2544) -> (index of element=w2547:i32)  [unwired: 1 out]
          n1149 = Index Array(array=w2551, index (row)=w2548) -> (element=w2550:string[])  [unwired: 1 in]
          n1150 = case shown="0, Default" w2547 {
            tunnel: w2544 -> [_ w2555]
            tunnel: w2546 -> [w2552 w2554]
            tunnel: [w2552 w2553] -> w2545
            frame 0, Default {
            }
            frame -1 {
              n1151 = Build Array (concatenate)(w2554, w2555) -> (w2553:i32[])
            }
          }
        }
        n1152 = local read "Result files to read"() -> (w2519:path[])
        n1153 = for {
          tunnel: w2520 -> [w2543] mode=indexing
          tunnel: w2519 -> [w2542]
          tunnel: [w2539] -> w2517 mode=indexing
          n1154 = Index Array(array=w2542, index=w2543) -> (element=w2541:path)
          n1155 = Strip Path(path=w2541) -> (name=w2540:string)  [unwired: 1 out]
          n1156 = call "Add_filename_suffix.vi"("Filename"=w2540) -> ("Base name"=w2539:string)  [unwired: 1 in, 3 out]
        }
        n1157 = call "Value_Occurence_Analysis.vi"("String Array"=w2517) -> ("Output String"=w2516:string)  [unwired: 3 in, 2 out]
        n1158 = global write "Results_plotter_Global.vi" "Current Data Filenames"(w2516) -> ()
        n1159 = call "Summarise.vi"("Channel Names"=w2534, "Data"=w2529, "Summarise All"=w2528) -> ("Summary"=w2536:string[][])  [unwired: 2 in]
        n1160 = global write "Results_plotter_Global.vi" "Plot Summary"(w2536) -> ()
      }
      frame "Create summary per series" {
        n1161 = global read "Results_plotter_Global.vi" "Plot Summary"() -> (w2557:string[][])
        n1162 = local read "Plotted Series"() -> (w2559:bool[][])
        n1163 = for {
          tunnel: w2559 -> [w2576] mode=indexing
          tunnel: i32[] [] -> [w2575]
          tunnel: w2564 -> [w2573]
          tunnel: w2561 -> [w2571]
          shift-right: [w2565] -> w2556
          shift-left: w2557 -> [w2567]
          w2570 = TRUE  # Summarise All
          n1164 = for {
            shift-right: [w2584] -> w2574
            shift-left: w2575 -> [w2585]
            tunnel: w2576 -> [w2583] mode=indexing
            i -> [w2586]
            n1165 = case shown="True" w2583 {
              tunnel: w2586 -> [_ w2590]
              tunnel: w2585 -> [w2587 w2589]
              tunnel: [w2587 w2588] -> w2584
              frame False {
              }
              frame True {
                n1166 = Build Array (concatenate)(w2589, w2590) -> (w2588:i32[])
              }
            }
          }
          n1167 = for {
            tunnel: w2574 -> [w2582] mode=indexing
            tunnel: w2573 -> [w2581]
            tunnel: [w2580] -> w2572 mode=indexing
            n1168 = Index Array(array=w2581, index (row)=w2582) -> (element=w2580:string[])  [unwired: 1 in]
          }
          n1169 = call "Summarise.vi"("Channel Names"=w2571, "Data"=w2572, "Summarise All"=w2570) -> ("Summary"=w2568:string[][])  [unwired: 2 in]
          n1170 = Index Array(array=w2568, index (col)=2 ("disabled index (col)")) -> (element=w2566:string[])  [unwired: 1 in]
          n1171 = for {
            tunnel: w2567 -> [w2579] mode=indexing
            tunnel: w2566 -> [w2578] mode=indexing
            tunnel: [w2577] -> w2565 mode=indexing
            n1172 = Build Array (concatenate)(w2579, w2578) -> (w2577:string[])
          }
        }
        n1173 = global write "Results_plotter_Global.vi" "Plot Summary"(w2556) -> ()
      }
      frame "Save Intensity plot as jpg" {
        n1174 = local read "Job Directory"() -> (w2597:path)
        n1175 = global read "Constants_global.vi" "EnFlo SW Folder"() -> (w2599:path)
        n1176 = Build Path(base path=w2599, name or relative path=path "Anemometry/Anemometry Sub Vis/Data_plotting_vis/Intensity Plot Vis") -> (appended path=w2593:path)
        n1177 = call "Remote_call_prep.vi"("Vi Name in"="Create picture Vi Name", "Job Directory In"=w2597, "VI Directory"=w2593) -> ("Vi Name out"=w2595:string, "Job Directory out"=w2592:path, "cancelled"=w2591:bool)
        n1178 = local write "Create picture Vi Name"(w2595) -> ()
        n1179 = local write "Job Directory"(w2592) -> ()
        n1180 = Build Path(base path=w2593, name or relative path=w2595) -> (appended path=w2594:path)
        n1181 = case shown="False" w2591 {
          tunnel: w2594 -> [w2608 _]
          tunnel: w2592 -> [w2607 _]
          frame False {
            n1182 = Open VI Reference(type specifier VI Refnum (for type only)="type specifier VI Refnum (for type only)", vi path=w2608) -> (vi reference=w2613:refnum<vi>, error out=w2612:errorcluster)  [unwired: 2 in, 2 out]
            n1183 = property class="VI Interface Type 0"(reference=w2613, error in=w2612, "Front Panel Window:Open"=TRUE) -> (reference out=w2609:refnum<vi>, error out=w2610:errorcluster)
            n1184 = local read "Intensity Graph"() -> (w2616:dbl[][])
            n1185 = local read "No of Contours"() -> (w2606:i32)
            n1186 = call-by-ref "?"(reference=w2609, error in=w2610, "No of Contours"=w2606, "Job Directory"=w2607, "Intensity Graph"=w2616) -> (reference out=w2615:refnum<vi>, error out=w2614:errorcluster)  [unwired: 3 in]
            n1187 = Close Reference(reference=w2615, error in (no error)=w2614) -> ()  [unwired: 1 out]
          }
          frame True {
          }
        }
        n1188 = local write "Save Plot as jpg"(FALSE ("Save All data")) -> ()
      }
      frame "Run Calculation Routine" {
        n1189 = stacked-sequence {
          seq-local: [w2625 _ _] -> [_ w2635 _]
          seq-local: [w2624 _ _] -> [_ w2636 _]
          tunnel: [_ w2634 _] -> w2619
          tunnel: w2618 -> [_ _ _]
          frame #0 {
            n1190 = global read "Constants_global.vi" "EnFlo SW Folder"() -> (w2631:path)
            n1191 = Build Path(base path=w2631, name or relative path=path "Anemometry/Anemometry Sub Vis/Data_plotting_vis/Calculation Vis") -> (appended path=w2628:path)
            n1192 = local read "Job Directory"() -> (w2627:path)
            n1193 = call "Remote_call_prep.vi"("Vi Name in"="Calculate Routine", "Job Directory In"=w2627, "VI Directory"=w2628) -> ("Vi Name out"=w2629:string, "Job Directory out"=w2626:path, "cancelled"=w2625:bool)
            n1194 = local write "Calculate Routine"(w2629) -> ()
            n1195 = local write "Job Directory"(w2626) -> ()
            n1196 = Build Path(base path=w2628, name or relative path=w2629) -> (appended path=w2624:path)
          }
          frame #1 {
            n1197 = case shown="False" w2635 {
              tunnel: w2636 -> [w2644 _]
              tunnel: [w2640 w2657] -> w2634
              tunnel: "What to do next?" -> [w2639 w2657]
              frame False {
                n1198 = Open VI Reference(type specifier VI Refnum (for type only)="VI Refnum Calculation", vi path=w2644) -> (vi reference=w2650:refnum<vi>, error out=w2649:errorcluster)  [unwired: 1 in, 3 out]
                n1199 = property class="VI Interface Type 1"(reference=w2650, error in=w2649, "Front Panel Window:Open"=TRUE) -> (reference out=w2646:refnum<vi>, error out=w2647:errorcluster)
                n1200 = call-by-ref "?"(reference=w2646, error in=w2647) -> (reference out=w2652:refnum<vi>, error out=w2651:errorcluster, "New Values In"=w2637:string[][], "New Chs In"=w2645:string[])  [unwired: 2 in]
                n1201 = for {
                  tunnel: w2645 -> [w2655] mode=indexing
                  tunnel: [w2654] -> w2638 mode=indexing
                  n1202 = call "Check_Ch_Name_colons.vi"("No of Colons"=2, "Ch Name in"=w2655) -> ("Ch Name out"=w2654:string)
                }
                n1203 = Empty String/Path?(string/path=w2638) -> (empty?=w2642:bool[])
                n1204 = Or Array Elements(Boolean array=w2642) -> (logical OR=w2641:bool)
                n1205 = Close Reference(reference=w2652, error in (no error)=w2651) -> ()  [unwired: 1 out]
                n1206 = Select(t=w2639, s=w2641, f="Input calculated values") -> (s? t:f=w2640:string)
                n1207 = global write "Results_plotter_Global.vi" "New Values In"(w2637) -> ()
                n1208 = global write "Results_plotter_Global.vi" "New Chs In"(w2638) -> ()
              }
              frame True {
              }
            }
          }
          frame #2 {
            w2660 = FALSE ("Raw DF in Orig Pos?")
            n1209 = local write "Edit Raw Data Header Info"(w2660) -> ()
            n1210 = local write "Calculate new metadata"(FALSE ("Save All data")) -> ()
            n1211 = local write "Plotted rows only?"(TRUE ("Plotted rows only?")) -> ()
            n1212 = local write "Raw DF in Orig Pos?"(w2660) -> ()
            n1213 = local write "Edit Raw DF?"(w2660) -> ()
            n1214 = local write "Mode"(Plotter_Mode."Edit values per row" ("Mode")) -> ()
          }
        }
      }
      frame "Input calculated values" {
        n1215 = local read "Result files to read"() -> (w2666:path[])
        n1216 = local read "Raw DF in Orig Pos?"() -> (w2663:bool)
        n1217 = stacked-sequence {
          seq-local: [w2670 _ _ _] -> [_ w2683 w2695 _]
          seq-local: [_ w2680 _ _] -> [_ _ w2696 _]
          tunnel: [_ _ _ w2748] -> w2668
          tunnel: w2666 -> [_ _ w2697 _]
          tunnel: w2665 -> [_ _ w2694 _]
          tunnel: w2664 -> [_ _ w2693 _]
          tunnel: w2663 -> [_ _ w2692 _]
          tunnel: w2662 -> [_ _ _ w2745]
          frame #0 {
            n1218 = global read "Results_plotter_Global.vi" "Plot Index values"() -> (w2673:dbl[][])
            n1219 = global read "Results_plotter_Global.vi" "Row Reference"() -> (w2674:i32[][])
            n1220 = Index Array(array=w2673, index (row)=2) -> (element=w2671:dbl[])  [unwired: 1 in]
            n1221 = for {
              tunnel: w2674 -> [w2678]
              tunnel: w2671 -> [w2677] mode=indexing
              tunnel: [w2676] -> w2670 mode=indexing
              n1222 = Index Array(array=w2678, index (row)=w2677) -> (element=w2676:i32[])  [unwired: 1 in]
            }
            n1223 = local write "Delete Plotted data from file"(FALSE ("Save All data")) -> ()
          }
          frame #1 {
            n1224 = Index Array(array=w2683, index (col)=0 ("disabled index (col)")) -> (element=w2679:i32[])  [unwired: 1 in]
            n1225 = for {
              shift-right: [w2685] -> w2680
              shift-left: i32[] [] -> [w2686]
              tunnel: w2679 -> [w2684] mode=indexing
              n1226 = Search 1D Array(1D array=w2686, element=w2684) -> (index of element=w2687:i32)  [unwired: 1 out]
              n1227 = case shown="-1" w2687 {
                tunnel: w2686 -> [w2688 w2691]
                tunnel: [w2688 w2690] -> w2685
                tunnel: w2684 -> [_ w2689]
                frame 0, Default {
                }
                frame -1 {
                  n1228 = Build Array (concatenate)(w2691, w2689) -> (w2690:i32[])
                }
              }
            }
          }
          frame #2 {
            n1229 = for {
              tunnel: w2697 -> [w2704]
              tunnel: w2696 -> [w2701] mode=indexing
              tunnel: w2695 -> [w2702]
              tunnel: w2694 -> [w2700]
              tunnel: w2693 -> [w2699]
              tunnel: w2692 -> [w2698]
              # "New Values"
              # "Row in file"
              n1230 = Index Array(array=w2704, index=w2701) -> (element=w2703:path)
              n1231 = stacked-sequence {
                seq-local: [w2709 _] -> [_ w2743]
                seq-local: [w2707 _] -> [_ w2738]
                tunnel: w2703 -> [_ w2744]
                tunnel: w2702 -> [w2711 _]
                tunnel: w2701 -> [w2710 _]
                tunnel: w2700 -> [_ _]
                tunnel: w2699 -> [_ _]
                tunnel: w2698 -> [_ w2742]
                frame #0 {
                  n1232 = global read "Results_plotter_Global.vi" "New Values In"() -> (w2705:string[][])
                  n1233 = for {
                    tunnel: w2710 -> [w2722]
                    tunnel: w2711 -> [w2718] mode=indexing
                    shift-right: [w2716] -> w2709
                    shift-left: i32[] [] -> [w2717]
                    shift-right: [w2715] -> w2707
                    shift-left: string[][] [] -> [w2714]
                    tunnel: w2705 -> [w2713]
                    i -> [w2712]
                    n1234 = Index Array(array=w2718, index=0) -> (element=w2720:i32)
                    n1235 = Equal?(x=w2720, y=w2722) -> (x = y?=w2719:bool)
                    n1236 = case shown="True" w2719 {
                      tunnel: w2718 -> [_ w2728]
                      tunnel: w2717 -> [w2724 w2733]
                      tunnel: [w2724 w2731] -> w2716
                      tunnel: w2714 -> [w2723 w2729]
                      tunnel: [w2723 w2730] -> w2715
                      tunnel: w2713 -> [_ w2726]
                      tunnel: w2712 -> [_ w2725]
                      frame False {
                      }
                      frame True {
                        n1237 = Index Array(array=w2726, index (row)=w2725) -> (element=w2727:string[])  [unwired: 1 in]
                        n1238 = Index Array(array=w2728, index=1) -> (element=w2732:i32)
                        n1239 = Build Array (concatenate)(w2733, w2732) -> (w2731:i32[])
                        n1240 = Build Array (concatenate)(w2729, w2727) -> (w2730:string[][])
                      }
                    }
                  }
                }
                frame #1 {
                  w2737 = FALSE  # Edit all Rows?
                  w2739 = FALSE  # Edit Raw DF?
                  w2740 = FALSE  # Edit Raw Data Header Info
                  w2741 = FALSE  # Value  Constant?
                  n1241 = global read "Results_plotter_Global.vi" "New Chs In"() -> (w2735:string[])
                  n1242 = local read "Job Directory"() -> (w2736:path)
                  n1243 = call "Add_Update_Values.vi"("Filename"=w2744, "Value  Constant?"=w2741, "Edit Raw data files?"=w2739, "New Chs In"=w2735, "Edit Raw Data Header Info"=w2740, "New Values In"=w2738, "Selected Rows"=w2743, "Edit all Rows?"=w2737, "Raw DF in Orig Pos?"=w2742, "Job Directory"=w2736) -> ()  [unwired: 1 in, 5 out]
                }
              }
            }
          }
          frame #3 {
            n1244 = local read "No Of Rows"() -> (w2747:i32)
            n1245 = Less?(x=w2747, y=w2745) -> (x < y?=w2746:bool)
            n1246 = Current VI's Path() -> (path=w2749:path)
            n1247 = case shown="True" w2746 {
              tunnel: ["Create Selectors" "Initialise" ("t")] -> w2748
              frame False {
              }
              frame True {
              }
            }
            n1248 = call "Bring_to_front.vi"("path"=w2749) -> ()
          }
        }
      }
      frame "Save XY plot as jpg" {
        n1249 = local read "Create picture Vi Name"() -> (w2756:string)
        n1250 = local read "Job Directory"() -> (w2759:path)
        n1251 = global read "Constants_global.vi" "EnFlo SW Folder"() -> (w2761:path)
        n1252 = Build Path(base path=w2761, name or relative path=path "Anemometry/Anemometry Sub Vis/Data_plotting_vis/XY Plot Vis") -> (appended path=w2757:path)
        n1253 = call "Remote_call_prep.vi"("Vi Name in"=w2756, "Job Directory In"=w2759, "VI Directory"=w2757) -> ("Vi Name out"=w2758:string, "Job Directory out"=w2754:path, "cancelled"=w2753:bool)
        n1254 = local write "Create picture Vi Name"(w2758) -> ()
        n1255 = local write "Job Directory"(w2754) -> ()
        n1256 = Build Path(base path=w2757, name or relative path=w2758) -> (appended path=w2755:path)
        n1257 = case shown="False" w2753 {
          tunnel: [w2774 FALSE ("Saved Automatically?")] -> w2764
          tunnel: [w2773 path "" ("Plot data file")] -> w2763
          tunnel: [w2772 "" ("Tex Info String")] -> w2762
          tunnel: w2755 -> [w2771 _]
          tunnel: w2754 -> [w2770 _]
          frame False {
            n1258 = Open VI Reference(type specifier VI Refnum (for type only)="type specifier VI Refnum (for type only) 2", vi path=w2771) -> (vi reference=w2781:refnum<vi>, error out=w2780:errorcluster)  [unwired: 1 in, 3 out]
            n1259 = property class="VI Interface Type 2"(reference=w2781, error in=w2780, "Front Panel Window:Open"=TRUE) -> (reference out=w2777:refnum<vi>, error out=w2778:errorcluster)
            n1260 = global read "Results_plotter_Global.vi" "XY Graph Cluster"() -> (w2775:cluster{dbl[], dbl[]}[])
            n1261 = call-by-ref "?"(reference=w2777, error in=w2778, "Plot Array"=w2775, "Template"=w2770) -> (reference out=w2783:refnum<vi>, error out=w2782:errorcluster, "Saved Automatically?"=w2774:bool, "Tex Info String"=w2772:string, "Plot data file"=w2773:path)
            n1262 = Close Reference(reference=w2783, error in (no error)=w2782) -> ()  [unwired: 1 out]
          }
          frame True {
          }
        }
        n1263 = local write "Save Plot as jpg"(FALSE ("Save All data")) -> ()
        n1264 = case shown="False" w2764 {
          tunnel: w2763 -> [_ w2795]
          tunnel: [w2787 "Save Plot Data"] -> w2752
          tunnel: w2762 -> [_ w2793]
          frame False {
            n1265 = global read "Results_plotter_Global.vi" "New Chs In"() -> (w2792:string[])
            n1266 = Array Size(array=w2792) -> (size(s)=w2791:i32)
            n1267 = Greater Than 0?(x=w2791) -> (x > 0?=w2790:bool)
            n1268 = Select(t="Input calculated values", s=w2790, f="Create Selectors") -> (s? t:f=w2787:string)
          }
          frame True {
            n1269 = local write "Output Filename"(w2795) -> ()
            n1270 = local write "Header"(w2793) -> ()
          }
        }
      }
      frame "Full Res file manipulator" {
        n1271 = local read "Result files to read"() -> (w2805:path[])
        n1272 = local read "Output Filename"() -> (w2803:path)
        n1273 = local read "Mode"() -> (w2804:T1)
        n1274 = local read "Raw DF in Orig Pos?"() -> (w2799:bool)
        n1275 = local read "Plotted rows only?"() -> (w2802:bool)
        n1276 = global read "Results_plotter_Global.vi" "New Values In"() -> (w2796:string[][])
        n1277 = global read "Results_plotter_Global.vi" "New Chs In"() -> (w2797:string[])
        n1278 = stacked-sequence {
          seq-local: [w2810 _ _ _ _] -> [_ w2837 w2872 _ _]
          seq-local: [_ w2834 _ _ _] -> [_ _ w2873 _ _]
          seq-local: [_ w2831 _ _ _] -> [_ _ w2864 _ _]
          seq-local: [_ _ w2862 _ _] -> [_ _ _ w3085 _]
          seq-local: [_ _ w2861 _ _] -> [_ _ _ w3084 _]
          seq-local: [_ _ w2856 _ _] -> [_ _ _ w3081 _]
          tunnel: [_ _ _ w3088 _] -> w2807
          tunnel: w2805 -> [_ _ w2874 _ _]
          tunnel: w2804 -> [_ w2830 w2871 w3086 _]
          tunnel: w2803 -> [_ _ w2870 _ _]
          tunnel: w2802 -> [w2809 _ w2869 _ _]
          tunnel: w2797 -> [_ _ w2868 _ _]
          tunnel: w2801 -> [_ _ w2867 w3082 _]
          tunnel: w2800 -> [_ _ w2866 w3083 _]
          tunnel: w2799 -> [_ _ w2865 _ _]
          tunnel: w2798 -> [_ _ _ w3087 _]
          tunnel: w2796 -> [_ _ w2858 _ _]
          frame #0 {
            n1279 = global read "Results_plotter_Global.vi" "Row Reference"() -> (w2811:i32[][])
            n1280 = case shown="True" w2809 {
              tunnel: w2811 -> [w2813 w2814]
              tunnel: [w2813 w2815] -> w2810
              frame False {
              }
              frame True {
                n1281 = local read "Plotted Series"() -> (w2817:bool[][])
                n1282 = for {
                  tunnel: w2817 -> [w2824]
                  shift-right: [w2818] -> w2815
                  shift-left: i32[][] [] -> [w2820]
                  tunnel: w2814 -> [w2819] mode=indexing
                  i -> [w2823]
                  n1283 = Index Array(array=w2824, index (col)=w2823) -> (element=w2822:bool[])  [unwired: 1 in]
                  n1284 = Or Array Elements(Boolean array=w2822) -> (logical OR=w2821:bool)
                  n1285 = case shown="True" w2821 {
                    tunnel: w2820 -> [w2825 w2828]
                    tunnel: w2819 -> [_ w2827]
                    tunnel: [w2825 w2826] -> w2818
                    frame False {
                    }
                    frame True {
                      n1286 = Build Array (concatenate)(w2828, w2827) -> (w2826:i32[][])
                    }
                  }
                }
              }
            }
            n1287 = local write "Delete Plotted data from file"(FALSE ("Save All data")) -> ()
          }
          frame #1 {
            n1288 = local read "Job Directory"() -> (w2829:path)
            n1289 = case shown="\"Post Process Plotted Rows\"" w2830 {
              tunnel: [FALSE w2842] -> w2832
              tunnel: [w2838 w2841] -> w2831
              tunnel: w2829 -> [w2838 w2840]
              frame "Post Process Plotted Rows" {
              }
              frame "Delete unwanted rows", Default {
                n1290 = call "Remote_call_prep.vi"("Job Directory In"=w2840) -> ("Job Directory out"=w2841:path)  [unwired: 2 in, 2 out]
                n1291 = local write "Job Directory"(w2841) -> ()
                n1292 = Not Equal?(x=w2840, y=w2841) -> (x != y?=w2842:bool)
              }
            }
            n1293 = Index Array(array=w2837, index (col)=0 ("disabled index (col)")) -> (element=w2833:i32[])  [unwired: 1 in]
            n1294 = for {
              shift-right: [w2849] -> w2834
              shift-left: i32[] [] -> [w2850]
              tunnel: w2833 -> [w2848] mode=indexing
              n1295 = Search 1D Array(1D array=w2850, element=w2848) -> (index of element=w2851:i32)  [unwired: 1 out]
              n1296 = case shown="-1" w2851 {
                tunnel: w2850 -> [w2852 w2855]
                tunnel: [w2852 w2854] -> w2849
                tunnel: w2848 -> [_ w2853]
                frame 0, Default {
                }
                frame -1 {
                  n1297 = Build Array (concatenate)(w2855, w2853) -> (w2854:i32[])
                }
              }
            }
            n1298 = case shown="True" w2832 {
              tunnel: w2831 -> [_ w2844]
              frame False {
              }
              frame True {
                n1299 = local read "Template"() -> (w2843:path)
                n1300 = Path To String(path=w2844) -> (string=w2847:string)
                n1301 = call "Read_Write_Template.vi"("Template File"=w2843, "Mode"=Global_mode."Write Global to File", "Single Value In"=w2847, "Data type"="Log Folder Name" ("Variable name")) -> ()  [unwired: 4 in, 8 out]
              }
            }
          }
          frame #2 {
            w2860 = path[] []
            n1302 = local read "Full_Res_Results_Folder"() -> (w2859:path)
            n1303 = for {
              tunnel: w2874 -> [w2896]
              tunnel: w2873 -> [w2893] mode=indexing
              tunnel: w2872 -> [w2894]
              tunnel: w2871 -> [w2892]
              tunnel: w2870 -> [w2891]
              tunnel: w2869 -> [w2890]
              tunnel: w2868 -> [w2889]
              tunnel: w2867 -> [w2888]
              tunnel: w2866 -> [w2887]
              tunnel: w2865 -> [w2886]
              tunnel: w2864 -> [w2885]
              shift-right: [w2884] -> _
              shift-left: FALSE -> [w2883]
              shift-right: [w2881] -> w2862
              shift-left: w2860 -> [w2882]
              shift-right: [w2879] -> w2861
              shift-left: w2860 -> [w2880]
              tunnel: w2859 -> [w2878]
              tunnel: w2858 -> [w2877]
              shift-right: [w2875] -> w2856
              shift-left: i32[] [] -> [w2876]
              # "Row No in file"
              # "Row No in plotter"
              n1304 = Index Array(array=w2896, index=w2893) -> (element=w2895:path)
              n1305 = stacked-sequence {
                seq-local: [w2899 _ _ _] -> [_ w2927 w2976 _]
                seq-local: [_ w2925 _ _] -> [_ _ w2975 _]
                seq-local: [w2897 _ _ _] -> [_ _ w2968 w3079]
                tunnel: w2895 -> [_ w2926 w2977 _]
                tunnel: w2894 -> [w2901 _ _ _]
                tunnel: w2893 -> [w2900 _ _ _]
                tunnel: w2892 -> [_ w2924 w2974 _]
                tunnel: w2891 -> [_ _ w2973 _]
                tunnel: w2890 -> [_ _ w2972 _]
                tunnel: w2889 -> [_ _ w2971 _]
                tunnel: w2888 -> [_ _ w2970 _]
                tunnel: w2887 -> [_ _ w2969 _]
                tunnel: w2886 -> [_ _ w2967 _]
                tunnel: w2885 -> [_ _ w2966 _]
                tunnel: [_ w2923 _ _] -> w2884
                tunnel: w2883 -> [_ w2922 _ _]
                tunnel: w2882 -> [_ _ w2965 _]
                tunnel: [_ _ w2964 _] -> w2881
                tunnel: w2880 -> [_ _ w2963 _]
                tunnel: [_ _ w2962 _] -> w2879
                tunnel: w2878 -> [_ _ w2961 _]
                tunnel: w2877 -> [_ _ w2960 _]
                tunnel: w2876 -> [_ _ _ w3080]
                tunnel: [_ _ _ w3078] -> w2875
                frame #0 {
                  w2898 = i32[] []
                  n1306 = for {
                    tunnel: w2900 -> [w2910]
                    tunnel: w2901 -> [w2906] mode=indexing
                    shift-right: [w2904] -> w2899
                    shift-left: w2898 -> [w2905]
                    shift-right: [w2903] -> w2897
                    shift-left: w2898 -> [w2902]
                    n1307 = Index Array(array=w2906, index=0) -> (element=w2908:i32)
                    n1308 = Equal?(x=w2908, y=w2910) -> (x = y?=w2907:bool)
                    n1309 = case shown="True" w2907 {
                      tunnel: w2906 -> [_ w2914]
                      tunnel: w2905 -> [w2912 w2920]
                      tunnel: [w2912 w2918] -> w2904
                      tunnel: w2902 -> [w2911 w2916]
                      tunnel: [w2911 w2917] -> w2903
                      frame False {
                      }
                      frame True {
                        n1310 = Index Array(array=w2914, index=2) -> (element=w2913:i32)
                        n1311 = Build Array (concatenate)(w2916, w2913) -> (w2917:i32[])
                        n1312 = Index Array(array=w2914, index=1) -> (element=w2919:i32)
                        n1313 = Build Array (concatenate)(w2920, w2919) -> (w2918:i32[])
                      }
                    }
                  }
                }
                frame #1 {
                  n1314 = case shown="\"Post Process Plotted Rows\"" w2924 {
                    tunnel: w2927 -> [_ _ _ _ _ w2943]
                    tunnel: w2926 -> [_ _ _ _ _ w2941]
                    tunnel: [TRUE ("T button?") TRUE ("T button?") TRUE ("T button?") TRUE ("T button?") TRUE ("T button?") w2940] -> w2925
                    tunnel: [w2928 w2930 w2932 w2934 w2936 w2939] -> w2923
                    tunnel: w2922 -> [w2928 w2930 w2932 w2934 w2936 w2938]
                    frame "Save file" {
                    }
                    frame "Edit values per row" {
                    }
                    frame "Edit Values with constants" {
                    }
                    frame "Edit Raw Data file header" {
                    }
                    frame "Post Process Plotted Rows" {
                    }
                    frame "Delete unwanted rows" {
                      n1315 = Array Size(array=w2943) -> (size(s)=w2942:i32)
                      n1316 = case shown="True" w2938 {
                        tunnel: w2942 -> [w2952 _]
                        tunnel: w2941 -> [w2951 _]
                        tunnel: [w2946 w2959] -> w2940
                        tunnel: [w2945 w2959] -> w2939
                        frame False {
                          n1317 = Format Into String(format string="Remove %d rows from \"%s\"", w2952, w2951) -> (resulting string=w2949:string)  [unwired: 2 in, 1 out]
                          n1318 = call <vilib>:"Three Button Dialog.vi"("Allow user to close window? (TRUE)"=TRUE, "Right Button Text (\"Cancel\")"="Yes To All Files" ("Right Button Text (\"Cancel\")"), "message"=w2949) -> ("Which Button?"=w2947:T10)  [unwired: 3 in, 5 out]
                          n1319 = case shown="\"Left Button\"" w2947 {
                            tunnel: [TRUE TRUE w2957 w2958] -> w2946
                            tunnel: [FALSE TRUE w2957 w2958] -> w2945
                            frame "Left Button" {
                            }
                            frame "Right Button" {
                            }
                            frame "Center Button" {
                              w2957 = FALSE
                            }
                            frame "Window Close" {
                              w2958 = FALSE
                            }
                          }
                        }
                        frame True {
                          w2959 = TRUE
                        }
                      }
                    }
                  }
                }
                frame #2 {
                  n1320 = case shown="True" w2975 {
                    tunnel: w2977 -> [_ w2996]
                    tunnel: w2976 -> [_ w2995]
                    tunnel: w2974 -> [_ w2994]
                    tunnel: w2973 -> [_ w2993]
                    tunnel: w2972 -> [_ w2992]
                    tunnel: w2971 -> [_ w2991]
                    tunnel: w2970 -> [_ w2990]
                    tunnel: w2969 -> [_ w2989]
                    tunnel: w2968 -> [_ w2988]
                    tunnel: w2967 -> [_ w2987]
                    tunnel: w2966 -> [_ w2986]
                    tunnel: w2965 -> [w2979 w2985]
                    tunnel: [w2979 w2984] -> w2964
                    tunnel: w2963 -> [w2978 w2983]
                    tunnel: [w2978 w2982] -> w2962
                    tunnel: w2961 -> [_ w2981]
                    tunnel: w2960 -> [_ w2980]
                    frame False {
                    }
                    frame True {
                      n1321 = case shown="\"Edit Raw Data file header\", Default" w2994 {
                        tunnel: w2996 -> [w3002 w3007 w3036 w3049 w3066]
                        tunnel: w2995 -> [w3005 w3018 w3035 w3048 w3065]
                        tunnel: w2993 -> [_ _ _ _ _]
                        tunnel: w2992 -> [_ _ _ w3046 w3063]
                        tunnel: w2991 -> [_ _ _ w3044 w3061]
                        tunnel: w2990 -> [_ _ _ _ w3060]
                        tunnel: w2989 -> [_ _ _ _ w3058]
                        tunnel: w2988 -> [_ _ _ _ w3057]
                        tunnel: w2987 -> [_ _ _ w3043 w3055]
                        tunnel: w2986 -> [_ _ _ w3041 w3053]
                        tunnel: w2985 -> [w3004 w3011 w3034 w3039 w3051]
                        tunnel: [w3004 w3012 w3034 w3039 w3051] -> w2984
                        tunnel: w2983 -> [w3003 w3010 w3033 w3038 w3050]
                        tunnel: [w3003 w3008 w3033 w3038 w3050] -> w2982
                        tunnel: w2981 -> [w3001 _ _ _ _]
                        tunnel: w2980 -> [_ _ _ w3037 _]
                        frame "Save file" {
                          n1322 = Strip Path(path=w3002) -> (name=w2999:string)  [unwired: 1 out]
                          n1323 = call "Add_filename_suffix.vi"("Filename"=w2999, "Suffix to add"=".xls") -> ("Filename out"=w2997:string)  [unwired: 3 out]
                          n1324 = Build Path(base path=w3001, name or relative path=w2997) -> (appended path=w3000:path)
                          n1325 = call "Save_full_Res_rows.vi"("Selected Rows"=w3005, "Filename to write"=w3000, "Filename Orig"=w3002) -> ()  [unwired: 2 out]
                        }
                        frame "Edit Raw Data file header", Default {
                          w3023 = FALSE  # Add Extra Channels?
                          w3022 = FALSE  # Read Channel Names only
                          n1326 = global read "Constants_global.vi" "Run VI Folder"() -> (w3017:path)
                          n1327 = Strip Path(path=w3017) -> (stripped path=w3016:path)  [unwired: 1 out]
                          n1328 = Build Path(base path=w3016, name or relative path="Data_plotting_vis") -> (appended path=w3015:path)
                          n1329 = Build Path(base path=w3015, name or relative path="RD_Files.tpt") -> (appended path=w3021:path)
                          n1330 = call "Read_Data_file.vi"("Results file"=w3007, "Read Channel Names only"=w3022, "Add Extra Channels?"=w3023, "Template File"=w3021) -> ("Row numbers"=w3006:i32[], "Channel Values Out"=w3024:string[][])  [unwired: 1 in, 13 out]
                          n1331 = Index Array(array=w3024, index (col)=0 ("index (row)")) -> (element=w3019:string[])  [unwired: 1 in]
                          n1332 = for {
                            tunnel: w3019 -> [w3032]
                            tunnel: w3018 -> [w3026] mode=indexing
                            tunnel: [w3030] -> w3013 mode=indexing
                            tunnel: [w3029] -> w3009 mode=indexing
                            tunnel: w3007 -> [w3029]
                            tunnel: w3006 -> [w3028]
                            n1333 = Search 1D Array(1D array=w3028, element=w3026) -> (index of element=w3027:i32)  [unwired: 1 in]
                            n1334 = Index Array(array=w3032, index=w3027) -> (element=w3031:string)
                            n1335 = call "String_to_Pathname.vi"("Input String"=w3031) -> ("path"=w3030:path)
                          }
                          n1336 = Build Array (concatenate)(w3010, w3009) -> (w3008:path[])
                          n1337 = Build Array (concatenate)(w3011, w3013) -> (w3012:path[])
                        }
                        frame "Delete unwanted rows" {
                          n1338 = call "Delete_unwanted_rows.vi"("Selected Rows"=w3035, "Filename"=w3036) -> ()  [unwired: 1 out]
                        }
                        frame "Edit Values with constants" {
                          w3047 = TRUE  # Value  Constant?
                          n1339 = local read "Edit Raw Data Header Info"() -> (w3040:bool)
                          n1340 = local read "Edit Raw DF?"() -> (w3042:bool)
                          n1341 = Not(x=w3046) -> (.not. x?=w3045:bool)
                          n1342 = call "Add_Update_Values.vi"("Filename"=w3049, "Value  Constant?"=w3047, "Edit Raw data files?"=w3042, "New Chs In"=w3044, "Edit Raw Data Header Info"=w3040, "New Values In"=w3037, "Selected Rows"=w3048, "Edit all Rows?"=w3045, "Raw DF in Orig Pos?"=w3043, "Job Directory"=w3041) -> ()  [unwired: 1 in, 5 out]
                        }
                        frame "Edit values per row" {
                          w3052 = FALSE  # Edit Raw Data Header Info
                          w3064 = FALSE  # Value  Constant?
                          n1343 = for {
                            tunnel: w3061 -> [w3077] mode=indexing
                            tunnel: w3060 -> [w3076]
                            tunnel: [w3075] -> w3059 mode=indexing
                            n1344 = Search 1D Array(1D array=w3076, element=w3077) -> (index of element=w3075:i32)  [unwired: 1 out]
                          }
                          n1345 = for {
                            tunnel: w3059 -> [w3071]
                            tunnel: w3058 -> [w3070]
                            tunnel: w3057 -> [w3068] mode=indexing
                            tunnel: [w3067] -> w3056 mode=indexing
                            n1346 = Index Array(array=w3070, index (row)=w3068) -> (element=w3069:string[])  [unwired: 1 in]
                            n1347 = for {
                              tunnel: w3071 -> [w3074] mode=indexing
                              tunnel: w3069 -> [w3073]
                              tunnel: [w3072] -> w3067 mode=indexing
                              n1348 = Index Array(array=w3073, index=w3074) -> (element=w3072:string)
                            }
                          }
                          n1349 = Not(x=w3063) -> (.not. x?=w3062:bool)
                          n1350 = local read "Edit Raw DF?"() -> (w3054:bool)
                          n1351 = call "Add_Update_Values.vi"("Filename"=w3066, "Value  Constant?"=w3064, "Edit Raw data files?"=w3054, "New Chs In"=w3061, "Edit Raw Data Header Info"=w3052, "New Values In"=w3056, "Selected Rows"=w3065, "Edit all Rows?"=w3062, "Raw DF in Orig Pos?"=w3055, "Job Directory"=w3053) -> ()  [unwired: 1 in, 5 out]
                        }
                      }
                    }
                  }
                }
                frame #3 {
                  n1352 = Build Array (concatenate)(w3080, w3079) -> (w3078:i32[])
                }
              }
            }
          }
          frame #3 {
            n1353 = case shown="\"Post Process Plotted Rows\"" w3086 {
              tunnel: ["Create Selectors" w3096 "Initialise" ("t") w3155] -> w3088
              tunnel: w3087 -> [_ _ _ w3152]
              tunnel: w3085 -> [w3089 w3095 _ _]
              tunnel: w3084 -> [_ w3094 _ _]
              tunnel: w3083 -> [_ w3093 _ _]
              tunnel: w3082 -> [_ w3092 _ _]
              tunnel: w3081 -> [_ w3091 _ _]
              frame "Edit Raw Data file header" {
                n1354 = call "Edit_Raw_DF_Header.vi"("Selected files"=w3089) -> ()  [unwired: 15 out]
              }
              frame "Post Process Plotted Rows" {
                n1355 = stacked-sequence {
                  seq-local: [w3098 _ _] -> [_ w3122 _]
                  seq-local: [w3097 _ _] -> [_ _ w3147]
                  seq-local: [_ w3119 _] -> [_ _ w3146]
                  tunnel: [_ _ "Create Selectors"] -> w3096
                  tunnel: w3095 -> [_ _ w3149]
                  tunnel: w3094 -> [_ _ w3148]
                  tunnel: w3093 -> [_ w3121 _]
                  tunnel: w3092 -> [w3099 _ _]
                  tunnel: w3091 -> [_ w3118 _]
                  frame #0 {
                    n1356 = global read "Results_plotter_Global.vi" "Dispose"() -> (w3101:string[])
                    n1357 = for {
                      tunnel: w3101 -> [w3110] mode=indexing
                      shift-right: [w3106] -> w3098
                      shift-left: i32[] [] -> [w3108]
                      i -> [w3107]
                      n1358 = String Subset(string=w3110, length (rest)=1 ("length (rest)")) -> (substring=w3112:string)  [unwired: 1 out]
                      n1359 = Equal?(x="T", y=w3112) -> (x = y?=w3109:bool)
                      n1360 = case shown="False" w3109 {
                        tunnel: w3108 -> [w3116 w3117]
                        tunnel: [w3115 w3117] -> w3106
                        tunnel: w3107 -> [w3114 _]
                        frame False {
                          n1361 = Build Array (concatenate)(w3116, w3114) -> (w3115:i32[])
                        }
                        frame True {
                        }
                      }
                    }
                    n1362 = for {
                      tunnel: w3099 -> [w3105]
                      tunnel: w3098 -> [w3104] mode=indexing
                      tunnel: [w3103] -> w3097 mode=indexing
                      n1363 = Index Array(array=w3105, index=w3104) -> (element=w3103:string)
                    }
                    n1364 = local write "Post Process Plotted Data"(FALSE ("Post Process Plotted Data")) -> ()
                  }
                  frame #1 {
                    n1365 = global read "Results_plotter_Global.vi" "Precision"() -> (w3120:string[])
                    n1366 = for {
                      tunnel: w3122 -> [w3128]
                      tunnel: w3121 -> [w3124]
                      tunnel: w3120 -> [w3127]
                      tunnel: [w3126] -> w3119 mode=indexing
                      tunnel: w3118 -> [w3125] mode=indexing
                      n1367 = Index Array(array=w3124, index (row)=w3125) -> (element=w3123:string[])  [unwired: 1 in]
                      n1368 = for {
                        tunnel: w3128 -> [w3138] mode=indexing
                        tunnel: w3123 -> [w3140]
                        tunnel: w3127 -> [w3139]
                        tunnel: [w3132] -> w3126 mode=indexing
                        n1369 = Index Array(array=w3140, index=w3138) -> (element=w3131:string)
                        n1370 = Index Array(array=w3139, index=w3138) -> (element=w3130:string)
                        n1371 = Fract/Exp String To Number(string=w3131) -> (offset past number=w3136:i32, number=w3133:dbl)  [unwired: 3 out]
                        n1372 = String Length(string=w3131) -> (length=w3137:i32)
                        n1373 = Equal?(x=w3137, y=w3136) -> (x = y?=w3134:bool)
                        n1374 = Empty String/Path?(string/path=w3131) -> (empty?=w3135:bool)
                        n1375 = Compound Arithmetic op=AND(invert w3135, w3134) -> (w3129:bool)
                        n1376 = case shown="True" w3129 {
                          tunnel: w3130 -> [_ w3143]
                          tunnel: w3133 -> [_ w3144]
                          tunnel: [w3141 w3142] -> w3132
                          tunnel: w3131 -> [w3141 _]
                          frame False {
                          }
                          frame True {
                            n1377 = call "Number_2_string.vi"("precision"=w3143, "number"=w3144) -> ("String"=w3142:string)
                          }
                        }
                      }
                    }
                  }
                  frame #2 {
                    n1378 = Build Array (concatenate)(w3147, w3146) -> (w3145:string[][])
                    n1379 = call "Post_Process_Profile_Remote.vi"("Results Plotter Rows"=w3145, "Raw Data files to PP"=w3149, "Current Results filenames"=w3148) -> ()  [unwired: 1 out]
                  }
                }
              }
              frame "Delete unwanted rows" {
              }
              frame "Edit Values with constants", Default {
                n1380 = local read "No Of Rows"() -> (w3154:i32)
                n1381 = Less?(x=w3154, y=w3152) -> (x < y?=w3153:bool)
                n1382 = case shown="False" w3153 {
                  tunnel: ["Create Selectors" "Initialise" ("t")] -> w3155
                  frame False {
                  }
                  frame True {
                  }
                }
              }
            }
          }
          frame #4 {
            n1383 = Current VI's Path() -> (path=w3158:path)
            n1384 = call "Bring_to_front.vi"("path"=w3158) -> ()
          }
        }
      }
      frame "End" {
        n1385 = local read "Template"() -> (w3160:path)
        n1386 = local read "Empty"() -> (w3161:bool)
        n1387 = call "Valid_Path.vi"("Filename"=w3160) -> ("Valid Path?"=w3159:bool)
        n1388 = case shown="True" w3161 {
          frame False {
          }
          frame True {
            n1389 = property on="Result files to read" class="Arr (strict)"("Index Values"=u32[] [0] ("Write Attribute")) -> ()  [unwired: 2 in, 2 out]
            n1390 = local write "Result files to read"(path[] [] ("Result files to read")) -> ()
            n1391 = local write "Empty"(FALSE ("Empty")) -> ()
          }
        }
        n1392 = case shown="False" w3159 {
          tunnel: w3162 -> [w3171 _]
          frame False {
            n1393 = local write "Template"(w3171) -> ()
          }
          frame True {
          }
        }
      }
      frame "Empty Results file array" {
        n1394 = local read "Template"() -> (w3173:path)
        n1395 = call "Valid_Path.vi"("Filename"=w3173) -> ("Valid Path?"=w3172:bool)
        n1396 = case shown="True" w3172 {
          tunnel: w3174 -> [w3183 _]
          frame False {
            n1397 = local write "Template"(w3183) -> ()
          }
          frame True {
          }
        }
        n1398 = property on="Result files to read" class="Arr (strict)"("Index Values"=u32[] [0] ("Write Attribute")) -> ()  [unwired: 2 in, 2 out]
        n1399 = local write "Result files to read"(path[] [] ("Result files to read")) -> ()
        n1400 = local write "Empty"(FALSE ("Empty")) -> ()
      }
      frame "Save Setup" {
        w3188 = "Current_Setup.xls" ("Setup filename")
        n1401 = local read "Create picture Vi Name"() -> (w3203:string)
        n1402 = local read "Additional X Values"() -> (w3209:dbl[])
        n1403 = local read "Additional Y Values"() -> (w3208:dbl[])
        n1404 = local read "Result files to read"() -> (w3211:path[])
        n1405 = local read "Output Filename"() -> (w3204:path)
        n1406 = local read "Intensity Plot?"() -> (w3202:bool)
        n1407 = local read "Multi Ordinate?"() -> (w3201:bool)
        n1408 = local read "Multi Ordinate"() -> (w3197:i32[])
        n1409 = local read "Filter Array"() -> (w3205:u16[])
        n1410 = local read "Transpose"() -> (w3210:bool)
        n1411 = local read "Template"() -> (w3189:path)
        n1412 = local read "Filter Bins 2"() -> (w3198:i32[])
        n1413 = local read "Ordinate"() -> (w3207:u16)
        n1414 = local read "Filter Bins 1"() -> (w3199:i32[])
        n1415 = local read "Absisca"() -> (w3206:u16)
        n1416 = call "Read_Write_Plot_Setup.vi"("Mode"=enum16{"Load", "Save"}."Load", "Setup filename"=w3188) -> ("Cluster 2"=w3212:T9)  [unwired: 1 in, 1 out]
        n1417 = Bundle By Name(cluster=w3212, "Result files to read"=w3211, "Template"=w3189, "Transpose"=w3210, "Additional X Values"=w3209, "Additional Y Values"=w3208, "Ordinate"=w3207, "Absisca"=w3206, "Filter Array"=w3205, "color and symbol"=TRUE, "Output Filename"=w3204, "Jpg Vi Name"=w3203, "Intensity Plot?"=w3202, "Multi Ordinate?"=w3201, "Filter Bins 1"=w3199, "Filter Bins 2"=w3198, "Multi Ordinate"=w3197) -> (w3200:T9)
        n1418 = local read "Save Setup"() -> (w3187:bool)
        n1419 = local read "stop"() -> (w3195:bool)
        n1420 = Not(x=w3195) -> (.not. x?=w3194:bool)
        n1421 = Path To String(path="Job Directory") -> (string=w3193:string)
        n1422 = call "Read_Write_Plot_Setup.vi"("Mode"=enum16{"Load", "Save"}."Save", "Setup filename"=w3188, "Cluster"=w3200) -> ()  [unwired: 2 out]
        n1423 = call "Read_Write_Template.vi"("Template File"=w3189, "Mode"=Global_mode."Write Global to File", "Single Value In"=w3193, "Data type"="Log Folder Name" ("Variable name")) -> ()  [unwired: 4 in, 8 out]
        n1424 = Select(t="Save to named setup file", s=w3187, f="Check modification dates?") -> (s? t:f=w3185:string)
      }
      frame "Save to named setup file" {
        w3218 = TRUE  # Save New File?
        n1425 = global read "Constants_global.vi" "Results file plotter folder"() -> (w3220:path)
        n1426 = call "Save_current_setup.vi"("Save New File?"=w3218, "Folder"=w3220) -> ()  [unwired: 4 out]
        n1427 = local write "Save Setup"(FALSE ("Save Setup")) -> ()
      }
    }
    "Current" <- w11
  }
